vi "CRYO_MASTER_FULL.vi"() -> ()   [LabVIEW 2017]
uses:
  LSI218Data.lvclass
  LSI336Data.lvclass
  USBData.lvclass
  6240AData.lvclass
  <vilib>/DAQmx/create/channels.llb/DAQmx Create Channel (DO-Digital Output).vi
  <vilib>/DAQmx/miscellaneous.llb/DAQmx Fill In Error Info.vi
  <vilib>/DAQmx/create/channels.llb/DAQmx Create Channel (AO-Voltage-Basic).vi
  <vilib>/express/express arith-compare/Formula/XNode/ExpressFormulaBlockNode.xnode
  <vilib>/Analysis/NI_AALBase.lvlib
panel:
  in  "Frontpanel screenshots":bool
  in  "Screenshots interval":i64=3605
  in  "Record interval":i64=10
  out "Cycle #":u32=332
  in  "Measurement Interval (s)":dbl=1.0
  in  "Stop Button":bool
  in  "?":T1(tab)=enum."(Place holder)"
  in  "Base Path (screenshots)":path=path "C:/LabVIEW/DATA/Precooling"
  out "error out (USB6210/6218 AOUT)":errorcluster
  in  "AOUT 1 Label":string="KIKUSUI_I"
  in  "AOUT 0 Label":string="KIKUSUI_V"
  in  "DOUT Labels":string[](array[string])=["D_V1_NO", "D_V2_NC", "D_CV1"]
  in  "AOUT for Current CTRL":tag="Dev1/ao1"
  in  "AOUT For Voltage CTRL":tag="Dev1/ao0"
  out "AO task out":refnum<k21>="20200912_112449_AO"
  in  "Analog Out ON?":bool=TRUE
  in  "InstName (USB6218)":string="USB6218"
  in  "USB6218 Config":T2(array[cluster])=[{"Label"="F_1", "FileFormat"="%5.5f", "Active?"=TRUE, "Physical CH"="Dev1/ai0", " terminal\n type"=10083, "ConversionType"={"Type"=enum."SimpleProp", "ConversionParameters"=[0.0, 5.0, 0.0, 500.0]}, "VoltageLimits"=[0.0, 5.0]}, {"Label"="F_2", "FileFormat"="%5.5f", "Active?"=TRUE, "Physical CH"="Dev1/ai1", " terminal\n type"=10083, "ConversionType"={"Type"=enum."SimpleProp", "ConversionParameters"=[0.0, 5.0, 0.0, 200.0]}, "VoltageLimits"=[0.0, 5.0]}, {"Label"="F_3", "FileFormat"="%5.5f", "Active?"=TRUE, "Physical CH"="Dev1/ai2", " terminal\n type"=10083, "ConversionType"={"Type"=enum."SimpleProp", "ConversionParameters"=[0.0, 5.0, 0.0, 200.0]}, "VoltageLimits"=[0.0, 5.0]}, {"Label"="F_4", "FileFormat"="%5.5f", "Active?"=TRUE, "Physical CH"="Dev1/ai3", " terminal\n type"=10083, "ConversionType"={"Type"=enum."SimpleProp", "ConversionParameters"=[0.0, 5.0, 0.0, 500.0]}, "VoltageLimits"=[0.0, 5.0]}, {"Label"="F_5", "FileFormat"="%5.5f", "Active?"=TRUE, "Physical CH"="Dev1/ai4", " terminal\n type"=10083, "ConversionType"={"Type"=enum."SimpleProp", "ConversionParameters"=[0.0, 5.0, 0.0, 500.0]}, "VoltageLimits"=[0.0, 5.0]}, {"Label"="I_CV", "FileFormat"="%3.5f", "Active?"=TRUE, "Physical CH"="Dev1/ai5", " terminal\n type"=10083, "ConversionType"={"Type"=enum."SimpleProp", "ConversionParameters"=[0.0, 10.0, 0.0, 2000.0]}, "VoltageLimits"=[0.0, 10.0]}, {"Label"="CV1_answer", "FileFormat"="%3.5f", "Active?"=TRUE, "Physical CH"="Dev1/ai6", " terminal\n type"=10083, "ConversionType"={"Type"=enum."SimpleProp", "ConversionParameters"=[1.0, 5.0, 0.0, 100.0]}, "VoltageLimits"=[0.0, 5.0]}] {"terminal\n type" items=["Default"=-1, "RSE"=10083, "NRSE"=10078, "Differential"=10106, "Pseudodifferential"=12529]}
  out "error out (USB6218)":errorcluster
  out "error out (USB6210/6218 DOUT)":errorcluster
  out "DOUT task out":refnum<k21>="20200912_112449_DO"
  in  "DOUT Physical CH":tag[](array[tag])=["Dev1/port1/line0", "Dev1/port1/line1", "Dev1/port1/line2"]
  in  "Digital Out ON?":bool=TRUE
  in  "USB6210 Config":T2(array[cluster])=[{"Label"="P_ins", "FileFormat"="%5.5e", "Active?"=TRUE, "Physical CH"="Dev2/ai0", " terminal\n type"=10083, "ConversionType"={"Type"=enum."CC-10_LOG", "ConversionParameters"=[0.5, 9.0, 0.0, 1.0]}, "VoltageLimits"=[0.0, 10.0]}, {"Label"="P_4Kres", "FileFormat"="%5.5e", "Active?"=TRUE, "Physical CH"="Dev2/ai1", " terminal\n type"=10083, "ConversionType"={"Type"=enum."SimpleProp", "ConversionParameters"=[1.0, 5.0, 0.0, 200000.0]}, "VoltageLimits"=[0.0, 5.0]}, {"Label"="P_3HeIN", "FileFormat"="%5.5e", "Active?"=TRUE, "Physical CH"="Dev2/ai2", " terminal\n type"=10083, "ConversionType"={"Type"=enum."SimpleProp", "ConversionParameters"=[1.0, 5.0, 0.0, 200000.0]}, "VoltageLimits"=[0.0, 5.0]}, {"Label"="P_SldRTN", "FileFormat"="%5.5e", "Active?"=TRUE, "Physical CH"="Dev2/ai3", " terminal\n type"=10083, "ConversionType"={"Type"=enum."SimpleProp", "ConversionParameters"=[1.0, 5.0, 0.0, 200000.0]}, "VoltageLimits"=[0.0, 5.0]}, {"Label"="P_3Hepot", "FileFormat"="%5.5e", "Active?"=TRUE, "Physical CH"="Dev2/ai4", " terminal\n type"=10083, "ConversionType"={"Type"=enum."SimpleProp", "ConversionParameters"=[0.0, 10.0, 0.0, 133320.0]}, "VoltageLimits"=[0.0, 10.0]}, {"Label"="P_1Kpot", "FileFormat"="%5.5e", "Active?"=TRUE, "Physical CH"="Dev2/ai5", " terminal\n type"=10083, "ConversionType"={"Type"=enum."SimpleProp", "ConversionParameters"=[0.0, 10.0, 0.0, 133320.0]}, "VoltageLimits"=[0.0, 10.0]}, {"Label"="P_Dewar", "FileFormat"="%5.5e", "Active?"=TRUE, "Physical CH"="Dev2/ai6", " terminal\n type"=10083, "ConversionType"={"Type"=enum."SimpleProp", "ConversionParameters"=[1.0, 5.0, 0.0, 200000.0]}, "VoltageLimits"=[0.0, 5.0]}, {"Label"="DP_HEX4", "FileFormat"="%5.5e", "Active?"=TRUE, "Physical CH"="Dev2/ai7", " terminal\n type"=10083, "ConversionType"={"Type"=enum."SimpleProp", "ConversionParameters"=[1.0, 5.0, 0.0, 1000.0]}, "VoltageLimits"=[0.0, 5.0]}, {"Label"="DP_HEX5", "FileFormat"="%5.5e", "Active?"=TRUE, "Physical CH"="Dev2/ai8", " terminal\n type"=10083, "ConversionType"={"Type"=enum."SimpleProp", "ConversionParameters"=[1.0, 5.0, 0.0, 20000.0]}, "VoltageLimits"=[0.0, 5.0]}, {"Label"="L1", "FileFormat"="%5.5f", "Active?"=TRUE, "Physical CH"="Dev2/ai9", " terminal\n type"=10083, "ConversionType"={"Type"=enum."SimpleProp", "ConversionParameters"=[0.0, 10.0, 0.0, 100.0]}, "VoltageLimits"=[0.0, 10.0]}, {"Label"="L2-1", "FileFormat"="%5.5f", "Active?"=TRUE, "Physical CH"="Dev2/ai10", " terminal\n type"=10083, "ConversionType"={"Type"=enum."SimpleProp", "ConversionParameters"=[0.0, 10.0, 0.0, 100.0]}, "VoltageLimits"=[0.0, 10.0]}, {"Label"="L2-2", "FileFormat"="%5.5f", "Active?"=TRUE, "Physical CH"="Dev2/ai11", " terminal\n type"=10083, "ConversionType"={"Type"=enum."SimpleProp", "ConversionParameters"=[0.0, 10.0, 0.0, 100.0]}, "VoltageLimits"=[0.0, 10.0]}, {"Label"="L3", "FileFormat"="%5.5f", "Active?"=TRUE, "Physical CH"="Dev2/ai12", " terminal\n type"=10083, "ConversionType"={"Type"=enum."SimpleProp", "ConversionParameters"=[0.0, 10.0, 0.0, 100.0]}, "VoltageLimits"=[0.0, 10.0]}] {"terminal\n type" items=["Default"=-1, "RSE"=10083, "NRSE"=10078, "Differential"=10106, "Pseudodifferential"=12529]}
  in  "RUN identifier":string="PreCooling"
  in  "Base Path":path=path "C:/LabVIEW/DATA/Precooling"
  in  "InstName (USB6210)":string="USB6210"
  out "error out (USB6210)":errorcluster
  out "File Refn USB AO":refnum<file>
  out "File Refn USB DO":refnum<file>
  out "error out (LSI336)":errorcluster
  in  "InstName (LSI336)":string="LSI336"
  in  "FileFormat (336)":string="%4.4f"
  in  "LSI336Settings(X,Y)":T3(array[cluster])=[{"LSIName"="LSi336X", "Labels"=["T1K3-1", "T1K3-2", "T3He5", "T3He8"], "SensorLocations"=[enum."T1K3-1", enum."T1K3-2", enum."T3He5", enum."T3He8"], "Active?"=TRUE, "VISA res. name"="GPIB0::6::INSTR"}, {"LSIName"="LSi336Y", "Labels"=["T3He6-1", "T3He6-2", "T3He7-1", "T3He7-2"], "SensorLocations"=[enum."T3He6-1", enum."T3He6-2", enum."T3He7-1", enum."T3He7-2"], "Active?"=TRUE, "VISA res. name"="GPIB0::2::INSTR"}]
  in  "FileFormat (218)":string="%4.4f"
  in  "InstName (LSI218)":string="LSI218"
  in  "LSI218Settings(A-F)":T3(array[cluster])=[{"LSIName"="LSI218A", "Labels"=["T3He10", "T3He1-1", "TTH3", "TTH4", "TTH1", "TTH2", "T4He1", "T1K1"], "SensorLocations"=[enum."T3He10", enum."T3He1-1", enum."TTH3", enum."TTH4", enum."TTH1", enum."TTH2", enum."T4He1", enum."T1K1"], "Active?"=TRUE, "VISA res. name"="GPIB0::7::INSTR"}, {"LSIName"="LSI218B", "Labels"=["N.C.", "N.C.", "N.C.", "N.C.", "T3He2-1", "T3He2-2", "T3He3", "T3He1-4"], "SensorLocations"=[enum."N.C.", enum."N.C.", enum."N.C.", enum."N.C.", enum."T3He2-1", enum."T3He2-2", enum."T3He3", enum."T3He1-4"], "Active?"=TRUE, "VISA res. name"="GPIB0::4::INSTR"}, {"LSIName"="LSI218C", "Labels"=["T4He3-1", "T4He3-2", "T4He3-3", "T4He3-4", "T4He2-1", "T4He2-2", "T4He4", "T4He5"], "SensorLocations"=[enum."T4He3-1", enum."T4He3-2", enum."T4He3-3", enum."T4He3-4", enum."T4He2-1", enum."T4He2-2", enum."T4He4", enum."T4He5"], "Active?"=TRUE, "VISA res. name"="GPIB0::3::INSTR"}, {"LSIName"="LSI218D", "Labels"=["T4He6", "T4He9", "T3He1-2", "T3He1-3", "T4He7", "T4He8", "T4He10", "T1K6"], "SensorLocations"=[enum."T4He6", enum."T4He9", enum."T3He1-2", enum."T3He1-3", enum."T4He7", enum."T4He8", enum."T4He10", enum."T1K6"], "Active?"=TRUE, "VISA res. name"="GPIB0::5::INSTR"}, {"LSIName"="LSI218E", "Labels"=["TIP1", "N.C.", "TIP2", "N.C.", "TIP3", "TIP4", "TIP5", "N.C."], "SensorLocations"=[enum."TIP1", enum."N.C.", enum."TIP2", enum."N.C.", enum."TIP3", enum."TIP4", enum."TIP5", enum."N.C."], "Active?"=TRUE, "VISA res. name"="GPIB0::11::INSTR"}, {"LSIName"="LSI218F", "Labels"=["T1K2", "T1K4", "T1K5", "T3He4", "T3He9", "TIP6", "N.C.", "N.C."], "SensorLocations"=[enum."T1K2", enum."T1K4", enum."T1K5", enum."T3He4", enum."T3He9", enum."TIP6", enum."N.C.", enum."N.C."], "Active?"=TRUE, "VISA res. name"="GPIB0::8::INSTR"}]
  out "error out (LSI218)":errorcluster
  out "Graph 3":T4(graph) caption="XY Graph"
  out "Graph 1":T4(graph)=[{"TimeArray"=[timestamp(3682722291.26542 s since 1904-01-01), timestamp(3682722291.60303 s since 1904-01-01), timestamp(3682722291.9037905 s since 1904-01-01), timestamp(3682722292.2130303 s since 1904-01-01), timestamp(3682722293.6093 s since 1904-01-01), timestamp(3682722293.911434 s since 1904-01-01), timestamp(3682722294.215163 s since 1904-01-01), timestamp(3682722294.522572 s since 1904-01-01), timestamp(3682722294.8441634 s since 1904-01-01), timestamp(3682722295.1448545 s since 1904-01-01), timestamp(3682722295.44568 s since 1904-01-01), timestamp(3682722295.7512665 s since 1904-01-01), timestamp(3682722296.071016 s since 1904-01-01), timestamp(3682722297.4895544 s since 1904-01-01), timestamp(3682722298.3582816 s since 1904-01-01), timestamp(3682722298.6583776 s since 1904-01-01), timestamp(3682722298.976703 s since 1904-01-01), timestamp(3682722299.303491 s since 1904-01-01), timestamp(3682722299.6028943 s since 1904-01-01), timestamp(3682722299.9109864 s since 1904-01-01), timestamp(3682722301.2943215 s since 1904-01-01), timestamp(3682722302.439338 s since 1904-01-01), timestamp(3682722302.84283 s since 1904-01-01), timestamp(3682722303.976296 s since 1904-01-01), timestamp(3682722304.298886 s since 1904-01-01), timestamp(3682722304.6146727 s since 1904-01-01), timestamp(3682722304.9304714 s since 1904-01-01), timestamp(3682722306.0827866 s since 1904-01-01), timestamp(3682722306.400269 s since 1904-01-01), timestamp(3682722306.701908 s since 1904-01-01), timestamp(3682722307.01266 s since 1904-01-01), timestamp(3682722307.3139567 s since 1904-01-01), timestamp(3682722307.617281 s since 1904-01-01), timestamp(3682722307.9324656 s since 1904-01-01), timestamp(3682722308.2477794 s since 1904-01-01), timestamp(3682722309.066163 s since 1904-01-01), timestamp(3682722309.3965664 s since 1904-01-01), timestamp(3682722309.7003713 s since 1904-01-01), timestamp(3682722310.0011826 s since 1904-01-01), timestamp(3682722310.3316903 s since 1904-01-01), timestamp(3682722310.6338625 s since 1904-01-01), timestamp(3682722311.8390217 s since 1904-01-01), timestamp(3682722312.147876 s since 1904-01-01), timestamp(3682722312.4494967 s since 1904-01-01), timestamp(3682722312.760971 s since 1904-01-01), timestamp(3682722313.065274 s since 1904-01-01), timestamp(3682722313.3656464 s since 1904-01-01), timestamp(3682722313.6989264 s since 1904-01-01), timestamp(3682722314.00116 s since 1904-01-01), timestamp(3682722314.3316183 s since 1904-01-01), timestamp(3682722314.632463 s since 1904-01-01), timestamp(3682722314.9485526 s since 1904-01-01), timestamp(3682722315.2606983 s since 1904-01-01), timestamp(3682722315.5799346 s since 1904-01-01), timestamp(3682722315.9180913 s since 1904-01-01), timestamp(3682722316.2203927 s since 1904-01-01), timestamp(3682722316.5203104 s since 1904-01-01), timestamp(3682722316.8202634 s since 1904-01-01), timestamp(3682722318.055342 s since 1904-01-01), timestamp(3682722318.3566217 s since 1904-01-01), timestamp(3682722318.67011 s since 1904-01-01), timestamp(3682722318.979581 s since 1904-01-01), timestamp(3682722319.3166094 s since 1904-01-01), timestamp(3682722319.6308255 s since 1904-01-01), timestamp(3682722319.948837 s since 1904-01-01), timestamp(3682722320.2572136 s since 1904-01-01), timestamp(3682722320.599373 s since 1904-01-01), timestamp(3682722320.919993 s since 1904-01-01), timestamp(3682722321.220749 s since 1904-01-01), timestamp(3682722321.5287714 s since 1904-01-01), timestamp(3682722321.8486905 s since 1904-01-01), timestamp(3682722322.1527696 s since 1904-01-01), timestamp(3682722322.4684625 s since 1904-01-01), timestamp(3682722322.768717 s since 1904-01-01), timestamp(3682722323.0695057 s since 1904-01-01), timestamp(3682722323.3691983 s since 1904-01-01), timestamp(3682722323.699779 s since 1904-01-01), timestamp(3682722324.00254 s since 1904-01-01), timestamp(3682722324.302169 s since 1904-01-01), timestamp(3682722324.6159334 s since 1904-01-01), timestamp(3682722324.9335217 s since 1904-01-01), timestamp(3682722325.2332306 s since 1904-01-01), timestamp(3682722325.5330367 s since 1904-01-01), timestamp(3682722325.833967 s since 1904-01-01), timestamp(3682722326.1509953 s since 1904-01-01), timestamp(3682722326.4644866 s since 1904-01-01), timestamp(3682722326.767284 s since 1904-01-01), timestamp(3682722327.067716 s since 1904-01-01), timestamp(3682722327.3710494 s since 1904-01-01), timestamp(3682722327.6760697 s since 1904-01-01), timestamp(3682722328.0013742 s since 1904-01-01), timestamp(3682722328.3049417 s since 1904-01-01), timestamp(3682722328.605616 s since 1904-01-01), timestamp(3682722328.915824 s since 1904-01-01), timestamp(3682722329.2197704 s since 1904-01-01), timestamp(3682722329.533479 s since 1904-01-01), timestamp(3682722329.8484006 s since 1904-01-01), timestamp(3682722330.1537294 s since 1904-01-01), timestamp(3682722330.4685154 s since 1904-01-01), timestamp(3682722330.7689 s since 1904-01-01), timestamp(3682722331.0704536 s since 1904-01-01), timestamp(3682722331.371037 s since 1904-01-01), timestamp(3682722331.701168 s since 1904-01-01), timestamp(3682722332.003296 s since 1904-01-01), timestamp(3682722332.3189206 s since 1904-01-01), timestamp(3682722332.6204143 s since 1904-01-01), timestamp(3682722332.9201455 s since 1904-01-01), timestamp(3682722333.222704 s since 1904-01-01), timestamp(3682722333.5307713 s since 1904-01-01), timestamp(3682722333.850218 s since 1904-01-01), timestamp(3682722334.1687818 s since 1904-01-01), timestamp(3682722334.50168 s since 1904-01-01), timestamp(3682722334.8162985 s since 1904-01-01), timestamp(3682722335.1198063 s since 1904-01-01), timestamp(3682722335.433464 s since 1904-01-01), timestamp(3682722335.754174 s since 1904-01-01), timestamp(3682722336.065685 s since 1904-01-01), timestamp(3682722336.3676305 s since 1904-01-01), timestamp(3682722336.678262 s since 1904-01-01), timestamp(3682722337.00354 s since 1904-01-01), timestamp(3682722337.305712 s since 1904-01-01), timestamp(3682722337.6067743 s since 1904-01-01), timestamp(3682722337.906976 s since 1904-01-01), timestamp(3682722338.207723 s since 1904-01-01), timestamp(3682722338.5086007 s since 1904-01-01), timestamp(3682722338.8327622 s since 1904-01-01), timestamp(3682722339.15376 s since 1904-01-01), timestamp(3682722339.4660926 s since 1904-01-01), timestamp(3682722339.7669024 s since 1904-01-01), timestamp(3682722340.0687447 s since 1904-01-01), timestamp(3682722340.3689446 s since 1904-01-01), timestamp(3682722340.669699 s since 1904-01-01), timestamp(3682722340.971668 s since 1904-01-01), timestamp(3682722341.2735777 s since 1904-01-01), timestamp(3682722341.5808673 s since 1904-01-01), timestamp(3682722341.9035897 s since 1904-01-01), timestamp(3682722342.2187233 s since 1904-01-01), timestamp(3682722342.519108 s since 1904-01-01), timestamp(3682722342.8346863 s since 1904-01-01), timestamp(3682722343.148861 s since 1904-01-01), timestamp(3682722343.453436 s since 1904-01-01), timestamp(3682722343.7687 s since 1904-01-01), timestamp(3682722344.0703554 s since 1904-01-01), timestamp(3682722344.3702574 s since 1904-01-01), timestamp(3682722344.6709967 s since 1904-01-01), timestamp(3682722345.753763 s since 1904-01-01), timestamp(3682722346.088916 s since 1904-01-01), timestamp(3682722346.411592 s since 1904-01-01), timestamp(3682722346.713475 s since 1904-01-01), timestamp(3682722347.054868 s since 1904-01-01), timestamp(3682722347.366645 s since 1904-01-01), timestamp(3682722347.6674814 s since 1904-01-01), timestamp(3682722348.1936336 s since 1904-01-01), timestamp(3682722348.7083697 s since 1904-01-01), timestamp(3682722349.007952 s since 1904-01-01), timestamp(3682722349.320494 s since 1904-01-01), timestamp(3682722349.6215 s since 1904-01-01), timestamp(3682722349.921623 s since 1904-01-01), timestamp(3682722350.2236137 s since 1904-01-01), timestamp(3682722350.525284 s since 1904-01-01), timestamp(3682722350.8256655 s since 1904-01-01), timestamp(3682722351.126511 s since 1904-01-01), timestamp(3682722351.434491 s since 1904-01-01), timestamp(3682722351.75064 s since 1904-01-01), timestamp(3682722352.0507593 s since 1904-01-01), timestamp(3682722352.3531384 s since 1904-01-01), timestamp(3682722352.6707296 s since 1904-01-01), timestamp(3682722352.9734945 s since 1904-01-01), timestamp(3682722353.2847114 s since 1904-01-01), timestamp(3682722353.600667 s since 1904-01-01), timestamp(3682722353.906944 s since 1904-01-01), timestamp(3682722354.206764 s since 1904-01-01), timestamp(3682722354.518809 s since 1904-01-01), timestamp(3682722354.8189607 s since 1904-01-01), timestamp(3682722355.138008 s since 1904-01-01), timestamp(3682722355.4524865 s since 1904-01-01), timestamp(3682722355.7545385 s since 1904-01-01), timestamp(3682722356.0694222 s since 1904-01-01), timestamp(3682722356.371631 s since 1904-01-01), timestamp(3682722356.671609 s since 1904-01-01), timestamp(3682722356.972576 s since 1904-01-01), timestamp(3682722357.2745256 s since 1904-01-01), timestamp(3682722357.5746017 s since 1904-01-01), timestamp(3682722357.9027176 s since 1904-01-01), timestamp(3682722358.220368 s since 1904-01-01), timestamp(3682722358.536658 s since 1904-01-01), timestamp(3682722358.8382 s since 1904-01-01), timestamp(3682722359.139381 s since 1904-01-01), timestamp(3682722359.4571586 s since 1904-01-01), timestamp(3682722359.7668686 s since 1904-01-01), timestamp(3682722360.068324 s since 1904-01-01), timestamp(3682722360.3683295 s since 1904-01-01), timestamp(3682722361.6878138 s since 1904-01-01), timestamp(3682722363.114297 s since 1904-01-01), timestamp(3682722363.413959 s since 1904-01-01), timestamp(3682722363.7199144 s since 1904-01-01), timestamp(3682722364.037248 s since 1904-01-01), timestamp(3682722364.3384633 s since 1904-01-01), timestamp(3682722364.6368146 s since 1904-01-01), timestamp(3682722364.936756 s since 1904-01-01), timestamp(3682722365.3525553 s since 1904-01-01), timestamp(3682722365.6523194 s since 1904-01-01), timestamp(3682722365.953843 s since 1904-01-01), timestamp(3682722366.259619 s since 1904-01-01), timestamp(3682722366.5631113 s since 1904-01-01), timestamp(3682722366.868568 s since 1904-01-01), timestamp(3682722367.202246 s since 1904-01-01), timestamp(3682722367.518932 s since 1904-01-01), timestamp(3682722367.835234 s since 1904-01-01), timestamp(3682722368.151437 s since 1904-01-01), timestamp(3682722368.455229 s since 1904-01-01), timestamp(3682722368.7568297 s since 1904-01-01), timestamp(3682722369.070481 s since 1904-01-01), timestamp(3682722369.3724856 s since 1904-01-01), timestamp(3682722369.674691 s since 1904-01-01), timestamp(3682722369.9750576 s since 1904-01-01), timestamp(3682722370.2769585 s since 1904-01-01), timestamp(3682722370.5767703 s since 1904-01-01), timestamp(3682722371.761378 s since 1904-01-01), timestamp(3682722372.0615153 s since 1904-01-01), timestamp(3682722372.36768 s since 1904-01-01), timestamp(3682722372.6716857 s since 1904-01-01), timestamp(3682722372.9741178 s since 1904-01-01), timestamp(3682722373.2752647 s since 1904-01-01), timestamp(3682722373.5791826 s since 1904-01-01), timestamp(3682722373.8855314 s since 1904-01-01), timestamp(3682722374.2075486 s since 1904-01-01), timestamp(3682722374.5190463 s since 1904-01-01), timestamp(3682722374.822685 s since 1904-01-01), timestamp(3682722375.135455 s since 1904-01-01), timestamp(3682722375.4391584 s since 1904-01-01), timestamp(3682722375.753536 s since 1904-01-01), timestamp(3682722376.0574703 s since 1904-01-01), timestamp(3682722376.3707743 s since 1904-01-01), timestamp(3682722376.671406 s since 1904-01-01), timestamp(3682722376.973929 s since 1904-01-01), timestamp(3682722377.275672 s since 1904-01-01), timestamp(3682722377.903696 s since 1904-01-01), timestamp(3682722378.3413343 s since 1904-01-01), timestamp(3682722378.6628866 s since 1904-01-01), timestamp(3682722378.971062 s since 1904-01-01), timestamp(3682722379.272179 s since 1904-01-01), timestamp(3682722379.574565 s since 1904-01-01), timestamp(3682722379.8750696 s since 1904-01-01), timestamp(3682722380.1758666 s since 1904-01-01), timestamp(3682722380.4776945 s since 1904-01-01), timestamp(3682722380.785676 s since 1904-01-01), timestamp(3682722381.101816 s since 1904-01-01), timestamp(3682722382.102351 s since 1904-01-01), timestamp(3682722383.1034727 s since 1904-01-01), timestamp(3682722384.1039815 s since 1904-01-01), timestamp(3682722385.1047606 s since 1904-01-01), timestamp(3682722386.103784 s since 1904-01-01), timestamp(3682722387.1065063 s since 1904-01-01), timestamp(3682722388.105764 s since 1904-01-01), timestamp(3682722389.1080866 s since 1904-01-01), timestamp(3682722392.018273 s since 1904-01-01), timestamp(3682722393.0827537 s since 1904-01-01), timestamp(3682722394.4643016 s since 1904-01-01), timestamp(3682722395.465176 s since 1904-01-01), timestamp(3682722396.4664454 s since 1904-01-01), timestamp(3682722398.0099154 s since 1904-01-01), timestamp(3682722399.010983 s since 1904-01-01), timestamp(3682722400.0118704 s since 1904-01-01), timestamp(3682722401.013437 s since 1904-01-01), timestamp(3682722402.015486 s since 1904-01-01), timestamp(3682722403.0175056 s since 1904-01-01), timestamp(3682722404.01802 s since 1904-01-01), timestamp(3682722405.0194936 s since 1904-01-01), timestamp(3682722406.0196953 s since 1904-01-01), timestamp(3682722407.0214458 s since 1904-01-01), timestamp(3682722408.0222106 s since 1904-01-01), timestamp(3682722409.023329 s since 1904-01-01), timestamp(3682722410.0232754 s since 1904-01-01), timestamp(3682722411.024305 s since 1904-01-01), timestamp(3682722412.0254784 s since 1904-01-01), timestamp(3682722413.024827 s since 1904-01-01), timestamp(3682722414.026385 s since 1904-01-01), timestamp(3682722415.0269694 s since 1904-01-01), timestamp(3682722416.029292 s since 1904-01-01), timestamp(3682722417.03152 s since 1904-01-01), timestamp(3682722418.031929 s since 1904-01-01), timestamp(3682722419.03179 s since 1904-01-01), timestamp(3682722420.032112 s since 1904-01-01), timestamp(3682722421.0339622 s since 1904-01-01), timestamp(3682722422.032736 s since 1904-01-01), timestamp(3682722423.0335274 s since 1904-01-01), timestamp(3682722424.032856 s since 1904-01-01), timestamp(3682722425.0344257 s since 1904-01-01), timestamp(3682722426.0349946 s since 1904-01-01), timestamp(3682722427.1135817 s since 1904-01-01), timestamp(3682722428.113387 s since 1904-01-01), timestamp(3682722429.122927 s since 1904-01-01), timestamp(3682722430.122795 s since 1904-01-01), timestamp(3682722431.1243224 s since 1904-01-01), timestamp(3682722432.1657104 s since 1904-01-01), timestamp(3682722433.5395536 s since 1904-01-01), timestamp(3682722434.5393767 s since 1904-01-01), timestamp(3682722435.5397377 s since 1904-01-01), timestamp(3682722436.541572 s since 1904-01-01), timestamp(3682722437.8902345 s since 1904-01-01), timestamp(3682722438.889765 s since 1904-01-01), timestamp(3682722439.890742 s since 1904-01-01), timestamp(3682722440.8925166 s since 1904-01-01), timestamp(3682722441.8928022 s since 1904-01-01), timestamp(3682722442.8935113 s since 1904-01-01), timestamp(3682722443.9465127 s since 1904-01-01), timestamp(3682722444.946664 s since 1904-01-01), timestamp(3682722445.946266 s since 1904-01-01), timestamp(3682722446.9467134 s since 1904-01-01), timestamp(3682722447.9487176 s since 1904-01-01), timestamp(3682722448.9498606 s since 1904-01-01), timestamp(3682722449.9507394 s since 1904-01-01), timestamp(3682722451.010164 s since 1904-01-01), timestamp(3682722452.011107 s since 1904-01-01), timestamp(3682722453.0121975 s since 1904-01-01), timestamp(3682722454.014766 s since 1904-01-01), timestamp(3682722455.129564 s since 1904-01-01), timestamp(3682722456.129246 s since 1904-01-01), timestamp(3682722457.1289473 s since 1904-01-01), timestamp(3682722458.129476 s since 1904-01-01), timestamp(3682722459.129673 s since 1904-01-01), timestamp(3682722460.1309032 s since 1904-01-01), timestamp(3682722461.1332126 s since 1904-01-01), timestamp(3682722462.133421 s since 1904-01-01), timestamp(3682722463.1336327 s since 1904-01-01), timestamp(3682722464.1343303 s since 1904-01-01), timestamp(3682722465.134672 s since 1904-01-01), timestamp(3682722466.136228 s since 1904-01-01), timestamp(3682722467.1370697 s since 1904-01-01), timestamp(3682722468.136828 s since 1904-01-01), timestamp(3682722469.4057984 s since 1904-01-01)], "DataArray"=array[332 elements]}] caption="XY Graph"
  in  "FIle suffix 4":string="Graph4"
  in  "Take Screenshot! 4":bool
  in  "FIle suffix 3":string="Graph3"
  in  "Take Screenshot! 3":bool
  in  "FIle suffix 2":string="Graph2"
  in  "Take Screenshot! 2":bool
  in  "FIle suffix 1":string="Graph1"
  in  "Take Screenshot! 1":bool
  in  "log/linear 2":bool
  in  "Tab Control 2":T5(tab)
  in  "Plot selecter (USB6210)\n    1      2     3     4":bool[][](array[boolean])=[[FALSE, FALSE, TRUE, FALSE], [FALSE, FALSE, TRUE, FALSE], [FALSE, FALSE, TRUE, FALSE], [FALSE, FALSE, TRUE, FALSE], [FALSE, FALSE, TRUE, FALSE], [FALSE, FALSE, TRUE, FALSE], [TRUE, FALSE, FALSE, FALSE], [FALSE, FALSE, TRUE, FALSE], [FALSE, FALSE, TRUE, FALSE], [FALSE, FALSE, FALSE, TRUE], [FALSE, FALSE, FALSE, TRUE], [FALSE, FALSE, FALSE, TRUE], [FALSE, FALSE, FALSE, TRUE], [FALSE, FALSE, FALSE, FALSE], [FALSE, FALSE, FALSE, FALSE], [FALSE, FALSE, FALSE, FALSE]]
  out "All Labels (USB6210)":string[](array[string])=["P_ins", "P_4Kres", "P_3HeIN", "P_SldRTN", "P_3Hepot", "P_1Kpot", "P_Dewar", "DP_HEX4", "DP_HEX5", "L1", "L2-1", "L2-2", "L3"]
  out "Last Data \n(USB6210)":dbl[](array[numeric])=[0.00028560714995192756, 101440.7952285239, 101333.90751417259, 101019.82209454894, 100881.91242915385, 101237.87956202377, 101521.37230060964, -12.315450307474885, 24.853264932898078, 100.08478128736311, 0.1573062383944258, 0.10338097393213444, 0.16585536566079262] format="%#_6e"
  out "Time of Last Measurement (USB6210)":timestamp=timestamp(3682722469.4057984 s since 1904-01-01)
  out "USB6210 Status":T6(ring)=enum."Ready"
  out "Last Vol\n(USB6210)":dbl[](array[numeric])=[5.72788453773169, 3.028815904570478, 3.026678150283452, 3.020396441890979, 7.566900122198758, 7.593600327184501, 3.030427446012193, 0.9507381987701005, 1.0049706529865796, 10.00847812873631, 0.01573062383944258, 0.010338097393213444, 0.01658553656607926] format="%_5f"
  out "Time of Last Measurement (USB6218)":timestamp=timestamp(3682722469.4107466 s since 1904-01-01)
  out "USB6218 Status":T6(ring)=enum."Ready"
  out "Last Vol \n(USB6218)":dbl[](array[numeric])=[0.1161921013139235, 0.004469645896882965, 0.00525873920597651, -0.08617745088139704, 0.3127420592396069, -0.00427246828913797, -0.0001005194945602722] format="%_5f"
  out "Last Data \n(USB6218)":dbl[](array[numeric])=[11.61921013139235, 0.1787858358753186, 0.21034956823906042, -8.617745088139705, 31.27420592396069, -0.854493657827594, -25.002512987364007] format="%#_6e"
  out "All Labels (USB6218)":string[](array[string])=["F_1", "F_2", "F_3", "F_4", "F_5", "I_CV", "CV1_answer"]
  in  "Plot selecter (USB6218)\n    1      2     3     4":bool[][](array[boolean])=[[FALSE, FALSE, TRUE, FALSE], [FALSE, FALSE, TRUE, FALSE], [FALSE, FALSE, TRUE, FALSE], [FALSE, FALSE, TRUE, FALSE], [FALSE, FALSE, TRUE, FALSE], [FALSE, FALSE, TRUE, FALSE], [FALSE, FALSE, FALSE, FALSE], [FALSE, FALSE, TRUE, FALSE], [FALSE, FALSE, TRUE, FALSE], [FALSE, FALSE, FALSE, TRUE], [FALSE, FALSE, FALSE, TRUE], [FALSE, FALSE, FALSE, TRUE], [FALSE, FALSE, FALSE, TRUE], [FALSE, FALSE, FALSE, FALSE], [FALSE, FALSE, FALSE, FALSE], [FALSE, FALSE, FALSE, FALSE]]
  out "Time of Last Measurement (LSI218)":timestamp=timestamp(3682722469.4057984 s since 1904-01-01)
  out "LSI218 Status":T7(ring)=enum."Measuring"
  out "Last Data \nLSI218 (1)":dbl[](array[numeric])=[285.45, 290.71, 245.43, 252.59, 172.54, 177.97, 71.656, 129.11, 30.0, 0.0, 0.0, 0.0, 207.67, 199.47, 131.72, 290.16, 292.6, 292.74, 292.31, 292.37, 207.68, 204.03, 195.11, 188.36]
  out "Labels LSI218 (1)":string[](array[string])=["T3He10", "T3He1-1", "TTH3", "TTH4", "TTH1", "TTH2", "T4He1", "T1K1", "N.C.", "N.C.", "N.C.", "N.C.", "T3He2-1", "T3He2-2", "T3He3", "T3He1-4", "T4He3-1", "T4He3-2", "T4He3-3", "T4He3-4", "T4He2-1", "T4He2-2", "T4He4", "T4He5"]
  in  "Plot selecter LSI218(1)\n    1      2     3     4":bool[][](array[boolean])=[[FALSE, FALSE, FALSE, FALSE], [FALSE, FALSE, FALSE, FALSE], [FALSE, FALSE, FALSE, FALSE], [FALSE, FALSE, FALSE, FALSE], [FALSE, FALSE, FALSE, FALSE], [FALSE, FALSE, FALSE, FALSE], [FALSE, FALSE, FALSE, FALSE], [FALSE, FALSE, FALSE, FALSE], [FALSE, FALSE, FALSE, FALSE], [FALSE, FALSE, FALSE, FALSE], [FALSE, FALSE, FALSE, FALSE], [FALSE, FALSE, FALSE, FALSE], [FALSE, FALSE, FALSE, FALSE], [FALSE, FALSE, FALSE, FALSE], [FALSE, FALSE, FALSE, FALSE], [FALSE, FALSE, FALSE, FALSE], [FALSE, FALSE, FALSE, FALSE], [FALSE, FALSE, FALSE, FALSE], [FALSE, FALSE, FALSE, FALSE], [FALSE, FALSE, FALSE, FALSE], [FALSE, FALSE, FALSE, FALSE], [FALSE, FALSE, FALSE, FALSE], [FALSE, FALSE, FALSE, FALSE], [FALSE, FALSE, FALSE, FALSE]]
  out "Active?\n (1)":bool[](array[boolean])=[TRUE, TRUE, TRUE, TRUE, TRUE, TRUE, TRUE, TRUE, TRUE, TRUE, TRUE, TRUE, TRUE, TRUE, TRUE, TRUE, TRUE, TRUE, TRUE, TRUE, TRUE, TRUE, TRUE, TRUE]
  out "Labels LSI218 (2)":string[](array[string])=["T4He6", "T4He9", "T3He1-2", "T3He1-3", "T4He7", "T4He8", "T4He10", "T1K6", "TIP1", "N.C.", "TIP2", "N.C.", "TIP3", "TIP4", "TIP5", "N.C.", "T1K2", "T1K4", "T1K5", "T3He4", "T3He9", "TIP6", "N.C.", "N.C."]
  out "Active?\n(2)":bool[](array[boolean])=[TRUE, TRUE, TRUE, TRUE, TRUE, TRUE, TRUE, TRUE, TRUE, TRUE, TRUE, TRUE, TRUE, TRUE, TRUE, TRUE, TRUE, TRUE, TRUE, TRUE, TRUE, TRUE, TRUE, TRUE]
  out "Last Data \nLSI218 (2)":dbl[](array[numeric])=[194.01, 235.91, 290.83, 290.58, 249.16, 274.59, 270.4, 284.47, 279.27, 0.0, 231.46, 688.49, 199.72, 114.83, 153.45, 688.58, 126.48, 94.139, 102.89, 143.16, 127.49, 149.95, 0.433, 0.0]
  in  "Plot selecter LSI218(2)\n    1      2     3     4":bool[][](array[boolean])=[[FALSE, TRUE, FALSE, FALSE], [FALSE, TRUE, FALSE, FALSE], [FALSE, TRUE, FALSE, FALSE], [FALSE, TRUE, FALSE, FALSE], [FALSE, TRUE, FALSE, FALSE], [FALSE, TRUE, FALSE, FALSE], [FALSE, TRUE, FALSE, FALSE], [FALSE, TRUE, FALSE, FALSE], [FALSE, TRUE, FALSE, FALSE], [FALSE, TRUE, FALSE, FALSE], [FALSE, TRUE, FALSE, FALSE], [FALSE, FALSE, FALSE, FALSE], [FALSE, FALSE, FALSE, FALSE], [FALSE, FALSE, FALSE, FALSE], [FALSE, FALSE, FALSE, FALSE], [FALSE, FALSE, FALSE, FALSE], [FALSE, FALSE, FALSE, FALSE], [FALSE, FALSE, FALSE, FALSE], [FALSE, FALSE, FALSE, FALSE], [FALSE, FALSE, FALSE, FALSE], [FALSE, FALSE, FALSE, FALSE], [FALSE, FALSE, FALSE, FALSE], [FALSE, FALSE, FALSE, FALSE], [FALSE, FALSE, FALSE, FALSE]]
  in  "Plot selecter LSI336 \n     1      2     3     4":bool[][](array[boolean])=[[FALSE, TRUE, FALSE, FALSE], [FALSE, TRUE, FALSE, FALSE], [FALSE, TRUE, FALSE, FALSE], [FALSE, TRUE, FALSE, FALSE], [FALSE, TRUE, FALSE, FALSE], [FALSE, TRUE, FALSE, FALSE], [FALSE, TRUE, FALSE, FALSE], [FALSE, TRUE, FALSE, FALSE]]
  out "Time of Last Measurement (LSI336)":timestamp=timestamp(3682722469.4057984 s since 1904-01-01)
  out "Last Data \nLSI336":dbl[](array[numeric])=[95.4242, 95.2873, 133.19, 132.559, 138.289, 138.31, 138.239, 137.444]
  out "Active?\n(LSI336)":bool[](array[boolean])=[TRUE, TRUE, TRUE, TRUE, TRUE, TRUE, TRUE, TRUE]
  out "Labels LSI336":string[](array[string])=["T1K3-1", "T1K3-2", "T3He5", "T3He8", "T3He6-1", "T3He6-2", "T3He7-1", "T3He7-2"]
  out "LSI336 Status":T7(ring)=enum."Measuring"
  in  "log/linear 1":bool
  out "Graph 2":T4(graph) caption="XY Graph"
  out "Graph 4":T4(graph) caption="XY Graph"
  in  "log/linear 4":bool
  in  "log/linear 3":bool
  out "Fill (false)":bool=TRUE
  in  "Fill state":bool
  out "state 1 (false)":bool=TRUE
  out "state 1":bool
  out "state 2":bool
  out "state 2 (false)":bool=TRUE
  out "Status V2 CTRL":enum16{"Pressurize", "Release"}(ring)
  out "Status V1 CTRL":enum16{"Pressurize", "Release"}(ring)
  out "Lav (%)":dbl=-49199.19854911039 format="%0.2f"
  out "Lstd":dbl=554.7391446242465 format="%0.2f"
  out "Last N M.A. Levels":dbl[](array[numeric]) format="%_5e"
  out "Lstd history":dbl(graph)=554.7391446242465
  out "Lav history":dbl(graph)=-49199.19854911039
  out "Target Index (L)":i32=6
  in  "Auto Fll\nHe level label":string="P_Dewar"
  out "Target Index (P)":i32=6
  in  "Auto Fll\nDewar P. label":string="P_Dewar"
  out "He Level":T8(graph) caption="XY Graph"
  in  "P_safelimit_high (Pa)":dbl=300000.0 format="%_4e"
  in  "P_safelimit_low (Pa)":dbl=100.0 format="%_4e"
  in  "Auto Fill ON?":bool
  out "Pstd history":dbl(graph)=554.7391446242465
  out "Pav history":dbl(graph)=-49199.19854911039
  in  "Mov. Avg Interval":i64=4
  in  "V2 (N.C.)":bool
  in  "V1 (N.O.)":bool=TRUE
  in  "N for sampling":i64=7
  in  "L_low (%)":dbl=5000.0 format="%_3f"
  in  "L_high (%)":dbl=5000.0 format="%_3g"
  in  "P_2_low (Pa)":dbl=103000.0 format="%_4e"
  in  "P_1_low (Pa)":dbl=125000.0 format="%_4g"
  in  "P_2_high (Pa)":dbl=120000.0 format="%_4e"
  in  "P_1_high (Pa)":dbl=130000.0 format="%_4e"
  out "Dewar Pressure":T8(graph) caption="XY Graph"
  out "Last N M.A. Pressures":dbl[](array[numeric]) format="%_5e"
  out "Pav (Pa)":dbl=-49199.19854911039 format="%0.4e"
  out "Pstd":dbl=554.7391446242465 format="%0.4e"
  out "File Refn DewarCTRL":refnum<file>
  out "Error Out (Dewar CTRL":errorcluster
  in  "update current":bool
  out "USB AOUT":dbl[](array[numeric])=[0.18461538461538463, 0.07466342093496944]
  out "Monitor Current (mA)":dbl=4.104672235741318 min=0.0 max=1.9 format="%_4e"
  out "Graph 7":T9(graph)=[{"TimeArray (USB6218)"=[timestamp(3682722306.0778 s since 1904-01-01), timestamp(3682722307.1276407 s since 1904-01-01), timestamp(3682722309.0611777 s since 1904-01-01), timestamp(3682722309.8881736 s since 1904-01-01), timestamp(3682722311.8328657 s since 1904-01-01)], "DataArrayConv (USB6218)"=[]}, {"TimeArray (USB6218)"=[], "DataArrayConv (USB6218)"=[]}] caption="XY Graph"
  in  "upper limit (V)\n (Kikusui)":dbl=20.0 format="%_3f"
  in  "lower limit (V) \n(Kikusui)":dbl format="%_3f"
  in  "lower limit (mA) \n(Kikusui)":dbl=4.0 format="%_3f"
  in  "upper limit (mA)\n (Kikusui)":dbl=20.0 format="%_3f"
  in  "lower limit (mA)":dbl=4.0 format="%_3f"
  in  "SetCurrent 2 (mA)":dbl=8.0 format="%_3f"
  in  "upper limit (mA)":dbl=20.0 format="%_3f"
  out "error out (KIKUSI CTRL)":errorcluster
  out "ActualVoltage (V)":dbl[](array[numeric]) format="%_6g"
  out "ActualCurrent (A)":dbl[](array[numeric])=[0.004, 0.008] format="%_3e"
  in  "SetCurrent 1 (mA)":dbl=3.9999999999999996 format="%_3g"
  in  "Output\n (ADCMT)":bool[](array[boolean])=[FALSE, FALSE]
  out "error out (ADCMT6420A)":errorcluster
  in  "Voltage limits (V)":dbl[](array[numeric])=[12.0, 12.0] format="%_3f"
  in  "CtrlLabels":string[](array[string])=["CV2", "CV3"]
  in  "VISA":refnum<visa-resource-name>[](array[refnum])=["GPIB0::1::INSTR", "GPIB0::12::INSTR"]
  out "Initialized?":bool=TRUE
  in  "InstName":string="ADCMT"
  out "Graph 6":T8(graph)=[{"TimeArray"=[timestamp(3682722298.1082263 s since 1904-01-01), timestamp(3682722301.293357 s since 1904-01-01), timestamp(3682722302.439338 s since 1904-01-01)], "Filtered X"=[0.004, 0.004, 0.004]}, {"TimeArray"=[timestamp(3682722298.1082263 s since 1904-01-01), timestamp(3682722301.293357 s since 1904-01-01), timestamp(3682722302.439338 s since 1904-01-01)], "Filtered X"=[0.008, 0.008, 0.008]}, {"TimeArray"=[timestamp(3682722298.1082263 s since 1904-01-01), timestamp(3682722301.293357 s since 1904-01-01), timestamp(3682722302.439338 s since 1904-01-01)], "Filtered X"=[0.003999999999999999, 0.003999999999999999, 0.003999999999999999]}, {"TimeArray"=[timestamp(3682722298.1082263 s since 1904-01-01), timestamp(3682722301.293357 s since 1904-01-01), timestamp(3682722302.439338 s since 1904-01-01)], "Filtered X"=[0.008, 0.008, 0.008]}] caption="XY Graph"
  in  "Initialize":bool
  in  "CONTROL KIKUSUI?":bool=TRUE
  in  "OUTPUT\n(Kikusui)":bool
  in  "Set Voltage (V)\n (Kikusui)":dbl=12.0 min=0.0 max=49.0 format="%_3g"
  in  "Set Current (mA)\n (Kikusui)":dbl=5.0 min=0.0 max=1.9 format="%_3g"
  out "DP HEX5":dbl=101960.43422179746 format="%_4e"
  out "DP_HEX5":dbl=101960.43422179746 format="%_4e"
  in  "Diff pressure HEX5":string="DP_HEX5"
  out "3He pot level":dbl=31.04734165451921 format="%_4f"
  in  "3He pot":string="L1"
  out "He level (3He)":dbl(slide)=31.04734165451921 scale=0.0..100.0
  out "He level (1K) b":dbl(slide)=31.04734165451921 scale=0.0..100.0
  out "He level (1K)":dbl(slide)=31.04734165451921 scale=0.0..100.0
  out "He level (4K)":dbl(slide)=31.04734165451921 scale=0.0..100.0
  out "1K pot(b1)":dbl=31.04734165451921 format="%_4f"
  in  "1K pot (b)":string="L2-2"
  in  "1K pot level":string="L2-1"
  out "L(1K) (a1)":dbl=31.04734165451921 format="%_4f"
  in  "SensorLocation 2":T10(ring)=enum."TTH4"
  out "Temperature 2":dbl=252.6
  out "DP HEX4":dbl=101960.43422179746 format="%_4e"
  in  "Diff pressure HEX4":string="DP_HEX4"
  out "V2":bool
  out "V1":bool
  out "F5 (3He pump ex.)":dbl=31.04734165451921 format="%_4e"
  out "F4 (3He in flow to HEX7)":dbl=-8.463214304279017 format="%_4e"
  out "F3 (4He rtn flw via HEX7)":dbl=0.19062223546802864 format="%_4e"
  out "F1 (1K pump exhaust) flow":dbl=11.563316028234391 format="%_4e"
  out "P (Dewar)":dbl=101960.43422179746 format="%_4e"
  out "P (1K pot)":dbl=101161.60088168262 format="%_4e"
  out "P (3He pot)":dbl=100974.8496520803 format="%_4e"
  out "P (shield return)":dbl=101003.37781721646 format="%_4e"
  out "P (3He IN)":dbl=100916.22322905027 format="%_4e"
  out "P (4K reservoir)":dbl=101450.66177958067 format="%_4e"
  out "P (insulation)":dbl=0.00032199835577441523 format="%_4e"
  in  "3He pump exhaust flow":string="F_5"
  out "F_5":dbl=31.04734165451921 format="%_4f"
  in  "3He incoming flow into HEX7":string="F_4"
  out "F_4":dbl=-8.463214304279017 format="%_4f"
  out "F_3":dbl=0.19062223546802864 format="%_4f"
  in  "4He return flow from HEX7":string="F_3"
  out "F_2":dbl=0.386580406013938 format="%_4f"
  in  "Shield flow":string="F_2"
  out "P_SldRTN":dbl=101003.37781721646 format="%_4e"
  in  "3He pot pressure":string="P_3Hepot"
  out "P_3Hepot":dbl=100974.8496520803 format="%_4e"
  in  "Shield return press.":string="P_SldRTN"
  out "F_1":dbl=11.563316028234391 format="%_4f"
  in  "1K pump exhaust flow":string="F_1"
  out "P_Dewar":dbl=101960.43422179746 format="%_4e"
  in  "Dewar pressure":string="P_Dewar"
  out "P_1Kpot":dbl=101161.60088168262 format="%_4e"
  in  "1Kpot pressure":string="P_1Kpot"
  out "P_3HeIN":dbl=100916.22322905027 format="%_4e"
  in  "3He inlet pressure":string="P_3HeIN"
  in  "4K reservoir pressure":string="P_4Kres"
  out "P_4Kres":dbl=101450.66177958067 format="%_4e"
  out "P_ins":dbl=0.00032199835577441523 format="%_4e"
  in  "Insulation vacuum":string="P_ins"
  out "T3He7-1/6-2 (3He pot) 2":dbl=137.447 format="%_4f"
  out "T3He7-1/7-2 (HEX1)":dbl=138.238 format="%_4f"
  out "T3He6-1/6-2 (3He pot) 2":dbl=138.305 format="%_4f"
  out "T3He6-1/6-2 (HEX1)":dbl=138.289 format="%_4f"
  out "T1K3-1/3-2 (1K pot) 2":dbl=95.288 format="%_4f"
  out "T1K3-1/3-2 (1K pot)":dbl=105.4208 format="%_4f"
  out "T4He1 (4K reservoir )":dbl=71.656 format="%_4f"
  out "Temperature 1":dbl=252.6
  in  "SensorLocation 1":T10(ring)=enum."TTH4"
  out "TIP7":dbl format="%_4g"
  out "T3He6-2":dbl=138.305 format="%_4g"
  out "T3He7-2":dbl=137.447 format="%_4g"
  out "T3He6-1":dbl=138.289 format="%_4g"
  out "T3He4":dbl=143.19 format="%_4g"
  out "T3He7-1":dbl=138.238 format="%_4g"
  out "T3He8":dbl=132.559 format="%_4g"
  out "T3He5":dbl=133.191 format="%_4g"
  out "T1K3-2":dbl=95.288 format="%_4g"
  out "T1K3-1":dbl=95.4208 format="%_4g"
  out "TIP6":dbl=149.97 format="%_4g"
  out "T3He9":dbl=128.03 format="%_4g"
  out "T1K5":dbl=102.91 format="%_4g"
  out "T1K4":dbl=93.845 format="%_4g"
  out "T1K2":dbl=126.48 format="%_4g"
  out "TIP5":dbl=153.46 format="%_4g"
  out "TIP4":dbl=114.84 format="%_4g"
  out "TIP3":dbl=199.72 format="%_4g"
  out "TIP2":dbl=231.46 format="%_4g"
  out "TIP1":dbl=279.27 format="%_4g"
  out "T1K6":dbl=284.49 format="%_4g"
  out "T4He10":dbl=270.39 format="%_4g"
  out "T4He8":dbl=274.6 format="%_4g"
  out "T4He7":dbl=249.16 format="%_4g"
  out "T3He1-3":dbl=290.57 format="%_4g"
  out "T3He1-2":dbl=290.84 format="%_4g"
  out "T4He9":dbl=235.88 format="%_4g"
  out "T4He6":dbl=194.05 format="%_4g"
  out "T4He5":dbl=188.35 format="%_4g"
  out "T4He4":dbl=195.1 format="%_4g"
  out "T4He2-2":dbl=204.02 format="%_4g"
  out "T4He2-1":dbl=207.68 format="%_4g"
  out "T4He3-4":dbl=292.38 format="%_4g"
  out "T4He3-3":dbl=292.31 format="%_4g"
  out "T4He3-2":dbl=292.75 format="%_4g"
  out "T4He3-1":dbl=292.61 format="%_4g"
  out "T3He1-4":dbl format="%_4g"
  out "T3He3":dbl=131.72 format="%_4g"
  out "T3He2-2":dbl=199.47 format="%_4g"
  out "T3He2-1":dbl=207.67 format="%_4g"
  out "T1K1":dbl=129.11 format="%_4g"
  out "T4He1":dbl=71.656 format="%_4g"
  out "TTH1":dbl=172.52 format="%_4g"
  out "TTH2":dbl=177.97 format="%_4g"
  out "TTH4":dbl=252.6 format="%_4g"
  out "TTH3":dbl=245.42 format="%_4g"
  out "T3He1-1":dbl=290.7 format="%_4g"
  out "T3He10":dbl=285.44 format="%_4g"
  out "F2 (shield flow)":dbl=0.386580406013938 format="%_4e"
  out "DP_HEX4":dbl=101960.43422179746 format="%_4e"
  in  "4K reservoir level":string="L3"
  out "L3":dbl=31.04734165451921 format="%_4f"
  out "Series 1":string[](array[string])=["P_Dewar"]
  out "Series 2":string[](array[string])=["T4He6", "T4He9", "T3He1-2", "T3He1-3", "T4He7", "T4He8", "T4He10", "T1K6", "TIP1", "N.C.", "TIP2", "T1K3-1", "T1K3-2", "T3He5", "T3He8", "T3He6-1", "T3He6-2", "T3He7-1", "T3He7-2"]
  out "Series 3":string[](array[string])=["P_ins", "P_4Kres", "P_3HeIN", "P_SldRTN", "P_3Hepot", "P_1Kpot", "DP_HEX4", "DP_HEX5", "F_1", "F_2", "F_3", "F_4", "F_5", "I_CV"]
  out "Series 4":string[](array[string])=["L1", "L2-1", "L2-2", "L3"]
  out "Plot errors":errorcluster
  out "LastMeasurementConfig (218)":T11(array[cluster])=[{"LSIName"="LSI218A", "Active?"=TRUE, "LastData"=[285.45, 290.71, 245.43, 252.59, 172.54, 177.97, 71.656, 129.11], "Labels"=["T3He10", "T3He1-1", "TTH3", "TTH4", "TTH1", "TTH2", "T4He1", "T1K1"]}, {"LSIName"="LSI218B", "Active?"=TRUE, "LastData"=[30.0, 0.0, 0.0, 0.0, 207.67, 199.47, 131.72, 290.16], "Labels"=["N.C.", "N.C.", "N.C.", "N.C.", "T3He2-1", "T3He2-2", "T3He3", "T3He1-4"]}, {"LSIName"="LSI218C", "Active?"=TRUE, "LastData"=[292.6, 292.74, 292.31, 292.37, 207.68, 204.03, 195.11, 188.36], "Labels"=["T4He3-1", "T4He3-2", "T4He3-3", "T4He3-4", "T4He2-1", "T4He2-2", "T4He4", "T4He5"]}, {"LSIName"="LSI218D", "Active?"=TRUE, "LastData"=[194.01, 235.91, 290.83, 290.58, 249.16, 274.59, 270.4, 284.47], "Labels"=["T4He6", "T4He9", "T3He1-2", "T3He1-3", "T4He7", "T4He8", "T4He10", "T1K6"]}, {"LSIName"="LSI218E", "Active?"=TRUE, "LastData"=[279.27, 0.0, 231.46, 688.49, 199.72, 114.83, 153.45, 688.58], "Labels"=["TIP1", "N.C.", "TIP2", "N.C.", "TIP3", "TIP4", "TIP5", "N.C."]}, {"LSIName"="LSI218F", "Active?"=TRUE, "LastData"=[126.48, 94.139, 102.89, 143.16, 127.49, 149.95, 0.433, 0.0], "Labels"=["T1K2", "T1K4", "T1K5", "T3He4", "T3He9", "TIP6", "N.C.", "N.C."]}]
  out "DataArrayConv (USB6210)":dbl[][](array[numeric])
  out "LastMeasurementConfig (336)":T11(array[cluster])=[{"LSIName"="LSi336X", "Active?"=TRUE, "LastData"=[95.4242, 95.2873, 133.19, 132.559], "Labels"=["T1K3-1", "T1K3-2", "T3He5", "T3He8"]}, {"LSIName"="LSi336Y", "Active?"=TRUE, "LastData"=[138.289, 138.31, 138.239, 137.444], "Labels"=["T3He6-1", "T3He6-2", "T3He7-1", "T3He7-2"]}]
  out "DataArrayConv (USB6218)":dbl[][](array[numeric])=[[11.490982481403101, 0.18273130197144594, 0.10513712758129379, -8.492805305061522, 30.587037338056568, -0.4467107834284478, -25.01730848687032], [11.58961913293365, 0.27873765455439214, 0.18930708004284258, -8.696654424264324, 30.882947256300454, -0.407247924666102, -24.99100537660044], [11.316724392303513, 0.1906222354247991, 0.21429503482473616, -9.071473772921438, 30.215505993440544, -0.13100791365129427, -24.98525157123842], [11.609346466643878, 0.08540979493210105, 0.19851316875147262, -8.558563085403442, 30.679098201121125, -0.06523648251544611, -25.035391875201192], [11.408785267398217, 0.19982832355139224, 0.29188920945905766, -9.199701445997562, 30.564022120811956, -0.7755679404119076, -25.001691015150374], [11.280557618819653, 0.4063077381192367, 0.3707985400753195, -9.318065451198459, 31.244614934109162, -0.6045622190648992, -25.004978903948793], [11.23781506863284, 0.1695797473442457, 0.25901032169088317, -8.755836426452737, 30.682386088525128, -1.1965051004229061, -25.013198625892088], [11.247678732990337, 0.09198557252944767, 0.1485372591722502, -8.719669647222561, 30.96514445628075, -0.6308707912467537, -25.003334959551943], [11.333163834776823, 0.26690125458449987, 0.07094308404610972, -8.657199755715721, 30.702113416623977, -1.1044250962649338, -24.985251571250938], [11.382482160824328, 0.18667676879071732, 0.2866285875458375, -9.387111119605493, 31.12296307874075, -0.8413393717973289, -25.003334959534047], [10.97149610069009, 0.06962792888078789, 0.2853134319841271, -9.193125666645193, 30.899386696069662, -1.2359679593997026, -25.02141834785811], [10.961632435400107, 0.12880992663947866, 0.2629557884889442, -9.212853002836892, 30.87637148017886, -0.9202650887594704, -24.99758115417236], [11.55345236284882, 0.10908259383470037, 0.08146432832322997, -8.959685546591448, 30.534431128691796, -0.7361050817496301, -25.010732709307952], [11.537012920386381, -0.0645179334322391, 0.22218596796138873, -9.462732567656094, 30.517991690252522, -0.5387907871187936, -25.007444820515133], [11.602770689682304, 0.04595512944075686, 0.08277948377222166, -8.581578308823968, 30.51470380140865, -1.130733669086672, -25.001691015148946], [11.586331247657418, 0.23928298927602942, 0.1222341492013323, -8.864336765720951, 30.975008120060217, -0.5256365008951391, -24.969634099523855], [11.934847423054636, 0.12354930458952762, 0.11697352656795973, -8.752548537237095, 30.583749449675857, -0.39409363853383617, -25.00497890394045], [11.809907663165475, 0.25901032194455026, 0.09987650548610605, -8.469790083152125, 31.040765879768717, -0.6834879361905949, -25.020596375679833], [11.264118176490383, 0.1787858356220916, 0.3352893413056002, -8.667063423594708, 30.633067768810697, -0.7624136540439441, -24.997581154167637], [11.609346466832863, 0.3589621401554776, 0.10908259418139332, -8.607881420665949, 30.882947253788313, -0.7229507948351943, -25.01155468149601], [11.5666039166006, 0.24322845555311945, 0.16694943655568423, -8.93338243454018, 30.797462168942356, -0.5124822147330038, -25.03046004202788], [11.513997701322246, 0.26032547720985183, 0.16431912561062356, -8.660487646525745, 31.172281398033995, -0.7624136543357224, -25.00169101515301], [11.418648934646505, -0.00796624659380718, 0.216925345832929, -9.156958888385258, 30.984871783453492, -0.6177165053589412, -25.01155468153301], [11.333163834137396, 0.3602772955422935, 0.27084672151487876, -8.854473097591264, 31.057205319599067, -0.3677850662851212, -25.01813045907319], [11.13589052562087, 0.1367008587328583, 0.1630039700939403, -9.383823231284946, 30.478537034131183, -0.7097965085394703, -25.021418347879194], [12.03677196699588, 0.032803574387140044, 0.06305215128172026, -8.926806656386994, 30.146460345753333, 4.196752238706526, -25.009088764923405], [11.69483156541343, 0.19456770208500096, 0.16431912551690975, -8.450062748726507, 31.03419010347982, 2.6840093310248223, -24.98689551562517], [11.296997061240452, 0.2353375229199257, 0.16431912554549244, -8.423759637899142, 30.9322655756951, 4.525609391337346, -25.015664542499167], [11.48111881652701, 0.28662858757665344, 0.20640410162105444, -8.344850299937132, 30.741568072714685, 4.512455105664342, -25.005800876121693], [11.504134035227695, 0.0893552613053823, 0.14064632586784898, -8.841321541329352, 30.616628329076327, 4.538763677132864, -25.01648651469523], [11.90854431702662, 0.2156101903358444, 0.06042184026468472, -8.785427427882212, 30.932265576275363, 3.762660794945796, -24.998403126369627], [11.513997700808494, 0.2747921873826553, 0.24980423360728216, -8.801866873211754, 31.346539460825763, 3.7626607957664246, -25.005800876130035], [11.49098248131275, 0.11960383788932238, 0.0656824622824208, -8.985988658712222, 30.60676466604444, 4.170443663281372, -25.011554681522803], [11.504134034914774, 0.1656342809324548, 0.2471739224851784, -9.350944340711155, 30.764583289103513, 4.328295099160375, -25.004978903931885], [11.487694593362393, 0.05779152909716451, 0.09067041705806561, -8.302107742862296, 30.72841652060969, 5.143860837763778, -25.002512987353576], [11.35946694179938, 0.2945195208556215, 0.14459179285486234, -8.640760311640621, 31.09665997523212, 3.4601122146074337, -24.993471293188524], [11.34960327725615, 0.21955565672792082, 0.1340705486112111, -8.499381085032953, 30.71855285683536, 4.972855118852794, -24.999225098560753], [11.323300169337553, 0.2958346757859944, 0.14853725927559763, -8.246213630939824, 30.95856867929743, 4.630843680254304, -24.99511523759339], [11.343027499831209, 0.1971980129461075, 0.17878583586159214, -9.058322217018965, 30.537719017370396, 4.999163689607002, -25.003334959550294], [11.214799849333652, 0.1682645918427173, 0.152482725576003, -8.69994231322289, 30.94541712790173, 5.170169410335134, -25.006622848326977], [11.694831566049324, 0.10645228310730631, 0.12354930468467995, -8.719669647039604, 30.66594664943561, 4.104672235741318, -24.985251571232826], [11.3561790540713, 0.16563428110695966, 0.2419133003458253, -8.903791432344011, 30.942129240024325, 4.236215096831768, -25.0099107371075], [11.58304335780301, 0.16826459199620225, 0.15511303705807572, -8.565138864832363, 31.303796915982918, 4.749232255496515, -25.01977440348003], [11.296997061349288, 0.15642819188859003, 0.16957974729617487, -8.801866873047695, 30.761295400579048, 2.7103179040088308, -25.00251298735928], [11.773740890305548, 0.3273984081929371, 0.12617961577417397, -8.318547188457153, 30.458809704916966, 4.24936937918712, -24.98360762685409], [11.530437142999236, 0.2892588982203344, 0.10776743835148439, -8.57829042068449, 30.692249753576657, 4.5387636774521924, -24.991827348815608], [11.441664154315093, 0.26821641020579745, 0.09593103884935505, -8.765700093686734, 31.10652363904777, 3.986283659825639, -25.014842570286522], [11.487694593426465, 0.14327663740091723, 0.08804010598887785, -8.371153412325885, 31.21502394179917, 4.933392259687649, -25.006622848329613], [11.724422560908906, 0.0038701533121064946, 0.04200966292254976, -8.752548538105561, 30.859932040831428, 4.1441350940945725, -25.03539187519175], [11.573179691901384, 0.0946158834193292, 0.19456770211979546, -8.650623978046331, 30.672522425053728, 4.157289378771079, -25.003334959536023], [11.622498020431989, 0.19062223547388768, 0.04332481866714627, -8.311971409622771, 30.935553464413125, 4.341449385738266, -25.003334959539973], [10.932041439003562, 0.12486446009947078, 0.4155138268466323, -8.87091254222994, 31.15255407018573, 3.591655075687629, -25.002512987345337], [11.648801127948376, 0.08672495015110332, 0.24454361102304417, -8.785427428737883, 30.494976474285686, 4.880775115228005, -25.014020598109894], [11.431800489175444, 0.26164063268574317, 0.18667676922523302, -8.551987308619152, 31.063781094431626, 4.9333922588917405, -25.01402059808496], [11.326588057630529, 0.047270285111469856, 0.17878583604706966, -8.423759635839918, 30.61005255347151, 4.249369381738312, -24.99922509857393], [11.938135311970399, 0.1616888143913328, 0.18010099137564967, -9.04845854932204, 30.639643545287353, 5.841038000070986, -25.007444820531166], [11.38905793856813, 0.1314402374978048, 0.19982832427219893, -8.627608755579605, 31.178857173247394, 3.9731293736403375, -24.998403126374352], [11.20493618394129, 0.26427094361574394, 0.2511193890151714, -9.143807331909667, 30.646219320909584, 3.973129374191226, -24.98525157124556], [11.520573477936999, 0.18536161338669932, 0.20508894615885265, -8.64404820072753, 30.758007512151963, 4.61768939294551, -24.996759181972124], [11.648801127237865, 0.1472221037437681, 0.2248162785409878, -9.097776885987265, 30.18920288925773, 4.4861465329015955, -24.9975811541661], [11.477830927105408, 0.3602772955697025, 0.22350112325037008, -8.384304968631232, 30.922401912365444, 3.4074950695641135, -24.97620987708589], [11.208224072183421, 0.261640632531558, 0.2576951664750871, -8.515820529183463, 30.955280791380712, 4.236215096656388, -25.000047070763298], [11.533725032031802, 0.28136796496159283, 0.1761555246875135, -9.018867549130013, 30.36674884264524, 4.420375100249781, -24.99840312636381], [11.257542399654593, 0.05516121792874357, 0.21824050120227734, -9.1964135561706, 30.771159063265586, 3.696889363571666, -25.021418347873155], [11.533725030831059, 0.16300396946990808, 0.22613143396148733, -9.173398333517598, 30.636355656384307, 3.4995750736956746, -25.006622848328625], [11.267406064948487, 0.31161654221495283, 0.2826831206829793, -8.436911193441471, 31.155841958435044, 4.130980808297173, -25.003334959567535], [11.412073157694342, 0.1577433477874154, 0.31293169703587137, -8.96626132472456, 30.4423702663223, 4.893929400351923, -25.000869042964517], [11.714558897258637, 0.18404645785937973, 0.03280357439560483, -9.288474449552917, 30.734992296048024, 4.0783636614594565, -25.01977440347015], [11.507421922732313, 0.21429503477160372, 0.2747921881032965, -9.541641904813343, 30.708689193235184, 4.157289380258517, -25.0000470707667], [11.31343650320379, 0.19193739117487718, 0.16168881447827366, -8.900503543472823, 30.804037944567597, 4.3940665297226085, -25.008266792714164], [11.421936822726948, 0.33528934081932094, 0.24454361140224945, -8.358001855686265, 30.932265576176448, 4.223060810047171, -24.999225098564487], [11.320012280603757, 0.39184102786781666, 0.2116647234762839, -8.913655099736326, 30.859932039866845, 4.617689393436315, -24.98525157123469], [11.359466942558269, 0.25374969951771364, 0.1380160153659168, -9.21614088997085, 30.68567397690054, 4.854466544401205, -24.996759181975087], [11.21151196070096, 0.21561018934420995, 0.18141614713988824, -8.621032977073492, 30.905962470907255, 4.380912243319898, -25.015664542484338], [11.537012920627934, 0.16037365847752522, 0.034118729761182964, -8.706518091199149, 30.843492600182632, 3.0523293422666047, -25.01073270929906], [11.704695232582127, 0.10908259419615718, 0.11171290507204756, -8.785427428475927, 30.72184074532085, 5.525335134902942, -25.001691015155203], [11.19178462998844, 0.14327663738580193, 0.09198557242903155, -8.995852325116555, 30.22865754683446, 3.920512224895726, -24.9794977658696], [11.467967261099128, 0.2287617446073898, 0.23139205644867122, -9.160246776752258, 30.879659367720368, 4.788695110710433, -25.0205963756929], [11.691543677021098, 0.43918662611029236, 0.2695315658782726, -8.173880071621355, 30.991447559469176, 4.854466544169839, -24.99264932099081], [11.267406064810318, 0.17484036946047787, 0.2537496997529462, -9.110928441528635, 30.945417127549295, 4.6439979663463316, -25.02059637565754], [11.481118816209705, 0.210349568000888, 0.18404645810879078, -9.219428780228679, 30.685673976856208, 4.578226535423113, -24.987717487822113], [11.329875946028352, 0.20245863520867452, 0.19062223561479003, -8.670351312861763, 30.938841352066316, 4.617689393709717, -25.030460042013164], [11.612634352381287, 0.18536161376067634, 0.27742249918069106, -8.542123640867594, 31.159129846474254, 4.565072248715825, -24.996759181970585], [11.606058578615938, 0.2511193886070723, 0.04200966305491066, -8.657199756040058, 30.853356264142658, 4.8018493991914655, -25.001691015159818], [11.737574115897516, 0.18141614707145182, 0.12617961560138247, -8.959685546847975, 30.69882552886415, 4.591380822260423, -24.980319738068847], [11.204936182972705, 0.18536161370412985, 0.34844089606606093, -8.910367211273423, 30.81718949706903, 4.617689393016876, -25.00744482054127], [11.366042719140374, 0.16431912547021216, 0.16957974757011207, -8.538835752335572, 30.498264361254968, 4.986009404436309, -25.01730848688844], [11.64551323982406, 0.27742249918470896, 0.13012508200383055, -8.42047174696457, 30.830341047905996, 3.7758150829860964, -25.01484257029728], [11.336451723145458, 0.4089380495894067, 0.14722210390966028, -8.683502869478591, 31.504358083933575, 3.6574265063055824, -25.01484257028026], [11.444952042141013, 0.14853725901717046, 0.06436730675290708, -9.028731215944132, 30.554158458011333, 3.9994379461594907, -25.00169101515246], [11.46139148492832, 0.19851316869843755, 0.24848907784158097, -8.532259973825003, 30.76787117669485, 4.6439979664410105, -25.02552820885875], [11.790180330339062, 0.21429503498046137, 0.14722210366835664, -8.584866199706713, 30.48840069843553, 4.1835979519428985, -24.988539460034865], [11.560028138327013, 0.1577433477233664, 0.24322845597049714, -9.268747115032323, 30.347021514508864, 4.367757957005107, -25.011554681504023], [10.974783989244564, 0.06436730654608763, 0.2695315659489414, -8.94982187909774, 30.22208177031035, 4.512455105264605, -24.998403126360408], [11.73757411768901, 0.3050407646433977, 0.03937935190537306, -8.768987982367756, 30.593613113286988, 3.9468208018141113, -24.996759181983215], [11.270693953340778, 0.05647637334519895, 0.010445930678276594, -8.76898798249356, 30.26811220269948, 4.380912243130697, -24.987717487823872], [11.053693313389731, 0.22481627847191282, 0.20114347981800534, -9.153670999310688, 30.80732583272507, 4.078363663290623, -25.016486514677112], [11.53372503198196, 0.21955565685679657, 0.1735252140766103, -8.864336765272949, 31.195296614132584, 4.025746518319017, -25.001691015151362], [11.201648294885306, 0.2879437429877677, 0.3050407647955287, -8.890639876225093, 31.333387908859596, 4.012592230578262, -24.999225098558007], [11.619210131681665, 0.34318027448452737, 0.22087081239644213, -9.035306993708554, 30.879659368151234, 4.736077969236117, -25.005800876133765], [11.586331247860352, 0.1090825938527224, 0.0735733954352426, -8.3875928573483, 30.534431129287505, 4.315140812231588, -25.012376653693607], [11.188496741206428, 0.23533752260488622, 0.3010952983541011, -8.752548538462053, 30.527855351165485, 4.144135093826316, -24.984429599042798], [11.52714925388285, 0.2353375226812675, 0.17878583609299487, -8.673639201081055, 30.96514445553463, 5.104397980353438, -24.991827348797386], [11.625785908751691, 0.14196148175098983, 0.12354930481913112, -8.959685546361996, 30.72184074500256, 4.643997965420521, -24.999225098575575], [11.234527179893057, 0.18141614703087855, 0.29320436517244913, -9.03530699398904, 31.33338790896548, 4.5782265358684855, -25.01073270930697], [11.573179693878725, 0.3287135633418243, 0.07751886192346741, -8.34156241153696, 30.853356263671657, 4.709769396138661, -24.99347129320532], [11.264118176507147, 0.34975605136471516, 0.29451952040311036, -8.548699418381519, 31.093372087018185, 4.696615108116297, -24.98936143222182], [11.418648935228177, 0.1498524149548467, 0.1011916609965064, -8.798578984806364, 30.353597289914607, 4.591380821730982, -24.989361432227085], [11.50413403487677, 0.3694833844462332, 0.21561019037551232, -9.268747115294081, 30.859932040582017, 3.5390379317261202, -24.98689551564197], [11.941423201444337, 0.37605916166655085, 0.024912641323538043, -8.384304967633211, 31.310372693185073, 5.1964779806748105, -24.994293265396998], [11.793468220551777, 0.08672495037927663, 0.14985241490832213, -8.857760986878587, 31.182145061828216, 2.789243620833091, -25.00086904294937], [11.32658805762146, 0.339234807828827, 0.198513168798701, -8.72953331527837, 31.021038551346543, 4.538763676302083, -25.00004707077219], [11.55345236219298, 0.15248272591201378, 0.19982832417004498, -8.765700093960195, 31.18872083740595, 4.301986525066979, -24.999225098561194], [11.099723752019482, 0.251119388589293, 0.19456770209876206, -9.028731215325159, 31.168993510384325, 4.038900804986406, -24.995937209781], [11.195072517832564, 0.21297987896775988, 0.2721618768902532, -9.433141566023213, 30.74485596099238, 4.367757957182527, -25.00744482051601], [11.494270370362027, 0.1722100582414982, 0.06962792885251401, -8.37115341297862, 30.406203498603222, 4.262523669177238, -24.992649320990374], [11.316724392009734, 0.16826459220368856, 0.31556200868490736, -9.242444002633254, 30.64293143263136, 5.025472263503187, -24.99429326538525], [11.711271009574919, 0.16300396981940024, 0.1248644603595267, -8.982700769401871, 30.652795096243064, 4.670306538025655, -25.04361159717556], [11.227951403078752, 0.19062223544310897, 0.23533752228807298, -9.12079210791374, 30.83362893691921, 5.656877995171407, -24.99758115417137], [11.40878526944105, 0.2353375226042836, 0.1774706804339341, -8.828169984989637, 30.393051946294225, 5.170169409910922, -24.979497765872342], [11.027390205156111, 0.21824050093024783, 0.4010471164191006, -8.699942314505, 30.698825528923262, 4.2888322402336705, -25.00744482052743], [11.441664152823417, 0.24848907791035652, 0.1866767688538099, -9.255595558674509, 30.774446952718442, 4.157289380325122, -25.015664542483023], [11.661952680947634, 0.09593103886931964, 0.2563800108120371, -9.272035003878063, 30.613340441057584, 4.130980808170916, -25.01237665369031], [11.336451723229338, 0.15248272559331305, 0.13144023776404523, -8.821594208617848, 30.557446344399008, 4.657152252987179, -25.001691015165306], [11.62907379688268, 0.26953156583444027, 0.32476809700664916, -8.851185210584596, 31.116387302294235, 4.236215096362043, -25.002512987382126], [11.87895331953046, 0.22744659002391626, 0.11565837140181628, -8.745972759195269, 31.698343473214997, 4.130980807965709, -25.008266792714384], [11.435088376928238, 0.106452282990956, 0.26032547742344697, -9.410126343375689, 30.72841652128833, 4.341449384772161, -25.001691015148946], [11.477830927829439, 0.16826459173286418, 0.2064041017418511, -8.939958212110415, 30.425930825415627, 5.025472261725607, -24.991827348816816], [11.809907662635128, 0.14590694818551703, 0.19193739117807473, -8.676927091111668, 30.61662832964272, 4.670306538963496, -25.003334959543377], [11.356179049661339, 0.15248272603470436, 0.2300769007288892, -8.82159420673442, 30.89609880849463, 3.302260781062552, -24.991005376598466], [11.701407343709565, 0.251119389014293, 0.29451952033844364, -8.775563761002719, 30.830341047899072, 5.104397979084068, -24.990183404412612], [11.451527820038521, 0.23533752260694135, 0.20377379076994845, -9.189837778759827, 30.925689799968016, 4.683460824874937, -25.004156931732858], [11.241102957022148, 0.16168881438995564, 0.2708467211518367, -9.064897994901308, 31.201872390004525, 4.433529388607073, -25.000869042961227], [11.698119454813524, 0.29714983154011965, 0.18667676893211282, -8.683502868214557, 31.047341655538336, 5.025472263240087, -24.981141710261067], [11.162193633292464, 0.2747921877807923, 0.26032547766719816, -8.864336764226472, 31.13940251912539, 4.052055090080714, -25.00991073710684], [11.490982480002403, 0.11171290492169167, 0.29714983183511756, -8.946533991218192, 30.82705315946469, 4.51245510504014, -24.996759181975197], [11.569891805215597, 0.2169253453875148, 0.21955565686187556, -8.867624653942892, 30.57717367344933, 5.025472257451534, -24.970456071721237], [11.471255150231356, -0.032954201256366056, 0.12354930465106401, -9.16353466563911, 30.85664415241178, 4.328295098396316, -24.993471293192147], [11.609346464833607, 0.25901032189018086, 0.20508894639509267, -8.722957537447684, 31.096659974790313, 4.459837959880813, -24.99347129319522], [11.283845507506088, 0.22218596741447816, 0.2563800110169885, -8.880776209986244, 30.93226557455938, 4.367757957511996, -24.981141710265785], [11.412073157867491, 0.11960383770528504, 0.11039774968052246, -8.91365509965694, 30.817189496424604, 3.407495069203982, -24.985251571240948], [11.648801127130156, 0.06436730676996433, 0.05779152929697928, -8.788715316509283, 30.550870569718292, 4.052055089759689, -24.970456071718054], [11.717846782420512, 0.18667676920031784, 0.21955565660824305, -9.344368562611708, 30.78759850516774, 5.209632268353697, -24.98196368245845], [11.754013556802008, 0.2945195207187883, 0.1182886822819364, -9.202989336279188, 30.54429479281543, 5.064935121782783, -24.994293265395456], [11.911832203624947, 0.03806419641263403, 0.09856134953862539, -9.097776884753769, 30.478537034186786, 4.472992247123424, -24.979497765865865], [11.619210129515494, 0.3247680973885546, 0.18536161327777972, -8.722957537800994, 31.168993509928654, 3.23648935076917, -24.976209877089182], [11.487694593389461, 0.09593103887110654, 0.06173699561125606, -8.226486296317288, 30.5475826819883, 5.4990265612601785, -25.000047070768343], [11.592907024456297, 0.16037365878388965, 0.15642819235834687, -8.69665442535664, 30.570597897261255, 4.078363663276581, -25.00826679272284], [11.911832205869729, 0.207719257208889, 0.11039774975550326, -8.838033652584844, 30.971720231811943, 4.10467223335575, -25.00086904297012], [11.490982481375504, 0.24322845581166475, 0.2734770324507107, -8.857760987249916, 30.531143240993035, 4.288832239921005, -24.99511523760744], [11.448239931168354, 0.12749477122753877, 0.152482725932384, -8.844609431013899, 30.748143848643412, 5.051780835887108, -24.98525157124457], [12.056499297068243, 0.13933117074205575, 0.05516121808433716, -8.736109092448645, 30.836916824531464, 4.56507224961168, -24.991827348796505], [11.329875946227974, 0.16431912502809815, 0.2077192570705204, -9.183262001770663, 30.52456746615831, 3.854740799089355, -25.01648651468787], [11.707983120998456, 0.08672495039824119, 0.12223414894544504, -8.565138864569343, 30.89938669636406, 4.788695112571493, -25.00908876491945], [11.546876585794195, 0.08804010581144506, 0.17221005825038566, -8.545411530051346, 30.938841351570552, 4.762386541353565, -25.009910737134845], [11.717846785955107, 0.18273130237443408, 0.15116757020515198, -8.558563085295013, 30.478537033690966, 5.249095127141636, -24.981141710255358], [11.777028777074735, -0.004020779757986315, 0.04069450737719349, -8.861048875393408, 30.268112202534443, 4.762386538574431, -24.969634099525393], [11.737574115131284, 0.13144023779687236, 0.09856134989936727, -8.54541152939295, 30.75143173644618, 4.301986527346431, -24.993471293186985], [11.198360406201266, 0.1143432158850663, 0.1748403687610542, -9.058322217058828, 30.432506602482327, 4.065209375618113, -24.97703184929414], [11.908544317390072, 0.07751886164654587, 0.10382197212254562, -9.018867549696965, 31.01775066278244, 4.065209377729995, -25.027994125453745], [11.517285589546864, 0.07620370619168815, 0.053846062682992246, -8.755836427356286, 30.71197708064457, 4.36775795855366, -24.986895515621658], [11.560028138437199, 0.23139205598442597, 0.23533752222339366, -8.85447309751473, 30.34373362603635, 4.012592231634331, -24.994293265400287], [11.612634353744959, 0.06436730664513302, 0.1511675705387428, -8.795291095873784, 30.09385413866607, 5.26224941256398, -24.986073543431413], [11.14575419083212, 0.08935526102293251, 0.23665267860454015, -9.15367099841794, 30.84678048822279, 4.9860094050622905, -25.0148425702807], [11.458103596000184, 0.09856135004284061, 0.16826459203395389, -9.36738378548769, 30.43579449019589, 4.354603672074128, -25.008266792723827], [11.85593810084857, 0.1537978814704576, 0.16563428091212362, -8.551987307396864, 30.304278970029795, 4.03890080276892, -25.009088764937687], [11.418648934636014, 0.18799192427945738, 0.27873765469616596, -8.571714642268743, 30.406203497590322, 4.367757957489003, -25.024706236648075], [11.543588696420077, 0.128809926410559, 0.17747068020813594, -8.749260649044425, 30.465385482466594, 3.841586512518262, -25.02059637565787], [11.172057298770568, 0.10382197215046701, 0.16694943650409555, -9.245731891568202, 30.646219321631442, 4.1046722355501695, -25.02717215323209], [11.155617855967604, 0.24191330044466786, 0.2682164106218414, -8.91694298854727, 31.070356871484723, 5.01231797700449, -25.016486514677332], [11.711271008976384, 0.2235011231321955, 0.10776743851127296, -8.52568419649002, 30.86321992823627, 5.5121808488265405, -24.991005376603955], [11.418648934946091, 0.23665267741524926, 0.12486446027824794, -8.32512296685944, 30.87308359227051, 4.394066529645393, -25.005800876132778], [11.145754190916463, 0.22087081220746674, 0.22876174538069893, -8.834745763061283, 30.843492599553635, 5.130706552265816, -25.011554681502048], [11.90854431509472, 0.0472702849427698, 0.03674904091260378, -8.795291094969189, 30.455521817389908, 4.091517949159994, -25.000047070780536], [11.816483439847964, 0.15116757015719096, 0.1669494363685458, -8.792003205870916, 30.827053158803597, 4.722923681839544, -24.98853946001873], [11.41864893525873, 0.178785836086701, 0.15248272592096707, -8.768987983101944, 30.771159064805442, 3.986283659637947, -24.99675918197245], [11.33645172309687, 0.340549962706821, 0.19719801326954994, -8.358001856998989, 30.62977988150551, 4.736077969057269, -24.966346210757603], [11.214799849059665, 0.2471739219850403, 0.18141614725327843, -8.916942989509192, 30.53114324096059, 4.972855119092857, -24.98936143223335], [11.379194273386853, 0.2511193891141257, 0.11434321614756815, -8.522396307125371, 30.889523030958106, 3.460112213282519, -24.98114171025887], [11.800043997824169, 0.19193739071623328, -0.03558451214834635, -8.117985958355897, 30.61334044186562, 4.183597952384781, -24.984429599040052], [11.711271008800436, 0.1551130366196825, 0.08277948383942435, -8.867624653624615, 30.024808490326027, 4.249369381670053, -25.021418347856677], [11.632361686030686, 0.15511303675805554, 0.2524345444910084, -8.768987984084497, 30.807325832476362, 4.052055090601465, -25.000869042978024], [11.073420643840732, 0.2129798792550458, 0.2971498317249395, -9.012291770868641, 31.165705621323347, 4.341449385776823, -25.021418347854812], [11.767165111725914, 0.24848907789912678, 0.11960383801222474, -8.321835077205828, 30.665946648106452, 5.196477981024213, -24.97538790488818], [11.402209492591172, 0.08935526147588507, 0.07225823994103198, -8.989276547617036, 30.228657546723248, 4.788695113681438, -25.02470623665884], [11.711271007526761, 0.23533752259933344, 0.16168881423757925, -8.949821878794287, 30.610052552396176, 4.236215095546468, -25.01648651468425], [11.770453000183752, 0.30635592007560886, 0.09593103880759979, -9.143807331527704, 30.89281092037307, 4.56507224800046, -24.991827348795518], [11.349603276208908, 0.15905850325066206, 0.26164063304684226, -9.245731892003494, 30.68567397591816, 4.236215095656783, -24.99758115417038], [11.86251387637984, 0.2287617452134746, 0.03806419631079999, -8.193607405778442, 30.94870501493966, 3.0260207714561433, -24.986073543432948], [11.37919427317358, 0.011761086239782781, 0.13275539322766905, -8.621032976635398, 30.300991082352287, 4.065209377238962, -24.997581154171588], [11.398921603553063, 0.22087081247437007, 0.24717392252141368, -8.821594206989229, 31.053917430742782, 4.6834608249906715, -25.000047070781523], [11.458103596796443, 0.19719801328848768, 0.06173699540463018, -8.50266897292319, 30.935553461703115, 3.7758150823844114, -24.99347129321268], [11.408785269595885, 0.18799192425323796, 0.11960383810208153, -8.37115341298415, 30.846780487435847, 4.4072208158741075, -24.998403126370068], [11.329875945925302, 0.237967833995904, 0.12486446015551261, -8.821594206780393, 30.80732583270926, 4.209906524612732, -24.992649320995312], [11.638937462629777, 0.06436730674095992, 0.09856135007442263, -8.755836427597014, 30.55744634582031, 5.038626548997431, -25.014842570283008], [11.796756108455565, 0.3116165422480415, 0.18010099157896348, -8.0883949574532, 31.698343473659857, 4.472992243766015, -24.962236349771906], [11.599482799000604, 0.08409463871132272, 0.17089490221539916, -8.887351988409245, 30.517991690149383, 3.578500789781608, -25.009088764906167], [11.444952042671163, 0.13538570421880242, 0.27084672147264904, -8.765700093546132, 30.902674583936506, 4.17044366511727, -25.000869042963092], [11.231239291803112, 0.252434544208653, 0.28662858769291816, -8.916942988612808, 30.846780488623825, 4.117826521952588, -25.018130459074513], [11.31343650353454, 0.2379678338606241, 0.17352521404449905, -8.893927765978397, 30.93555346351751, 3.4469579278225275, -24.989361432206227], [11.375906384602025, 0.23533752266402275, 0.13538570430900887, -8.535547863013985, 31.040765878233607, 4.104672233721107, -25.011554681513353], [11.52057347746918, 0.08014917269620603, 0.17221005857996868, -8.670351313280648, 30.705401305176615, 4.117826520991506, -24.990183404410196], [11.471255150938076, 0.24717392207389094, 0.21297987928229783, -8.926806655464711, 31.076932647310183, 4.1046722346485085, -25.000047070753634], [11.287133394958165, 0.1511675701862788, 0.2235011234412237, -9.40026267600009, 30.573885785684183, 4.815003684924131, -24.997581154168184], [11.615922242103476, 0.05647637353841539, 0.09461588334135612, -8.874200431906008, 30.55744634517879, 5.485872275070523, -24.999225098558448], [11.546876583980007, 0.07357339528318335, 0.2142950348017792, -8.936670322693745, 30.659370873638537, 4.486146532526341, -25.005800876138817], [11.421936822720905, 0.15642819249365097, 0.13538570398567135, -8.450062748337627, 30.682386089153336, 4.341449386271379, -25.012376653715567], [11.310148615125406, 0.25374969993393626, 0.28794374280928686, -8.512532640390932, 30.905962471852455, 5.117552264753816, -24.99675918197201], [11.76716511228, 0.16957974732571302, 0.16694943644551002, -8.657199756428389, 30.728416519264083, 4.880775115996331, -24.989361432208092], [11.490982479934061, 0.1787858358000965, 0.24454361142236647, -9.179974111215428, 31.234751268893245, 3.8152779361264417, -25.010732709303014], [11.560028139690726, 0.33134387469377685, 0.30109529801135715, -8.84460943093975, 31.432024547567256, 3.8547407986106244, -24.972921988300428], [11.385770050179197, 0.3313438744097542, 0.20640410165593615, -8.844609431009905, 30.820477384314415, 4.236215095677958, -25.0082667927235], [11.300284949653898, 0.13012508225705138, 0.049900596058222224, -8.351426077629307, 30.807325831934858, 4.683460824860909, -25.015664542480387], [11.030678093758395, 0.22744658947548468, 0.33923480747675505, -8.713093869446146, 30.912538248276277, 4.499300819009327, -25.010732709305323], [11.35946694234395, 0.24059814477232838, 0.15248272561325604, -8.551987307951633, 30.744855960447794, 3.354877924995863, -24.981141710255578], [11.622498020339615, 0.017021708165793126, 0.12091899364912789, -9.278610782786505, 30.386476169705272, 4.788695113963726, -25.024706236636984], [11.579755469946917, 0.2300769006059104, 0.1577433480624893, -8.792003205960183, 31.057205317684065, 4.880775115576987, -25.00251298733996], [11.402209492813368, 0.25769516636412887, 0.2669012549856544, -8.821594206718833, 30.54758268190753, 5.15701512330681, -25.01319862589582], [11.800043995237615, 0.11171290504712239, 0.12880992662689095, -8.542123640807631, 30.81061372002808, 5.025472262875462, -25.001691015151913], [11.244390845206713, 0.2090344128298403, 0.3037256088482682, -8.979412880484697, 30.748143848227045, 4.275677954410094, -25.004978903932653], [11.609346467203, 0.18010099172324895, 0.12486446009039087, -8.959685546194859, 30.85335626411434, 4.630843680759256, -24.994293265381405], [11.65866479311011, 0.03280357440263282, 0.22218596749826192, -8.96954921294116, 30.7875985039025, 4.749232254991513, -25.02224032006867], [11.10629952873353, 0.27347703239336, 0.3497560517768321, -8.93338243351008, 31.116387303352443, 3.499575073213294, -25.001691015145543], [11.42193682356332, 0.17484036953538423, 0.1919373906960391, -9.005715993211648, 30.715264968949512, 4.617689392213984, -25.015664542491255], [11.73099834033918, 0.09987650548842059, 0.15905850345697536, -9.035306995188822, 30.636355657195658, 4.262523669492913, -25.009910737114748], [11.84936232252117, 0.21034956800196675, 0.1564281918151939, -8.660487645115253, 30.685673977266053, 4.301986526892172, -24.98607354343833], [11.35617905417838, 0.21561018975228502, 0.03411873003241794, -8.581578308515683, 30.7415680721906, 4.091517947581984, -24.98442959903742], [11.29699706118761, 0.16431912538458043, 0.13538570429321228, -8.42704752802106, 30.741568072919854, 4.025746518762952, -25.00580087614135], [11.546876585693562, 0.34186511861359226, 0.09067041678088777, -8.328410855382772, 30.731704409167428, 4.933392260527465, -24.985251571238752], [11.721134673150898, 0.1682645918377017, 0.2695315659478059, -9.60739968568665, 30.28455164211824, 4.828157971834887, -25.00004707076747], [11.823059216339686, 0.24717392207398825, 0.16563428075831482, -8.489517417563079, 30.882947256110942, 5.1701694105227345, -24.982785654657476], [11.707983119561579, 0.23402236760995765, 0.2432284559833196, -8.627608755172703, 31.00788699987701, 3.657426507340432, -25.009088764910448], [11.290421284441269, 0.09987650500427209, 0.1774706805870071, -8.956397657218574, 30.902674584512663, 4.9202379742915765, -25.00908876491506], [11.16548152165127, 0.0775188615666067, 0.264270943793908, -8.805154762780088, 30.268112201915798, 3.525883646256945, -25.02059637566819], [11.520573477732968, 0.06962792839353787, 0.15116756996958225, -8.637472422625999, 30.29770319431906, 4.196752236693534, -24.985251571242156], [11.813195550937753, 0.33134387486541894, 0.31819231962199335, -9.51205090303682, 31.241327044125534, 4.078363663779943, -25.020596375675442], [11.750725670361513, 0.285313432127965, 0.12880992648807688, -9.426565788045723, 30.642931432932073, 4.565072249275019, -25.001691015153447], [11.464679373297734, 0.03543388556403271, 0.1498524145446124, -8.943246100553404, 30.320718410286506, 3.9468208016720094, -25.014020598085736], [11.707983120273315, 0.16037365896334077, 0.27347703235900456, -8.726245426350872, 30.78431061702222, 3.4469579288330396, -24.991005376598903], [11.537012920026049, 0.1090825941003058, 0.11960383803249924, -8.8215942069853, 30.10371780204651, 4.512455104700029, -24.998403126359747], [11.494270370061477, 0.16300397004828793, 0.07883401718004485, -8.473077972950191, 30.68896186461565, 4.749232254241056, -24.980319738085644], [11.836210770590938, 0.19851316884835912, 0.14196148182293272, -8.696654424751895, 30.804037944643003, 3.999437946798075, -24.997581154167637], [11.42522471206963, 0.12486446005211127, 0.09198557238789651, -8.509244751477352, 30.521279576542103, 4.986009404603116, -24.999225098568], [11.155617856195665, 0.22087081222460714, 0.2274465898824236, -8.502668973176334, 30.846780488696346, 4.565072249595976, -25.016486514679524], [11.553452362974843, 0.34449542979891223, 0.17747068037612834, -8.775563760528753, 31.17556928652799, 4.183597951969075, -25.010732709324646], [11.596194912911525, 0.29978014272881864, 0.27084672125372566, -8.841321542095848, 31.083508423231766, 5.117552264427933, -24.99100537660209], [11.44823992938577, 0.21561019004429166, 0.27216187692798316, -9.012291770231101, 30.85993203960591, 3.9994379464631016, -25.024706236641812], [11.60934646699751, 0.06962792847287347, 0.10382197187906966, -8.93338243435915, 30.692249753324724, 4.788695113825236, -25.03703581959738], [11.694831564492244, 0.14459179288153318, 0.2182405012040617, -8.57500253096183, 31.083508423502586, 4.18359795194629, -25.008266792715812], [11.26740606463148, 0.23402236721526148, 0.18930707990590562, -8.936670322419635, 30.57059789668382, 4.091517949649252, -25.017308486872736], [11.375906384660968, 0.21824050041576087, 0.1603736588060185, -8.456638526592483, 30.72512863343243, 5.3017122683070905, -25.016486514699405], [11.425224711294282, 0.10119166107760674, 0.3089862313457558, -8.900503544568856, 30.794174280990312, 4.499300819432042, -25.029638069865097], [11.540300808152844, 0.25243454434657947, 0.23139205654957679, -9.107640552174761, 31.027614327323256, 3.8152779401133463, -25.010732709307078], [11.533725030177907, 0.12617961562271474, 0.3563318291128851, -9.114216332204967, 31.126250967020212, 4.236215096026853, -25.008266792732837], [11.398921604334603, 0.2011434795873372, 0.1406463260844249, -8.749260648463645, 31.030902215048116, 4.972855118365295, -24.996759181969928], [11.33316383285132, 0.05384606245398338, 0.25769516643082413, -9.357520118567184, 30.38647616945232, 3.749506508555055, -24.99429326538492], [11.431800488125955, 0.1432766371682005, 0.31424685346265024, -8.706518091976125, 30.501552250440177, 4.999163690472176, -24.998403126366664], [11.606058577390261, 0.17878583616794302, 0.2866285874774864, -9.055034327855028, 30.564022121714014, 4.42037510017969, -24.982785654649465], [11.481118816140516, 0.0906704167904901, 0.17878583601155623, -8.979412880373246, 30.58046156153817, 4.749232255692866, -25.010732709300598], [11.579755467848459, 0.1840464579768451, 0.09724619414902508, -9.350944340959918, 30.721840744489782, 4.630843677480602, -25.018952431287378], [11.343027500285325, 0.14327663729732953, 0.16957974752288096, -8.772275872245087, 30.425930826403686, 4.920237974153306, -24.99429326538997], [11.487694591919894, 0.25769516583571334, 0.15905850315673087, -8.838033652415374, 31.08022053532719, 4.670306537176633, -25.032103986409687], [11.484406704971791, 0.29846498644606395, 0.07094308440010588, -8.742684870573544, 31.175569286069084, 4.420375102874492, -25.011554681504677], [11.849362324487407, 0.17747068046836822, 0.04595512964609416, -8.916942989030852, 30.669234537611572, 4.8413122568859395, -25.00662284832928], [11.533725031288554, 0.03674904094338677, 0.157743347893607, -8.890639876230873, 30.531143242223614, 3.8415865129148226, -25.005800876127836], [11.7014073415438, 0.2011434789558082, 0.12486445994424944, -8.77885165003445, 30.603476776826817, 4.722923682395243, -25.000047070751325], [11.747437782603061, 0.0919855723288554, 0.10908259387871733, -9.068185884635607, 30.820477384239307, 4.315140812458583, -25.000047070751986], [11.09314797505468, 0.28662858782642175, 0.31687716444951874, -8.535547862474509, 31.44188821221754, 4.446683673540274, -24.987717487817285], [11.79675610830488, 0.09198557262952861, 0.10119166115415706, -8.897215655685214, 30.541006906062236, 3.907357944199356, -25.00580087613124], [11.06026908838517, 0.11697352704290914, 0.2156101902216262, -9.055034327356278, 30.659370873764978, 4.42037510211005, -25.009088764910558], [11.632361686358243, 0.2853134321102708, 0.05121575168527731, -8.13442540328276, 30.425930824883036, 4.459837961038442, -25.018952431269696], [11.201648295095607, 0.30241045294920244, 0.21561019030531575, -8.77227587183789, 31.034190103355524, 4.315140810969339, -24.981963682456694], [11.839498659879338, 0.1248644599634599, 0.07751886164247068, -8.650623978433462, 30.75143173704218, 3.881049371578521, -24.985251571237104], [11.346315387888879, 0.2537496998115569, 0.2826831209772113, -8.953109768089071, 30.810613719654867, 4.394066528954214, -25.005800876127836], [12.00060519332751, 0.11434321601896952, 0.057791529098336236, -8.657199757011206, 30.93555346276819, 3.775815081563642, -24.97867579368221], [11.103011640732719, 0.17221005790568128, 0.2524345445764208, -9.048458549418468, 30.771159064304303, 4.7360779673089635, -25.020596375663036], [11.507421924052174, 0.17089490252226863, 0.28399827611850115, -8.479653749368588, 30.71197708139678, 4.722923683279063, -25.016486514682825], [11.652089015917188, 0.24191330030214792, 0.22744658967091297, -8.032500844751542, 30.659370873139856, 5.038626545790252, -24.980319738057645], [11.316724392419628, 0.1708949028470434, 0.13538570431377756, -8.450062748230575, 30.78102272768965, 4.2625236691491475, -25.004978903926723], [11.467967262584907, 0.18536161353076042, 0.17089490295722964, -8.611169310022754, 30.991447558792622, 4.499300818600636, -24.991827348801227], [11.625785909506051, 0.23270721178330545, 0.07488855085553692, -8.601305642639312, 30.4062034984116, 4.880775116164571, -24.99758115417609], [11.859225990868616, 0.32739840848242907, 0.13538570424436375, -8.519108417175728, 30.185915002331747, 4.709769396164888, -24.992649320996414], [11.458103596805156, 0.2116647235425605, 0.19456770185395145, -9.097776885360128, 30.57717367339291, 3.8284322241170163, -24.980319738058526], [11.5501644745511, 0.2721618770069232, 0.1551130369602916, -8.016061399297975, 30.55744634524178, 5.420100845583041, -24.984429599035224], [11.602770688456584, 0.24059814499262078, 0.11302806053308351, -8.637472422906765, 30.978296007533366, 4.14413509379294, -24.994293265400728], [11.96772630899543, 0.17221005865860844, 0.06305215112562584, -9.058322217131762, 30.646219321605205, 4.446683674457144, -24.99758115418773], [11.195072517977374, 0.2853134321332215, 0.2313920564839443, -8.722957536626726, 30.912538247672128, 4.801849397945039, -25.005800876135524], [11.320012280642906, 0.12354930419820043, 0.1432766372893684, -9.002428103362824, 30.718552856434094, 4.315140812710606, -25.040323708390645], [11.188496741307489, 0.18930707978089995, 0.2511193891343204, -9.055034327787014, 30.448946041316518, 4.788695113858554, -25.021418347851625], [11.497558257824531, 0.11828868255950598, 0.18667676899179342, -8.815018429688992, 30.639643545794854, 4.130980807955121, -24.9877174878197], [11.267406063720227, 0.14196148148666987, 0.24980423279606873, -9.11092844181608, 31.014462774923064, 3.933666516390441, -24.995115237590422], [11.36275482990431, 0.06568246202485312, 0.14590694819149574, -8.999140214719512, 30.406203498614037, 4.893929402449444, -25.004978903938476], [11.204936183594585, 0.1051371273681091, 0.2669012551762159, -9.147095221059395, 30.751431737351343, 3.657426505935503, -25.01319862591372], [11.517285589539114, 0.24059814496278786, 0.1985131686106945, -8.63747242164603, 30.810613721126785, 4.420375101841641, -24.997581154173783], [11.773740890421443, 0.12091899347679969, 0.13407054878955615, -7.996334066678937, 30.833628935531397, 4.525609391633674, -25.001691015159267], [11.241102956410954, 0.12880992637327449, 0.24848907755622418, -8.782139539880172, 30.60676466551202, 3.275952208185241, -24.99347129319676], [11.67839212467184, 0.2064041015381764, -0.004020779821048592, -8.864336765266529, 30.060975257944804, 4.828157971608747, -25.013198625891096], [11.484406703289492, 0.23928298925898983, 0.23796783383347248, -8.354713967419574, 31.356403124071697, 3.9468208014389856, -24.977853821490974], [11.096435863793715, 0.2116647230978792, 0.3208226306580933, -8.84132154179165, 30.978296007346557, 4.565072249978148, -24.99675918198365], [11.435088376545199, 0.33134387495212697, 0.18536161361692494, -8.532259974014554, 30.856644152003355, 4.775540827433397, -24.994293265406], [11.3364517221564, 0.2248162785367327, 0.28399827647187986, -9.041882772920786, 30.2648243128815, 4.788695112945309, -25.00580087616858], [11.80990766139125, 0.15774334763286918, 0.12091899340597972, -8.706518092475944, 30.33058207302133, 5.130706550562056, -24.99675918197168], [11.369330608034458, 0.03148841826536186, 0.18404645808012693, -9.08462532883361, 30.478537034081064, 5.762112283380259, -25.001691015153888], [11.61592224340429, 0.19719801297252815, 0.27742249865802143, -9.232580336146892, 31.20187239003866, 3.986283659646541, -24.98442959903643], [11.421936823376724, 0.1879919244801982, 0.22876174527001092, -8.601305643183206, 30.672522423161077, 3.420649356729571, -24.979497765870367], [11.77702877808213, 0.1274947712968525, 0.10382197216451916, -8.91036721152831, 30.1990665539991, 3.9205122303334816, -24.981963682464485], [11.69811945345154, 0.17352521262931386, 0.11171290453215404, -8.57500253091416, 30.208930218315476, 5.972580861862573, -24.977031849278113], [11.333163833739341, 0.21034956810525185, 0.21166472384004054, -9.291762338059458, 30.524567465730723, 4.17044366635404, -25.002512987341273], [11.356179053514978, 0.12749477114985602, 0.10908259416207805, -8.690078646650202, 30.810613720429025, 3.8415865125798074, -25.027994125430464], [11.658664792358895, 0.17484036899011635, 0.1787858358889644, -8.397456524856228, 30.90267458415224, 4.959700832613363, -25.0090887649211], [11.359466942241724, 0.16037365880802834, 0.17089490310189165, -8.4073201913481, 30.639643545133268, 4.893929399210605, -24.978675793672327], [11.241102957044044, 0.2445436113453872, 0.21692534557855764, -8.834745763764376, 31.017750663973416, 4.920237974708915, -24.998403126367432], [11.241102957226449, 0.22350112318559157, 0.16037365904547501, -8.196895294759761, 30.902674583871704, 3.959975086852558, -25.007444820538193], [11.487694593418732, 0.2550648556357621, 0.10250681587289223, -8.427047525875617, 30.823765272497322, 3.999437946410437, -24.995937209799006], [11.152329967870063, 0.11171290523935917, 0.17878583611105814, -9.05174643909739, 30.96843234413134, 4.538763676738756, -25.00826679271856], [11.89539276347589, 0.32345294172373057, 0.10908259425233952, -8.078531290172874, 30.67252242542781, 4.6176893939659465, -24.97538790488763], [11.671816346582704, 0.28005280999965787, 0.19193739117000402, -8.676927090112919, 31.211736054181717, 4.762386540780137, -24.991005376603077], [11.40220949274411, 0.22876174533962534, 0.13144023776298913, -8.305395632258197, 31.10323575021625, 4.446683673869909, -24.99758115418048], [11.721134673315925, 0.19062223563006309, 0.18141614711584314, -8.84132154154352, 30.682386088191784, 4.4729922469200645, -25.00333495954371], [11.004374985914637, 0.09067041689516553, 0.2537496998499311, -9.443005234009394, 30.945417128464413, 4.117826517814258, -25.00497890392925], [11.257542399295946, 0.08277948398391322, 0.2366526779827482, -9.193125667401695, 30.978296007353173, 4.341449384297049, -25.018130459066384], [11.711271007354608, 0.12223414848268854, 0.14722210382738304, -8.709805980987666, 30.938841351758807, 4.3940665288602405, -25.010732709307298], [11.45810359526331, 0.30372560910363683, 0.21166472382912022, -8.864336764416237, 30.988159671725146, 4.249369381640462, -25.032103986422864], [11.35946694179879, 0.07357339521628603, 0.19719801282129312, -9.63041490910859, 30.573885785553962, 4.36775795819416, -25.011554681499522], [11.905256428560644, 0.1419614813224393, 0.10908259325161285, -9.219428778896406, 30.577173672493814, 4.7623865407417, -24.99675918197388], [11.510709812737748, 0.15511303633386175, 0.10119166049372252, -8.775563761017017, 30.688961865688132, 4.551917964177176, -25.00004707075572], [11.19836040673518, 0.11828868255891761, 0.2077192572508642, -8.9761249919838, 30.343733624764447, 4.565072248770149, -25.003334959552166], [11.556740250782022, 0.21561018999217474, 0.2550648553603271, -8.772275872379756, 30.994735446123922, 4.3940665293948244, -25.032103986427153], [12.211030056316918, 0.1459069477976267, 0.07751886180827244, -8.910367211114526, 30.419355050552312, 4.43352938579152, -25.00086904298835], [11.707983119420854, 0.23270721193125354, 0.14853725916171645, -8.28238040883798, 30.79746216721042, 3.6837350793543293, -25.001691015148175], [11.563316028234391, 0.386580406013938, 0.19062223546802864, -8.463214304279017, 31.04734165451921, 3.4601122144512226, -25.01155468150215], [11.61921013139235, 0.1787858358753186, 0.21034956823906042, -8.617745088139705, 31.27420592396069, -0.854493657827594, -25.002512987364007]]
  out "TimeArray (USB6218)":timestamp[](array[timestamp])=[timestamp(3682722291.269417 s since 1904-01-01), timestamp(3682722291.6090097 s since 1904-01-01), timestamp(3682722291.909876 s since 1904-01-01), timestamp(3682722292.2170215 s since 1904-01-01), timestamp(3682722293.6133137 s since 1904-01-01), timestamp(3682722293.9179463 s since 1904-01-01), timestamp(3682722294.219336 s since 1904-01-01), timestamp(3682722294.528156 s since 1904-01-01), timestamp(3682722294.8491826 s since 1904-01-01), timestamp(3682722295.1502175 s since 1904-01-01), timestamp(3682722295.450474 s since 1904-01-01), timestamp(3682722295.7592254 s since 1904-01-01), timestamp(3682722296.078004 s since 1904-01-01), timestamp(3682722297.49354 s since 1904-01-01), timestamp(3682722298.3642545 s since 1904-01-01), timestamp(3682722298.6638055 s since 1904-01-01), timestamp(3682722298.9826818 s since 1904-01-01), timestamp(3682722299.3095007 s since 1904-01-01), timestamp(3682722299.607537 s since 1904-01-01), timestamp(3682722299.9149704 s since 1904-01-01), timestamp(3682722301.2983103 s since 1904-01-01), timestamp(3682722302.4433274 s since 1904-01-01), timestamp(3682722302.8488145 s since 1904-01-01), timestamp(3682722303.9812856 s since 1904-01-01), timestamp(3682722304.305741 s since 1904-01-01), timestamp(3682722304.6206574 s since 1904-01-01), timestamp(3682722304.9363046 s since 1904-01-01), timestamp(3682722306.086776 s since 1904-01-01), timestamp(3682722306.4063826 s since 1904-01-01), timestamp(3682722306.711479 s since 1904-01-01), timestamp(3682722307.0166626 s since 1904-01-01), timestamp(3682722307.3209543 s since 1904-01-01), timestamp(3682722307.6242127 s since 1904-01-01), timestamp(3682722307.9394455 s since 1904-01-01), timestamp(3682722308.2527823 s since 1904-01-01), timestamp(3682722309.0702834 s since 1904-01-01), timestamp(3682722309.403611 s since 1904-01-01), timestamp(3682722309.7063704 s since 1904-01-01), timestamp(3682722310.0072503 s since 1904-01-01), timestamp(3682722310.340029 s since 1904-01-01), timestamp(3682722310.640317 s since 1904-01-01), timestamp(3682722311.8439727 s since 1904-01-01), timestamp(3682722312.153859 s since 1904-01-01), timestamp(3682722312.456537 s since 1904-01-01), timestamp(3682722312.767045 s since 1904-01-01), timestamp(3682722313.072183 s since 1904-01-01), timestamp(3682722313.37411 s since 1904-01-01), timestamp(3682722313.7055745 s since 1904-01-01), timestamp(3682722314.006999 s since 1904-01-01), timestamp(3682722314.340123 s since 1904-01-01), timestamp(3682722314.6395106 s since 1904-01-01), timestamp(3682722314.9560866 s since 1904-01-01), timestamp(3682722315.2667 s since 1904-01-01), timestamp(3682722315.586967 s since 1904-01-01), timestamp(3682722315.9260817 s since 1904-01-01), timestamp(3682722316.2263846 s since 1904-01-01), timestamp(3682722316.5273294 s since 1904-01-01), timestamp(3682722316.824146 s since 1904-01-01), timestamp(3682722318.060288 s since 1904-01-01), timestamp(3682722318.36248 s since 1904-01-01), timestamp(3682722318.676595 s since 1904-01-01), timestamp(3682722318.9848504 s since 1904-01-01), timestamp(3682722319.3245873 s since 1904-01-01), timestamp(3682722319.6388264 s since 1904-01-01), timestamp(3682722319.9543386 s since 1904-01-01), timestamp(3682722320.2624993 s since 1904-01-01), timestamp(3682722320.606464 s since 1904-01-01), timestamp(3682722320.9279394 s since 1904-01-01), timestamp(3682722321.2265406 s since 1904-01-01), timestamp(3682722321.5345297 s since 1904-01-01), timestamp(3682722321.853625 s since 1904-01-01), timestamp(3682722322.159787 s since 1904-01-01), timestamp(3682722322.4765434 s since 1904-01-01), timestamp(3682722322.774765 s since 1904-01-01), timestamp(3682722323.076607 s since 1904-01-01), timestamp(3682722323.3740945 s since 1904-01-01), timestamp(3682722323.7074966 s since 1904-01-01), timestamp(3682722324.009541 s since 1904-01-01), timestamp(3682722324.3072734 s since 1904-01-01), timestamp(3682722324.6249175 s since 1904-01-01), timestamp(3682722324.94047 s since 1904-01-01), timestamp(3682722325.239233 s since 1904-01-01), timestamp(3682722325.537832 s since 1904-01-01), timestamp(3682722325.8409486 s since 1904-01-01), timestamp(3682722326.15796 s since 1904-01-01), timestamp(3682722326.469768 s since 1904-01-01), timestamp(3682722326.7745266 s since 1904-01-01), timestamp(3682722327.07472 s since 1904-01-01), timestamp(3682722327.3775873 s since 1904-01-01), timestamp(3682722327.680513 s since 1904-01-01), timestamp(3682722328.0083985 s since 1904-01-01), timestamp(3682722328.3129334 s since 1904-01-01), timestamp(3682722328.611471 s since 1904-01-01), timestamp(3682722328.922543 s since 1904-01-01), timestamp(3682722329.227749 s since 1904-01-01), timestamp(3682722329.5414734 s since 1904-01-01), timestamp(3682722329.8565145 s since 1904-01-01), timestamp(3682722330.1604033 s since 1904-01-01), timestamp(3682722330.476668 s since 1904-01-01), timestamp(3682722330.774875 s since 1904-01-01), timestamp(3682722331.0763545 s since 1904-01-01), timestamp(3682722331.376464 s since 1904-01-01), timestamp(3682722331.708552 s since 1904-01-01), timestamp(3682722332.0103297 s since 1904-01-01), timestamp(3682722332.3245473 s since 1904-01-01), timestamp(3682722332.627525 s since 1904-01-01), timestamp(3682722332.925225 s since 1904-01-01), timestamp(3682722333.2296343 s since 1904-01-01), timestamp(3682722333.5364175 s since 1904-01-01), timestamp(3682722333.8591824 s since 1904-01-01), timestamp(3682722334.174748 s since 1904-01-01), timestamp(3682722334.509348 s since 1904-01-01), timestamp(3682722334.8232136 s since 1904-01-01), timestamp(3682722335.1275034 s since 1904-01-01), timestamp(3682722335.4384727 s since 1904-01-01), timestamp(3682722335.761193 s since 1904-01-01), timestamp(3682722336.0714703 s since 1904-01-01), timestamp(3682722336.3734264 s since 1904-01-01), timestamp(3682722336.6838417 s since 1904-01-01), timestamp(3682722337.0125136 s since 1904-01-01), timestamp(3682722337.312355 s since 1904-01-01), timestamp(3682722337.6117897 s since 1904-01-01), timestamp(3682722337.911963 s since 1904-01-01), timestamp(3682722338.212713 s since 1904-01-01), timestamp(3682722338.515533 s since 1904-01-01), timestamp(3682722338.837754 s since 1904-01-01), timestamp(3682722339.1613526 s since 1904-01-01), timestamp(3682722339.473036 s since 1904-01-01), timestamp(3682722339.7738833 s since 1904-01-01), timestamp(3682722340.0778775 s since 1904-01-01), timestamp(3682722340.3737345 s since 1904-01-01), timestamp(3682722340.6766768 s since 1904-01-01), timestamp(3682722340.978561 s since 1904-01-01), timestamp(3682722341.27956 s since 1904-01-01), timestamp(3682722341.5866785 s since 1904-01-01), timestamp(3682722341.910305 s since 1904-01-01), timestamp(3682722342.226322 s since 1904-01-01), timestamp(3682722342.523912 s since 1904-01-01), timestamp(3682722342.842628 s since 1904-01-01), timestamp(3682722343.1561103 s since 1904-01-01), timestamp(3682722343.4603863 s since 1904-01-01), timestamp(3682722343.775651 s since 1904-01-01), timestamp(3682722344.0775495 s since 1904-01-01), timestamp(3682722344.375196 s since 1904-01-01), timestamp(3682722344.675948 s since 1904-01-01), timestamp(3682722345.75802 s since 1904-01-01), timestamp(3682722346.0932946 s since 1904-01-01), timestamp(3682722346.415583 s since 1904-01-01), timestamp(3682722346.7194586 s since 1904-01-01), timestamp(3682722347.059891 s since 1904-01-01), timestamp(3682722347.372628 s since 1904-01-01), timestamp(3682722347.6744647 s since 1904-01-01), timestamp(3682722348.1986303 s since 1904-01-01), timestamp(3682722348.712384 s since 1904-01-01), timestamp(3682722349.0128455 s since 1904-01-01), timestamp(3682722349.3274846 s since 1904-01-01), timestamp(3682722349.629469 s since 1904-01-01), timestamp(3682722349.9287167 s since 1904-01-01), timestamp(3682722350.2305937 s since 1904-01-01), timestamp(3682722350.5342593 s since 1904-01-01), timestamp(3682722350.832652 s since 1904-01-01), timestamp(3682722351.1315007 s since 1904-01-01), timestamp(3682722351.4424863 s since 1904-01-01), timestamp(3682722351.755626 s since 1904-01-01), timestamp(3682722352.058862 s since 1904-01-01), timestamp(3682722352.361109 s since 1904-01-01), timestamp(3682722352.6776423 s since 1904-01-01), timestamp(3682722352.9804754 s since 1904-01-01), timestamp(3682722353.289053 s since 1904-01-01), timestamp(3682722353.6086473 s since 1904-01-01), timestamp(3682722353.9139414 s since 1904-01-01), timestamp(3682722354.212695 s since 1904-01-01), timestamp(3682722354.526895 s since 1904-01-01), timestamp(3682722354.8239746 s since 1904-01-01), timestamp(3682722355.1460752 s since 1904-01-01), timestamp(3682722355.4592047 s since 1904-01-01), timestamp(3682722355.762469 s since 1904-01-01), timestamp(3682722356.0803466 s since 1904-01-01), timestamp(3682722356.3786144 s since 1904-01-01), timestamp(3682722356.676559 s since 1904-01-01), timestamp(3682722356.9803343 s since 1904-01-01), timestamp(3682722357.282457 s since 1904-01-01), timestamp(3682722357.578398 s since 1904-01-01), timestamp(3682722357.9105134 s since 1904-01-01), timestamp(3682722358.2273817 s since 1904-01-01), timestamp(3682722358.5446 s since 1904-01-01), timestamp(3682722358.843864 s since 1904-01-01), timestamp(3682722359.1465826 s since 1904-01-01), timestamp(3682722359.4641614 s since 1904-01-01), timestamp(3682722359.77346 s since 1904-01-01), timestamp(3682722360.075001 s since 1904-01-01), timestamp(3682722360.37332 s since 1904-01-01), timestamp(3682722361.6928 s since 1904-01-01), timestamp(3682722363.1191063 s since 1904-01-01), timestamp(3682722363.4209495 s since 1904-01-01), timestamp(3682722363.7262216 s since 1904-01-01), timestamp(3682722364.0422 s since 1904-01-01), timestamp(3682722364.3445926 s since 1904-01-01), timestamp(3682722364.640804 s since 1904-01-01), timestamp(3682722364.944861 s since 1904-01-01), timestamp(3682722365.3566194 s since 1904-01-01), timestamp(3682722365.6562753 s since 1904-01-01), timestamp(3682722365.95898 s since 1904-01-01), timestamp(3682722366.266608 s since 1904-01-01), timestamp(3682722366.57009 s since 1904-01-01), timestamp(3682722366.8765793 s since 1904-01-01), timestamp(3682722367.2081814 s since 1904-01-01), timestamp(3682722367.5267887 s since 1904-01-01), timestamp(3682722367.8403583 s since 1904-01-01), timestamp(3682722368.1564255 s since 1904-01-01), timestamp(3682722368.4612904 s since 1904-01-01), timestamp(3682722368.762861 s since 1904-01-01), timestamp(3682722369.077429 s since 1904-01-01), timestamp(3682722369.379464 s since 1904-01-01), timestamp(3682722369.6796794 s since 1904-01-01), timestamp(3682722369.9800215 s since 1904-01-01), timestamp(3682722370.281791 s since 1904-01-01), timestamp(3682722370.5837607 s since 1904-01-01), timestamp(3682722371.765492 s since 1904-01-01), timestamp(3682722372.0675383 s since 1904-01-01), timestamp(3682722372.373628 s since 1904-01-01), timestamp(3682722372.677635 s since 1904-01-01), timestamp(3682722372.9801407 s since 1904-01-01), timestamp(3682722373.282252 s since 1904-01-01), timestamp(3682722373.5831704 s since 1904-01-01), timestamp(3682722373.890516 s since 1904-01-01), timestamp(3682722374.2132273 s since 1904-01-01), timestamp(3682722374.525751 s since 1904-01-01), timestamp(3682722374.830208 s since 1904-01-01), timestamp(3682722375.143437 s since 1904-01-01), timestamp(3682722375.4440994 s since 1904-01-01), timestamp(3682722375.761483 s since 1904-01-01), timestamp(3682722376.0634546 s since 1904-01-01), timestamp(3682722376.3777046 s since 1904-01-01), timestamp(3682722376.6763616 s since 1904-01-01), timestamp(3682722376.9812737 s since 1904-01-01), timestamp(3682722377.2816544 s since 1904-01-01), timestamp(3682722377.907652 s since 1904-01-01), timestamp(3682722378.3451457 s since 1904-01-01), timestamp(3682722378.666877 s since 1904-01-01), timestamp(3682722378.9770503 s since 1904-01-01), timestamp(3682722379.278165 s since 1904-01-01), timestamp(3682722379.5815215 s since 1904-01-01), timestamp(3682722379.8790617 s since 1904-01-01), timestamp(3682722380.1838393 s since 1904-01-01), timestamp(3682722380.484638 s since 1904-01-01), timestamp(3682722380.791707 s since 1904-01-01), timestamp(3682722381.1058064 s since 1904-01-01), timestamp(3682722382.1073337 s since 1904-01-01), timestamp(3682722383.108455 s since 1904-01-01), timestamp(3682722384.109976 s since 1904-01-01), timestamp(3682722385.111748 s since 1904-01-01), timestamp(3682722386.110368 s since 1904-01-01), timestamp(3682722387.113498 s since 1904-01-01), timestamp(3682722388.110863 s since 1904-01-01), timestamp(3682722389.1160274 s since 1904-01-01), timestamp(3682722392.0222664 s since 1904-01-01), timestamp(3682722393.0877514 s since 1904-01-01), timestamp(3682722394.468309 s since 1904-01-01), timestamp(3682722395.472353 s since 1904-01-01), timestamp(3682722396.4754257 s since 1904-01-01), timestamp(3682722398.0146966 s since 1904-01-01), timestamp(3682722399.016179 s since 1904-01-01), timestamp(3682722400.01852 s since 1904-01-01), timestamp(3682722401.019458 s since 1904-01-01), timestamp(3682722402.0224977 s since 1904-01-01), timestamp(3682722403.0235906 s since 1904-01-01), timestamp(3682722404.0247984 s since 1904-01-01), timestamp(3682722405.0265346 s since 1904-01-01), timestamp(3682722406.027513 s since 1904-01-01), timestamp(3682722407.0285106 s since 1904-01-01), timestamp(3682722408.0305967 s since 1904-01-01), timestamp(3682722409.0293097 s since 1904-01-01), timestamp(3682722410.0282626 s since 1904-01-01), timestamp(3682722411.031312 s since 1904-01-01), timestamp(3682722412.032471 s since 1904-01-01), timestamp(3682722413.0294766 s since 1904-01-01), timestamp(3682722414.033274 s since 1904-01-01), timestamp(3682722415.032189 s since 1904-01-01), timestamp(3682722416.0382686 s since 1904-01-01), timestamp(3682722417.0385666 s since 1904-01-01), timestamp(3682722418.038904 s since 1904-01-01), timestamp(3682722419.0365458 s since 1904-01-01), timestamp(3682722420.0365386 s since 1904-01-01), timestamp(3682722421.039256 s since 1904-01-01), timestamp(3682722422.0376897 s since 1904-01-01), timestamp(3682722423.037548 s since 1904-01-01), timestamp(3682722424.0368495 s since 1904-01-01), timestamp(3682722425.041404 s since 1904-01-01), timestamp(3682722426.042352 s since 1904-01-01), timestamp(3682722427.1176 s since 1904-01-01), timestamp(3682722428.1180434 s since 1904-01-01), timestamp(3682722429.1272926 s since 1904-01-01), timestamp(3682722430.1267505 s since 1904-01-01), timestamp(3682722431.130331 s since 1904-01-01), timestamp(3682722432.170221 s since 1904-01-01), timestamp(3682722433.5435047 s since 1904-01-01), timestamp(3682722434.544317 s since 1904-01-01), timestamp(3682722435.547687 s since 1904-01-01), timestamp(3682722436.5455537 s since 1904-01-01), timestamp(3682722437.8944626 s since 1904-01-01), timestamp(3682722438.894748 s since 1904-01-01), timestamp(3682722439.8967633 s since 1904-01-01), timestamp(3682722440.897467 s since 1904-01-01), timestamp(3682722441.9001656 s since 1904-01-01), timestamp(3682722442.8984895 s since 1904-01-01), timestamp(3682722443.9515 s since 1904-01-01), timestamp(3682722444.9524393 s since 1904-01-01), timestamp(3682722445.951253 s since 1904-01-01), timestamp(3682722446.9551663 s since 1904-01-01), timestamp(3682722447.9556985 s since 1904-01-01), timestamp(3682722448.9578447 s since 1904-01-01), timestamp(3682722449.9597225 s since 1904-01-01), timestamp(3682722451.01432 s since 1904-01-01), timestamp(3682722452.0182304 s since 1904-01-01), timestamp(3682722453.018864 s since 1904-01-01), timestamp(3682722454.021084 s since 1904-01-01), timestamp(3682722455.134126 s since 1904-01-01), timestamp(3682722456.1330423 s since 1904-01-01), timestamp(3682722457.134115 s since 1904-01-01), timestamp(3682722458.1349463 s since 1904-01-01), timestamp(3682722459.136244 s since 1904-01-01), timestamp(3682722460.136195 s since 1904-01-01), timestamp(3682722461.139483 s since 1904-01-01), timestamp(3682722462.1393704 s since 1904-01-01), timestamp(3682722463.139332 s since 1904-01-01), timestamp(3682722464.1406846 s since 1904-01-01), timestamp(3682722465.14165 s since 1904-01-01), timestamp(3682722466.142207 s since 1904-01-01), timestamp(3682722467.1460376 s since 1904-01-01), timestamp(3682722468.1418934 s since 1904-01-01), timestamp(3682722469.4107466 s since 1904-01-01)]
  out "Data Array sizes (6210)":i32[](array[numeric])=[332, 13]
  out "DataArraySize (6218)":i32[](array[numeric])=[332, 7]
  out "TimeArray size (6218)":i32=332
  out "TimeArray (LSI336)":timestamp[](array[timestamp])=[timestamp(3682722291.2644224 s since 1904-01-01), timestamp(3682722291.604032 s since 1904-01-01), timestamp(3682722291.9037905 s since 1904-01-01), timestamp(3682722292.2130303 s since 1904-01-01), timestamp(3682722293.6093 s since 1904-01-01), timestamp(3682722293.911434 s since 1904-01-01), timestamp(3682722294.215163 s since 1904-01-01), timestamp(3682722294.522572 s since 1904-01-01), timestamp(3682722294.8441634 s since 1904-01-01), timestamp(3682722295.1448545 s since 1904-01-01), timestamp(3682722295.44568 s since 1904-01-01), timestamp(3682722295.7512665 s since 1904-01-01), timestamp(3682722296.071016 s since 1904-01-01), timestamp(3682722297.4895544 s since 1904-01-01), timestamp(3682722298.3582816 s since 1904-01-01), timestamp(3682722298.6583776 s since 1904-01-01), timestamp(3682722298.976703 s since 1904-01-01), timestamp(3682722299.303491 s since 1904-01-01), timestamp(3682722299.6028943 s since 1904-01-01), timestamp(3682722299.9109864 s since 1904-01-01), timestamp(3682722301.2943215 s since 1904-01-01), timestamp(3682722302.439338 s since 1904-01-01), timestamp(3682722302.84283 s since 1904-01-01), timestamp(3682722303.976296 s since 1904-01-01), timestamp(3682722304.298886 s since 1904-01-01), timestamp(3682722304.6146727 s since 1904-01-01), timestamp(3682722304.9304714 s since 1904-01-01), timestamp(3682722306.0827866 s since 1904-01-01), timestamp(3682722306.400269 s since 1904-01-01), timestamp(3682722306.701908 s since 1904-01-01), timestamp(3682722307.01266 s since 1904-01-01), timestamp(3682722307.3139567 s since 1904-01-01), timestamp(3682722307.617281 s since 1904-01-01), timestamp(3682722307.9324656 s since 1904-01-01), timestamp(3682722308.2477794 s since 1904-01-01), timestamp(3682722309.066163 s since 1904-01-01), timestamp(3682722309.3965664 s since 1904-01-01), timestamp(3682722309.7003713 s since 1904-01-01), timestamp(3682722310.0011826 s since 1904-01-01), timestamp(3682722310.3316903 s since 1904-01-01), timestamp(3682722310.6338625 s since 1904-01-01), timestamp(3682722311.8390217 s since 1904-01-01), timestamp(3682722312.147876 s since 1904-01-01), timestamp(3682722312.4494967 s since 1904-01-01), timestamp(3682722312.760971 s since 1904-01-01), timestamp(3682722313.065274 s since 1904-01-01), timestamp(3682722313.3656464 s since 1904-01-01), timestamp(3682722313.6989264 s since 1904-01-01), timestamp(3682722314.00116 s since 1904-01-01), timestamp(3682722314.3316183 s since 1904-01-01), timestamp(3682722314.632463 s since 1904-01-01), timestamp(3682722314.9485526 s since 1904-01-01), timestamp(3682722315.2606983 s since 1904-01-01), timestamp(3682722315.5799346 s since 1904-01-01), timestamp(3682722315.9180913 s since 1904-01-01), timestamp(3682722316.2203927 s since 1904-01-01), timestamp(3682722316.5203104 s since 1904-01-01), timestamp(3682722316.8202634 s since 1904-01-01), timestamp(3682722318.055342 s since 1904-01-01), timestamp(3682722318.3566217 s since 1904-01-01), timestamp(3682722318.67011 s since 1904-01-01), timestamp(3682722318.979581 s since 1904-01-01), timestamp(3682722319.3166094 s since 1904-01-01), timestamp(3682722319.6308255 s since 1904-01-01), timestamp(3682722319.948837 s since 1904-01-01), timestamp(3682722320.2572136 s since 1904-01-01), timestamp(3682722320.599373 s since 1904-01-01), timestamp(3682722320.919993 s since 1904-01-01), timestamp(3682722321.220749 s since 1904-01-01), timestamp(3682722321.5287714 s since 1904-01-01), timestamp(3682722321.8486905 s since 1904-01-01), timestamp(3682722322.1527696 s since 1904-01-01), timestamp(3682722322.4684625 s since 1904-01-01), timestamp(3682722322.7676926 s since 1904-01-01), timestamp(3682722323.0695057 s since 1904-01-01), timestamp(3682722323.3691983 s since 1904-01-01), timestamp(3682722323.699779 s since 1904-01-01), timestamp(3682722324.00254 s since 1904-01-01), timestamp(3682722324.302169 s since 1904-01-01), timestamp(3682722324.6159334 s since 1904-01-01), timestamp(3682722324.9335217 s since 1904-01-01), timestamp(3682722325.2332306 s since 1904-01-01), timestamp(3682722325.5330367 s since 1904-01-01), timestamp(3682722325.832957 s since 1904-01-01), timestamp(3682722326.1509953 s since 1904-01-01), timestamp(3682722326.4644866 s since 1904-01-01), timestamp(3682722326.767284 s since 1904-01-01), timestamp(3682722327.067716 s since 1904-01-01), timestamp(3682722327.3710494 s since 1904-01-01), timestamp(3682722327.6760697 s since 1904-01-01), timestamp(3682722328.0013742 s since 1904-01-01), timestamp(3682722328.3049417 s since 1904-01-01), timestamp(3682722328.605616 s since 1904-01-01), timestamp(3682722328.915824 s since 1904-01-01), timestamp(3682722329.2197704 s since 1904-01-01), timestamp(3682722329.533479 s since 1904-01-01), timestamp(3682722329.8484006 s since 1904-01-01), timestamp(3682722330.1537294 s since 1904-01-01), timestamp(3682722330.4685154 s since 1904-01-01), timestamp(3682722330.767936 s since 1904-01-01), timestamp(3682722331.0694575 s since 1904-01-01), timestamp(3682722331.371037 s since 1904-01-01), timestamp(3682722331.701168 s since 1904-01-01), timestamp(3682722332.003296 s since 1904-01-01), timestamp(3682722332.3189206 s since 1904-01-01), timestamp(3682722332.6204143 s since 1904-01-01), timestamp(3682722332.9201455 s since 1904-01-01), timestamp(3682722333.222704 s since 1904-01-01), timestamp(3682722333.5307713 s since 1904-01-01), timestamp(3682722333.850218 s since 1904-01-01), timestamp(3682722334.1687818 s since 1904-01-01), timestamp(3682722334.50168 s since 1904-01-01), timestamp(3682722334.8162985 s since 1904-01-01), timestamp(3682722335.1198063 s since 1904-01-01), timestamp(3682722335.433464 s since 1904-01-01), timestamp(3682722335.754174 s since 1904-01-01), timestamp(3682722336.065685 s since 1904-01-01), timestamp(3682722336.3676305 s since 1904-01-01), timestamp(3682722336.678262 s since 1904-01-01), timestamp(3682722337.00354 s since 1904-01-01), timestamp(3682722337.305712 s since 1904-01-01), timestamp(3682722337.6067743 s since 1904-01-01), timestamp(3682722337.906976 s since 1904-01-01), timestamp(3682722338.207723 s since 1904-01-01), timestamp(3682722338.5086007 s since 1904-01-01), timestamp(3682722338.8327622 s since 1904-01-01), timestamp(3682722339.15376 s since 1904-01-01), timestamp(3682722339.4660926 s since 1904-01-01), timestamp(3682722339.7669024 s since 1904-01-01), timestamp(3682722340.0687447 s since 1904-01-01), timestamp(3682722340.3689446 s since 1904-01-01), timestamp(3682722340.669699 s since 1904-01-01), timestamp(3682722340.971668 s since 1904-01-01), timestamp(3682722341.272559 s since 1904-01-01), timestamp(3682722341.5808673 s since 1904-01-01), timestamp(3682722341.9035897 s since 1904-01-01), timestamp(3682722342.2187233 s since 1904-01-01), timestamp(3682722342.519108 s since 1904-01-01), timestamp(3682722342.8346863 s since 1904-01-01), timestamp(3682722343.148861 s since 1904-01-01), timestamp(3682722343.453436 s since 1904-01-01), timestamp(3682722343.7687 s since 1904-01-01), timestamp(3682722344.0703554 s since 1904-01-01), timestamp(3682722344.3712144 s since 1904-01-01), timestamp(3682722344.6709967 s since 1904-01-01), timestamp(3682722345.753763 s since 1904-01-01), timestamp(3682722346.088916 s since 1904-01-01), timestamp(3682722346.411592 s since 1904-01-01), timestamp(3682722346.712583 s since 1904-01-01), timestamp(3682722347.054868 s since 1904-01-01), timestamp(3682722347.366645 s since 1904-01-01), timestamp(3682722347.6665287 s since 1904-01-01), timestamp(3682722348.1936336 s since 1904-01-01), timestamp(3682722348.7083697 s since 1904-01-01), timestamp(3682722349.007952 s since 1904-01-01), timestamp(3682722349.320494 s since 1904-01-01), timestamp(3682722349.6215 s since 1904-01-01), timestamp(3682722349.921623 s since 1904-01-01), timestamp(3682722350.2236137 s since 1904-01-01), timestamp(3682722350.525284 s since 1904-01-01), timestamp(3682722350.8256655 s since 1904-01-01), timestamp(3682722351.126511 s since 1904-01-01), timestamp(3682722351.434491 s since 1904-01-01), timestamp(3682722351.75064 s since 1904-01-01), timestamp(3682722352.0507593 s since 1904-01-01), timestamp(3682722352.3531384 s since 1904-01-01), timestamp(3682722352.6707296 s since 1904-01-01), timestamp(3682722352.9734945 s since 1904-01-01), timestamp(3682722353.2847114 s since 1904-01-01), timestamp(3682722353.600667 s since 1904-01-01), timestamp(3682722353.906944 s since 1904-01-01), timestamp(3682722354.206764 s since 1904-01-01), timestamp(3682722354.518809 s since 1904-01-01), timestamp(3682722354.8189607 s since 1904-01-01), timestamp(3682722355.138008 s since 1904-01-01), timestamp(3682722355.4524865 s since 1904-01-01), timestamp(3682722355.7545385 s since 1904-01-01), timestamp(3682722356.0694222 s since 1904-01-01), timestamp(3682722356.371631 s since 1904-01-01), timestamp(3682722356.671609 s since 1904-01-01), timestamp(3682722356.972576 s since 1904-01-01), timestamp(3682722357.2745256 s since 1904-01-01), timestamp(3682722357.5746017 s since 1904-01-01), timestamp(3682722357.9027176 s since 1904-01-01), timestamp(3682722358.220368 s since 1904-01-01), timestamp(3682722358.536658 s since 1904-01-01), timestamp(3682722358.8382 s since 1904-01-01), timestamp(3682722359.139381 s since 1904-01-01), timestamp(3682722359.4571586 s since 1904-01-01), timestamp(3682722359.7668686 s since 1904-01-01), timestamp(3682722360.068324 s since 1904-01-01), timestamp(3682722360.3683295 s since 1904-01-01), timestamp(3682722361.6878138 s since 1904-01-01), timestamp(3682722363.114297 s since 1904-01-01), timestamp(3682722363.413959 s since 1904-01-01), timestamp(3682722363.7199144 s since 1904-01-01), timestamp(3682722364.037248 s since 1904-01-01), timestamp(3682722364.337508 s since 1904-01-01), timestamp(3682722364.6368146 s since 1904-01-01), timestamp(3682722364.936756 s since 1904-01-01), timestamp(3682722365.3525553 s since 1904-01-01), timestamp(3682722365.6523194 s since 1904-01-01), timestamp(3682722365.953843 s since 1904-01-01), timestamp(3682722366.259619 s since 1904-01-01), timestamp(3682722366.5631113 s since 1904-01-01), timestamp(3682722366.868568 s since 1904-01-01), timestamp(3682722367.202246 s since 1904-01-01), timestamp(3682722367.518932 s since 1904-01-01), timestamp(3682722367.835234 s since 1904-01-01), timestamp(3682722368.151437 s since 1904-01-01), timestamp(3682722368.455229 s since 1904-01-01), timestamp(3682722368.755842 s since 1904-01-01), timestamp(3682722369.070481 s since 1904-01-01), timestamp(3682722369.371531 s since 1904-01-01), timestamp(3682722369.674691 s since 1904-01-01), timestamp(3682722369.9750576 s since 1904-01-01), timestamp(3682722370.2769585 s since 1904-01-01), timestamp(3682722370.5767703 s since 1904-01-01), timestamp(3682722371.761378 s since 1904-01-01), timestamp(3682722372.0615153 s since 1904-01-01), timestamp(3682722372.36768 s since 1904-01-01), timestamp(3682722372.6716857 s since 1904-01-01), timestamp(3682722372.9741178 s since 1904-01-01), timestamp(3682722373.2752647 s since 1904-01-01), timestamp(3682722373.5791826 s since 1904-01-01), timestamp(3682722373.8855314 s since 1904-01-01), timestamp(3682722374.2075486 s since 1904-01-01), timestamp(3682722374.5190463 s since 1904-01-01), timestamp(3682722374.822685 s since 1904-01-01), timestamp(3682722375.135455 s since 1904-01-01), timestamp(3682722375.4391584 s since 1904-01-01), timestamp(3682722375.753536 s since 1904-01-01), timestamp(3682722376.0574703 s since 1904-01-01), timestamp(3682722376.3707743 s since 1904-01-01), timestamp(3682722376.671406 s since 1904-01-01), timestamp(3682722376.973929 s since 1904-01-01), timestamp(3682722377.275672 s since 1904-01-01), timestamp(3682722377.903696 s since 1904-01-01), timestamp(3682722378.3413343 s since 1904-01-01), timestamp(3682722378.6628866 s since 1904-01-01), timestamp(3682722378.971062 s since 1904-01-01), timestamp(3682722379.27123 s since 1904-01-01), timestamp(3682722379.574565 s since 1904-01-01), timestamp(3682722379.8750696 s since 1904-01-01), timestamp(3682722380.1758666 s since 1904-01-01), timestamp(3682722380.4776945 s since 1904-01-01), timestamp(3682722380.785676 s since 1904-01-01), timestamp(3682722381.101816 s since 1904-01-01), timestamp(3682722382.102351 s since 1904-01-01), timestamp(3682722383.1034727 s since 1904-01-01), timestamp(3682722384.102972 s since 1904-01-01), timestamp(3682722385.1037545 s since 1904-01-01), timestamp(3682722386.103784 s since 1904-01-01), timestamp(3682722387.1065063 s since 1904-01-01), timestamp(3682722388.105764 s since 1904-01-01), timestamp(3682722389.1080866 s since 1904-01-01), timestamp(3682722392.018273 s since 1904-01-01), timestamp(3682722393.0827537 s since 1904-01-01), timestamp(3682722394.4643016 s since 1904-01-01), timestamp(3682722395.4641614 s since 1904-01-01), timestamp(3682722396.465436 s since 1904-01-01), timestamp(3682722398.0099154 s since 1904-01-01), timestamp(3682722399.010983 s since 1904-01-01), timestamp(3682722400.0118704 s since 1904-01-01), timestamp(3682722401.013437 s since 1904-01-01), timestamp(3682722402.015486 s since 1904-01-01), timestamp(3682722403.0175056 s since 1904-01-01), timestamp(3682722404.01802 s since 1904-01-01), timestamp(3682722405.0194936 s since 1904-01-01), timestamp(3682722406.0196953 s since 1904-01-01), timestamp(3682722407.0214458 s since 1904-01-01), timestamp(3682722408.0222106 s since 1904-01-01), timestamp(3682722409.023329 s since 1904-01-01), timestamp(3682722410.0232754 s since 1904-01-01), timestamp(3682722411.024305 s since 1904-01-01), timestamp(3682722412.0254784 s since 1904-01-01), timestamp(3682722413.024827 s since 1904-01-01), timestamp(3682722414.026385 s since 1904-01-01), timestamp(3682722415.0269694 s since 1904-01-01), timestamp(3682722416.029292 s since 1904-01-01), timestamp(3682722417.03152 s since 1904-01-01), timestamp(3682722418.031929 s since 1904-01-01), timestamp(3682722419.03179 s since 1904-01-01), timestamp(3682722420.032112 s since 1904-01-01), timestamp(3682722421.0330806 s since 1904-01-01), timestamp(3682722422.032736 s since 1904-01-01), timestamp(3682722423.0335274 s since 1904-01-01), timestamp(3682722424.032856 s since 1904-01-01), timestamp(3682722425.0344257 s since 1904-01-01), timestamp(3682722426.0349946 s since 1904-01-01), timestamp(3682722427.1135817 s since 1904-01-01), timestamp(3682722428.113387 s since 1904-01-01), timestamp(3682722429.122927 s since 1904-01-01), timestamp(3682722430.122795 s since 1904-01-01), timestamp(3682722431.1243224 s since 1904-01-01), timestamp(3682722432.1657104 s since 1904-01-01), timestamp(3682722433.5395536 s since 1904-01-01), timestamp(3682722434.5393767 s since 1904-01-01), timestamp(3682722435.5397377 s since 1904-01-01), timestamp(3682722436.541572 s since 1904-01-01), timestamp(3682722437.8902345 s since 1904-01-01), timestamp(3682722438.889765 s since 1904-01-01), timestamp(3682722439.890742 s since 1904-01-01), timestamp(3682722440.8925166 s since 1904-01-01), timestamp(3682722441.8928022 s since 1904-01-01), timestamp(3682722442.8935113 s since 1904-01-01), timestamp(3682722443.9465127 s since 1904-01-01), timestamp(3682722444.946664 s since 1904-01-01), timestamp(3682722445.946266 s since 1904-01-01), timestamp(3682722446.945718 s since 1904-01-01), timestamp(3682722447.9487176 s since 1904-01-01), timestamp(3682722448.9498606 s since 1904-01-01), timestamp(3682722449.9507394 s since 1904-01-01), timestamp(3682722451.010164 s since 1904-01-01), timestamp(3682722452.011107 s since 1904-01-01), timestamp(3682722453.0121975 s since 1904-01-01), timestamp(3682722454.013758 s since 1904-01-01), timestamp(3682722455.129564 s since 1904-01-01), timestamp(3682722456.129246 s since 1904-01-01), timestamp(3682722457.1289473 s since 1904-01-01), timestamp(3682722458.129476 s since 1904-01-01), timestamp(3682722459.129673 s since 1904-01-01), timestamp(3682722460.1309032 s since 1904-01-01), timestamp(3682722461.1332126 s since 1904-01-01), timestamp(3682722462.133421 s since 1904-01-01), timestamp(3682722463.1336327 s since 1904-01-01), timestamp(3682722464.1343303 s since 1904-01-01), timestamp(3682722465.134672 s since 1904-01-01), timestamp(3682722466.135208 s since 1904-01-01), timestamp(3682722467.1370697 s since 1904-01-01), timestamp(3682722468.136828 s since 1904-01-01), timestamp(3682722469.4057984 s since 1904-01-01)]
  out "TimeArray Size (336)":i32=332
  out "DataArray (336)":dbl[][](array[numeric])=[[95.4144, 95.2813, 133.127, 132.564, 138.25, 138.265, 138.199, 137.404], [95.4109, 95.2811, 133.125, 132.563, 138.248, 138.266, 138.2, 137.404], [95.4076, 95.2812, 133.127, 132.562, 138.246, 138.27, 138.2, 137.405], [95.4145, 95.2793, 133.129, 132.562, 138.25, 138.269, 138.198, 137.41], [95.4132, 95.281, 133.127, 132.563, 138.251, 138.27, 138.2, 137.405], [95.4164, 95.2745, 133.13, 132.564, 138.25, 138.267, 138.2, 137.404], [95.4172, 95.2793, 133.128, 132.563, 138.25, 138.267, 138.2, 137.406], [95.409, 95.2842, 133.128, 132.562, 138.245, 138.267, 138.204, 137.403], [95.4051, 95.2815, 133.131, 132.564, 138.248, 138.265, 138.201, 137.408], [95.4033, 95.2922, 133.129, 132.567, 138.247, 138.267, 138.2, 137.406], [95.4199, 95.2891, 133.129, 132.563, 138.254, 138.269, 138.2, 137.404], [95.41, 95.2827, 133.129, 132.561, 138.249, 138.268, 138.201, 137.41], [95.407, 95.276, 133.126, 132.564, 138.25, 138.269, 138.203, 137.409], [95.4152, 95.3249, 133.135, 132.564, 138.253, 138.266, 138.2, 137.406], [95.4102, 95.2723, 133.129, 132.563, 138.255, 138.271, 138.203, 137.407], [95.4213, 95.2806, 133.129, 132.565, 138.252, 138.269, 138.201, 137.411], [95.4119, 95.2804, 133.13, 132.56, 138.249, 138.269, 138.201, 137.409], [95.4069, 95.2767, 133.133, 132.563, 138.254, 138.27, 138.201, 137.41], [95.4094, 95.2781, 133.131, 132.565, 138.253, 138.269, 138.197, 137.407], [95.4119, 95.2776, 133.13, 132.562, 138.252, 138.269, 138.203, 137.407], [95.4095, 95.286, 133.13, 132.561, 138.251, 138.267, 138.204, 137.408], [95.3896, 95.2819, 133.134, 132.563, 138.25, 138.268, 138.2, 137.405], [95.4084, 95.2768, 133.134, 132.562, 138.247, 138.27, 138.206, 137.409], [95.408, 95.2856, 133.133, 132.563, 138.252, 138.27, 138.209, 137.406], [95.4139, 95.2746, 133.131, 132.563, 138.251, 138.271, 138.208, 137.405], [95.4132, 95.2838, 133.132, 132.564, 138.252, 138.266, 138.202, 137.405], [95.4122, 95.2779, 133.135, 132.561, 138.251, 138.271, 138.206, 137.411], [95.4127, 95.2784, 133.136, 132.562, 138.251, 138.268, 138.202, 137.408], [95.4119, 95.278, 133.135, 132.561, 138.252, 138.271, 138.204, 137.41], [95.4203, 95.2805, 133.136, 132.564, 138.254, 138.27, 138.205, 137.407], [95.4187, 95.2776, 133.137, 132.564, 138.251, 138.266, 138.205, 137.409], [95.42, 95.278, 133.13, 132.564, 138.253, 138.268, 138.203, 137.41], [95.4224, 95.2807, 133.134, 132.566, 138.253, 138.27, 138.204, 137.41], [95.4188, 95.2811, 133.133, 132.561, 138.253, 138.27, 138.205, 137.408], [95.4205, 95.2853, 133.134, 132.562, 138.251, 138.27, 138.203, 137.41], [95.4169, 95.2851, 133.137, 132.562, 138.249, 138.274, 138.206, 137.41], [95.4224, 95.2786, 133.135, 132.561, 138.252, 138.273, 138.205, 137.408], [95.4242, 95.2812, 133.136, 132.562, 138.252, 138.27, 138.202, 137.409], [95.4139, 95.2822, 133.134, 132.559, 138.256, 138.273, 138.204, 137.409], [95.4156, 95.2813, 133.139, 132.562, 138.253, 138.271, 138.207, 137.411], [95.4133, 95.2839, 133.136, 132.563, 138.252, 138.271, 138.204, 137.409], [95.4122, 95.2751, 133.136, 132.562, 138.251, 138.272, 138.202, 137.411], [95.4071, 95.2803, 133.136, 132.561, 138.253, 138.271, 138.206, 137.409], [95.4138, 95.2802, 133.137, 132.564, 138.253, 138.269, 138.206, 137.413], [95.4084, 95.2771, 133.136, 132.564, 138.254, 138.273, 138.208, 137.407], [95.4123, 95.2859, 133.135, 132.565, 138.255, 138.272, 138.205, 137.409], [95.417, 95.2802, 133.136, 132.561, 138.254, 138.273, 138.201, 137.409], [95.4119, 95.2826, 133.137, 132.56, 138.252, 138.274, 138.208, 137.41], [95.4071, 95.2779, 133.138, 132.563, 138.258, 138.274, 138.209, 137.408], [95.4116, 95.2839, 133.137, 132.564, 138.252, 138.271, 138.201, 137.408], [95.412, 95.2797, 133.138, 132.561, 138.253, 138.272, 138.206, 137.408], [95.412, 95.2785, 133.139, 132.563, 138.256, 138.269, 138.209, 137.409], [95.4152, 95.2835, 133.139, 132.564, 138.259, 138.268, 138.206, 137.409], [95.4095, 95.2815, 133.136, 132.563, 138.258, 138.275, 138.206, 137.41], [95.4111, 95.2798, 133.138, 132.563, 138.254, 138.27, 138.208, 137.412], [95.4126, 95.2839, 133.137, 132.563, 138.255, 138.275, 138.206, 137.409], [95.4105, 95.2776, 133.139, 132.562, 138.254, 138.272, 138.206, 137.41], [95.3709, 95.2535, 133.136, 132.56, 138.254, 138.274, 138.205, 137.41], [95.4121, 95.2821, 133.139, 132.561, 138.254, 138.274, 138.206, 137.411], [95.415, 95.2848, 133.138, 132.562, 138.254, 138.274, 138.204, 137.408], [95.4125, 95.2797, 133.139, 132.563, 138.254, 138.276, 138.204, 137.412], [95.4139, 95.2859, 133.139, 132.561, 138.258, 138.272, 138.21, 137.409], [95.4159, 95.2851, 133.138, 132.564, 138.253, 138.273, 138.206, 137.412], [95.4184, 95.2834, 133.141, 132.561, 138.252, 138.275, 138.207, 137.413], [95.4154, 95.2858, 133.141, 132.562, 138.256, 138.271, 138.206, 137.411], [95.4131, 95.2859, 133.138, 132.561, 138.256, 138.275, 138.209, 137.412], [95.4175, 95.2783, 133.139, 132.563, 138.257, 138.271, 138.207, 137.411], [95.4077, 95.2772, 133.142, 132.564, 138.252, 138.273, 138.205, 137.41], [95.409, 95.2846, 133.14, 132.561, 138.258, 138.273, 138.206, 137.412], [95.4164, 95.2766, 133.14, 132.565, 138.257, 138.272, 138.204, 137.41], [95.4132, 95.276, 133.138, 132.563, 138.253, 138.274, 138.206, 137.413], [95.4108, 95.2832, 133.142, 132.564, 138.255, 138.275, 138.21, 137.412], [95.4151, 95.2841, 133.139, 132.562, 138.256, 138.276, 138.21, 137.414], [95.4095, 95.2829, 133.14, 132.563, 138.254, 138.273, 138.203, 137.41], [95.403, 95.2785, 133.141, 132.563, 138.257, 138.275, 138.208, 137.409], [95.4123, 95.2846, 133.139, 132.562, 138.255, 138.273, 138.209, 137.41], [95.4167, 95.278, 133.142, 132.56, 138.257, 138.273, 138.204, 137.412], [95.4135, 95.2772, 133.143, 132.562, 138.254, 138.275, 138.207, 137.411], [95.4304, 95.2932, 133.144, 132.565, 138.255, 138.277, 138.206, 137.411], [95.4174, 95.2783, 133.142, 132.564, 138.26, 138.274, 138.208, 137.41], [95.4144, 95.2881, 133.141, 132.559, 138.258, 138.275, 138.209, 137.412], [95.416, 95.2812, 133.144, 132.566, 138.255, 138.277, 138.206, 137.416], [95.4086, 95.2784, 133.137, 132.56, 138.254, 138.275, 138.209, 137.412], [95.4106, 95.2832, 133.144, 132.563, 138.259, 138.274, 138.209, 137.415], [95.4191, 95.278, 133.141, 132.56, 138.257, 138.275, 138.207, 137.417], [95.4118, 95.2736, 133.141, 132.562, 138.257, 138.275, 138.206, 137.411], [95.4197, 95.2823, 133.144, 132.562, 138.255, 138.278, 138.209, 137.411], [95.4161, 95.277, 133.144, 132.56, 138.255, 138.277, 138.206, 137.415], [95.4089, 95.2743, 133.142, 132.566, 138.262, 138.27, 138.21, 137.419], [95.4073, 95.2783, 133.142, 132.564, 138.26, 138.276, 138.207, 137.415], [95.404, 95.2773, 133.141, 132.561, 138.256, 138.277, 138.21, 137.414], [95.4122, 95.2824, 133.143, 132.567, 138.259, 138.277, 138.209, 137.412], [95.4112, 95.2752, 133.141, 132.562, 138.258, 138.279, 138.209, 137.411], [95.4032, 95.2748, 133.143, 132.562, 138.258, 138.275, 138.208, 137.415], [95.4121, 95.2787, 133.143, 132.564, 138.255, 138.273, 138.21, 137.414], [95.4064, 95.2775, 133.144, 132.564, 138.257, 138.277, 138.212, 137.414], [95.4131, 95.2764, 133.144, 132.563, 138.258, 138.276, 138.211, 137.417], [95.4181, 95.2797, 133.141, 132.565, 138.259, 138.274, 138.209, 137.414], [95.4117, 95.2816, 133.142, 132.562, 138.261, 138.276, 138.208, 137.413], [95.4108, 95.2779, 133.143, 132.562, 138.256, 138.275, 138.211, 137.414], [95.4131, 95.277, 133.144, 132.563, 138.255, 138.277, 138.208, 137.414], [95.4095, 95.2758, 133.142, 132.563, 138.259, 138.276, 138.21, 137.412], [95.4145, 95.2801, 133.144, 132.561, 138.258, 138.28, 138.21, 137.413], [95.4154, 95.2821, 133.142, 132.562, 138.256, 138.276, 138.209, 137.412], [95.4113, 95.2804, 133.143, 132.561, 138.26, 138.277, 138.212, 137.416], [95.4129, 95.282, 133.148, 132.563, 138.254, 138.274, 138.21, 137.411], [95.4051, 95.2738, 133.143, 132.562, 138.257, 138.275, 138.207, 137.414], [95.4134, 95.286, 133.145, 132.564, 138.259, 138.276, 138.213, 137.414], [95.4139, 95.2798, 133.144, 132.558, 138.259, 138.277, 138.211, 137.413], [95.4106, 95.2788, 133.144, 132.56, 138.259, 138.275, 138.208, 137.415], [95.4106, 95.2793, 133.144, 132.56, 138.259, 138.277, 138.21, 137.418], [95.4092, 95.2785, 133.145, 132.562, 138.261, 138.274, 138.209, 137.415], [95.4104, 95.2775, 133.147, 132.564, 138.251, 138.273, 138.207, 137.418], [95.4143, 95.2841, 133.144, 132.562, 138.26, 138.277, 138.21, 137.41], [95.4123, 95.2859, 133.146, 132.563, 138.26, 138.278, 138.209, 137.412], [95.4123, 95.2796, 133.146, 132.565, 138.255, 138.274, 138.207, 137.416], [95.4154, 95.2812, 133.144, 132.562, 138.261, 138.276, 138.209, 137.414], [95.4102, 95.2888, 133.146, 132.564, 138.257, 138.276, 138.211, 137.418], [95.4083, 95.2844, 133.145, 132.562, 138.261, 138.28, 138.211, 137.415], [95.4133, 95.2793, 133.146, 132.562, 138.26, 138.272, 138.208, 137.415], [95.409, 95.2808, 133.146, 132.561, 138.258, 138.278, 138.209, 137.415], [95.4035, 95.2794, 133.146, 132.563, 138.259, 138.275, 138.211, 137.415], [95.4137, 95.2786, 133.145, 132.565, 138.259, 138.278, 138.209, 137.418], [95.4188, 95.2801, 133.146, 132.562, 138.255, 138.278, 138.212, 137.415], [95.4061, 95.2817, 133.146, 132.56, 138.257, 138.279, 138.213, 137.417], [95.4074, 95.2812, 133.149, 132.563, 138.258, 138.28, 138.211, 137.415], [95.4348, 95.2977, 133.148, 132.564, 138.261, 138.277, 138.211, 137.412], [95.4183, 95.2812, 133.146, 132.563, 138.26, 138.277, 138.21, 137.413], [95.4089, 95.2817, 133.146, 132.564, 138.26, 138.277, 138.212, 137.419], [95.4126, 95.2817, 133.149, 132.564, 138.259, 138.281, 138.212, 137.416], [95.4132, 95.2803, 133.146, 132.559, 138.26, 138.277, 138.211, 137.414], [95.4084, 95.2835, 133.148, 132.558, 138.261, 138.278, 138.212, 137.418], [95.413, 95.281, 133.144, 132.563, 138.26, 138.278, 138.21, 137.414], [95.4106, 95.2811, 133.145, 132.562, 138.259, 138.28, 138.211, 137.415], [95.4091, 95.2821, 133.146, 132.563, 138.26, 138.279, 138.215, 137.417], [95.4102, 95.286, 133.149, 132.563, 138.259, 138.28, 138.214, 137.414], [95.4087, 95.2831, 133.147, 132.563, 138.261, 138.277, 138.216, 137.418], [95.476, 95.3333, 133.151, 132.561, 138.261, 138.278, 138.212, 137.419], [95.4078, 95.2834, 133.148, 132.562, 138.261, 138.277, 138.213, 137.415], [95.4058, 95.2799, 133.148, 132.564, 138.259, 138.277, 138.212, 137.419], [95.4029, 95.2781, 133.147, 132.563, 138.259, 138.278, 138.216, 137.415], [95.4142, 95.2813, 133.15, 132.564, 138.262, 138.277, 138.212, 137.417], [95.4134, 95.278, 133.148, 132.561, 138.26, 138.279, 138.212, 137.416], [95.415, 95.2865, 133.149, 132.565, 138.259, 138.279, 138.209, 137.413], [95.4107, 95.2773, 133.147, 132.561, 138.263, 138.277, 138.214, 137.417], [95.4157, 95.281, 133.148, 132.562, 138.262, 138.277, 138.212, 137.418], [95.4027, 95.2788, 133.152, 132.561, 138.262, 138.279, 138.216, 137.418], [95.41, 95.2789, 133.149, 132.56, 138.262, 138.278, 138.214, 137.417], [95.4088, 95.2841, 133.149, 132.561, 138.259, 138.278, 138.213, 137.419], [95.4111, 95.2799, 133.15, 132.559, 138.262, 138.279, 138.211, 137.419], [95.4093, 95.2808, 133.15, 132.563, 138.263, 138.278, 138.211, 137.417], [95.4097, 95.2774, 133.148, 132.561, 138.262, 138.282, 138.214, 137.417], [95.4076, 95.2807, 133.15, 132.563, 138.265, 138.282, 138.219, 137.42], [95.408, 95.2832, 133.151, 132.563, 138.26, 138.277, 138.212, 137.417], [95.4072, 95.2746, 133.149, 132.563, 138.259, 138.282, 138.218, 137.42], [95.4108, 95.2793, 133.15, 132.561, 138.261, 138.283, 138.213, 137.417], [95.4139, 95.2847, 133.149, 132.558, 138.262, 138.279, 138.211, 137.414], [95.4084, 95.2723, 133.151, 132.562, 138.269, 138.283, 138.216, 137.419], [95.4072, 95.2817, 133.151, 132.564, 138.26, 138.281, 138.213, 137.419], [95.4118, 95.2855, 133.149, 132.562, 138.263, 138.279, 138.214, 137.416], [95.4041, 95.2834, 133.152, 132.561, 138.262, 138.277, 138.213, 137.418], [95.4159, 95.2824, 133.151, 132.561, 138.26, 138.282, 138.211, 137.417], [95.4101, 95.2807, 133.147, 132.563, 138.258, 138.28, 138.213, 137.42], [95.4076, 95.2745, 133.152, 132.564, 138.261, 138.28, 138.215, 137.422], [95.4052, 95.2784, 133.151, 132.563, 138.262, 138.281, 138.216, 137.42], [95.4106, 95.2765, 133.152, 132.562, 138.263, 138.277, 138.214, 137.418], [95.4141, 95.2796, 133.151, 132.563, 138.261, 138.279, 138.216, 137.419], [95.409, 95.28, 133.152, 132.562, 138.264, 138.278, 138.216, 137.422], [95.4123, 95.2839, 133.152, 132.562, 138.263, 138.278, 138.212, 137.416], [95.4091, 95.2837, 133.152, 132.559, 138.261, 138.283, 138.216, 137.418], [95.3819, 95.2646, 133.154, 132.562, 138.263, 138.28, 138.216, 137.417], [95.4031, 95.2843, 133.152, 132.559, 138.262, 138.283, 138.217, 137.422], [95.4038, 95.28, 133.153, 132.563, 138.262, 138.278, 138.214, 137.421], [95.4002, 95.2875, 133.151, 132.561, 138.263, 138.283, 138.213, 137.418], [95.4054, 95.2837, 133.153, 132.562, 138.262, 138.28, 138.213, 137.418], [95.4103, 95.2783, 133.155, 132.562, 138.265, 138.281, 138.216, 137.419], [95.4095, 95.2841, 133.153, 132.564, 138.261, 138.28, 138.215, 137.421], [95.4047, 95.2817, 133.155, 132.561, 138.265, 138.282, 138.217, 137.422], [95.4058, 95.2802, 133.152, 132.563, 138.264, 138.282, 138.211, 137.417], [95.4078, 95.281, 133.153, 132.565, 138.263, 138.283, 138.215, 137.418], [95.409, 95.2848, 133.153, 132.564, 138.264, 138.279, 138.215, 137.421], [95.4145, 95.2808, 133.152, 132.559, 138.263, 138.28, 138.216, 137.419], [95.4414, 95.3032, 133.158, 132.565, 138.264, 138.281, 138.213, 137.421], [95.4089, 95.2812, 133.156, 132.559, 138.262, 138.28, 138.216, 137.42], [95.418, 95.2799, 133.154, 132.565, 138.264, 138.282, 138.214, 137.417], [95.414, 95.2843, 133.153, 132.56, 138.268, 138.283, 138.214, 137.422], [95.4041, 95.2803, 133.153, 132.561, 138.261, 138.282, 138.216, 137.415], [95.4157, 95.2851, 133.156, 132.562, 138.26, 138.279, 138.214, 137.42], [95.4179, 95.2812, 133.155, 132.562, 138.265, 138.283, 138.217, 137.42], [95.4149, 95.2875, 133.154, 132.56, 138.258, 138.279, 138.213, 137.418], [95.4062, 95.2806, 133.154, 132.561, 138.264, 138.282, 138.214, 137.426], [95.4201, 95.28, 133.155, 132.561, 138.263, 138.286, 138.217, 137.423], [95.4123, 95.2746, 133.152, 132.561, 138.265, 138.285, 138.216, 137.423], [95.4148, 95.2802, 133.158, 132.562, 138.268, 138.28, 138.213, 137.419], [95.419, 95.28, 133.157, 132.561, 138.265, 138.285, 138.218, 137.422], [95.4105, 95.282, 133.157, 132.563, 138.266, 138.284, 138.219, 137.425], [95.4153, 95.2829, 133.153, 132.563, 138.265, 138.283, 138.219, 137.423], [95.4217, 95.277, 133.155, 132.562, 138.264, 138.282, 138.218, 137.422], [95.4076, 95.2861, 133.153, 132.561, 138.266, 138.285, 138.214, 137.424], [95.4176, 95.2798, 133.155, 132.561, 138.266, 138.284, 138.215, 137.417], [95.4105, 95.2802, 133.155, 132.561, 138.266, 138.285, 138.219, 137.421], [95.412, 95.2866, 133.156, 132.563, 138.265, 138.284, 138.216, 137.421], [95.4148, 95.2791, 133.157, 132.564, 138.264, 138.282, 138.217, 137.423], [95.4131, 95.2849, 133.156, 132.56, 138.264, 138.285, 138.215, 137.421], [95.4173, 95.2812, 133.157, 132.564, 138.266, 138.28, 138.216, 137.424], [95.4116, 95.2746, 133.157, 132.56, 138.264, 138.285, 138.217, 137.422], [95.4152, 95.276, 133.158, 132.565, 138.267, 138.286, 138.215, 137.422], [95.4153, 95.2887, 133.156, 132.559, 138.266, 138.285, 138.219, 137.423], [95.4161, 95.2775, 133.155, 132.564, 138.268, 138.282, 138.217, 137.423], [95.4145, 95.2822, 133.158, 132.563, 138.267, 138.281, 138.217, 137.421], [95.4062, 95.2877, 133.158, 132.561, 138.265, 138.281, 138.217, 137.427], [95.4758, 95.2802, 133.158, 132.56, 138.268, 138.285, 138.222, 137.423], [95.4041, 95.2875, 133.158, 132.561, 138.268, 138.284, 138.222, 137.422], [95.4127, 95.2815, 133.159, 132.561, 138.268, 138.285, 138.217, 137.421], [95.4215, 95.2842, 133.155, 132.559, 138.265, 138.284, 138.217, 137.428], [95.4118, 95.2831, 133.161, 132.561, 138.269, 138.285, 138.22, 137.424], [95.4197, 95.2883, 133.162, 132.564, 138.267, 138.282, 138.218, 137.42], [95.4164, 95.2817, 133.159, 132.559, 138.268, 138.286, 138.217, 137.425], [95.4205, 95.286, 133.159, 132.562, 138.27, 138.285, 138.218, 137.423], [95.4183, 95.3004, 133.16, 132.56, 138.267, 138.288, 138.216, 137.421], [95.4347, 95.2837, 133.158, 132.566, 138.261, 138.285, 138.217, 137.421], [95.4137, 95.285, 133.156, 132.566, 138.265, 138.285, 138.219, 137.422], [95.4217, 95.2827, 133.159, 132.561, 138.27, 138.284, 138.22, 137.423], [95.424, 95.2843, 133.159, 132.561, 138.267, 138.281, 138.219, 137.423], [95.4157, 95.2855, 133.161, 132.564, 138.266, 138.288, 138.217, 137.424], [95.4118, 95.2813, 133.159, 132.562, 138.266, 138.283, 138.215, 137.422], [95.4207, 95.2844, 133.157, 132.559, 138.269, 138.287, 138.221, 137.424], [95.4134, 95.2811, 133.159, 132.561, 138.269, 138.288, 138.217, 137.423], [95.4168, 95.2883, 133.16, 132.565, 138.268, 138.283, 138.22, 137.424], [95.413, 95.2793, 133.158, 132.559, 138.268, 138.287, 138.223, 137.427], [95.4213, 95.2825, 133.16, 132.561, 138.266, 138.287, 138.217, 137.424], [95.4213, 95.2793, 133.157, 132.56, 138.267, 138.284, 138.218, 137.424], [95.42, 95.2822, 133.158, 132.562, 138.266, 138.283, 138.218, 137.424], [95.4166, 95.2856, 133.159, 132.562, 138.269, 138.284, 138.215, 137.425], [95.412, 95.2892, 133.161, 132.563, 138.266, 138.286, 138.219, 137.421], [95.4091, 95.2869, 133.162, 132.563, 138.269, 138.287, 138.226, 137.427], [95.4156, 95.2851, 133.16, 132.561, 138.268, 138.285, 138.221, 137.426], [95.4182, 95.2783, 133.163, 132.562, 138.269, 138.285, 138.218, 137.423], [95.4189, 95.2821, 133.162, 132.563, 138.267, 138.284, 138.221, 137.423], [95.4179, 95.2814, 133.159, 132.559, 138.267, 138.284, 138.219, 137.423], [95.4178, 95.2813, 133.16, 132.564, 138.268, 138.291, 138.222, 137.427], [95.4181, 95.2864, 133.163, 132.564, 138.266, 138.283, 138.222, 137.425], [95.4176, 95.2329, 133.154, 132.561, 138.271, 138.285, 138.22, 137.426], [95.4104, 95.2826, 133.161, 132.561, 138.269, 138.286, 138.221, 137.426], [95.4149, 95.2786, 133.161, 132.561, 138.27, 138.286, 138.221, 137.424], [95.4224, 95.2831, 133.162, 132.56, 138.269, 138.286, 138.219, 137.424], [95.413, 95.2853, 133.162, 132.56, 138.27, 138.287, 138.221, 137.423], [95.4207, 95.2784, 133.162, 132.56, 138.27, 138.283, 138.221, 137.428], [95.4141, 95.2841, 133.16, 132.561, 138.271, 138.284, 138.221, 137.423], [95.4165, 95.2876, 133.16, 132.558, 138.268, 138.287, 138.222, 137.423], [95.4161, 95.2832, 133.159, 132.56, 138.271, 138.288, 138.218, 137.426], [95.4132, 95.2849, 133.164, 132.563, 138.269, 138.286, 138.221, 137.425], [95.4222, 95.2868, 133.162, 132.563, 138.27, 138.287, 138.222, 137.428], [95.4713, 95.3352, 133.163, 132.561, 138.269, 138.291, 138.223, 137.428], [95.4147, 95.2884, 133.165, 132.564, 138.271, 138.286, 138.222, 137.43], [95.418, 95.2822, 133.166, 132.562, 138.27, 138.289, 138.223, 137.428], [95.4252, 95.2907, 133.163, 132.56, 138.271, 138.288, 138.223, 137.426], [95.4181, 95.2803, 133.165, 132.56, 138.269, 138.29, 138.221, 137.426], [95.4133, 95.2751, 133.167, 132.561, 138.277, 138.292, 138.224, 137.429], [95.4152, 95.2832, 133.167, 132.561, 138.276, 138.29, 138.225, 137.428], [95.4154, 95.2889, 133.166, 132.558, 138.272, 138.29, 138.227, 137.429], [95.423, 95.2805, 133.169, 132.561, 138.27, 138.288, 138.227, 137.429], [95.4198, 95.2837, 133.167, 132.561, 138.273, 138.291, 138.223, 137.432], [95.4192, 95.2837, 133.168, 132.559, 138.27, 138.292, 138.225, 137.429], [95.4125, 95.2857, 133.167, 132.557, 138.271, 138.29, 138.226, 137.428], [95.4187, 95.2858, 133.168, 132.561, 138.275, 138.29, 138.226, 137.431], [95.4136, 95.2837, 133.167, 132.556, 138.273, 138.29, 138.226, 137.43], [95.4069, 95.2879, 133.171, 132.558, 138.271, 138.292, 138.225, 137.432], [95.4065, 95.2831, 133.169, 132.562, 138.275, 138.294, 138.228, 137.435], [95.4132, 95.2851, 133.168, 132.56, 138.274, 138.291, 138.23, 137.43], [95.4102, 95.2831, 133.168, 132.558, 138.273, 138.291, 138.224, 137.431], [95.4159, 95.2881, 133.171, 132.559, 138.276, 138.295, 138.228, 137.434], [95.4179, 95.292, 133.171, 132.56, 138.277, 138.295, 138.226, 137.434], [95.4147, 95.2959, 133.17, 132.557, 138.272, 138.292, 138.229, 137.434], [95.407, 95.29, 133.173, 132.56, 138.276, 138.293, 138.228, 137.431], [95.4152, 95.2916, 133.171, 132.558, 138.277, 138.292, 138.227, 137.428], [95.4116, 95.2896, 133.174, 132.559, 138.277, 138.291, 138.23, 137.432], [95.4141, 95.2897, 133.173, 132.561, 138.276, 138.296, 138.227, 137.432], [95.4168, 95.2942, 133.172, 132.561, 138.277, 138.299, 138.232, 137.44], [95.4136, 95.2918, 133.172, 132.559, 138.276, 138.293, 138.226, 137.437], [95.468, 95.3268, 133.175, 132.56, 138.279, 138.297, 138.229, 137.435], [95.4195, 95.2909, 133.174, 132.56, 138.277, 138.293, 138.226, 137.433], [95.4111, 95.2881, 133.174, 132.561, 138.278, 138.297, 138.228, 137.437], [95.411, 95.2924, 133.176, 132.56, 138.28, 138.296, 138.234, 137.433], [95.4142, 95.2927, 133.176, 132.562, 138.277, 138.293, 138.225, 137.439], [95.4139, 95.2907, 133.173, 132.558, 138.277, 138.297, 138.229, 137.436], [95.4076, 95.2855, 133.176, 132.556, 138.277, 138.294, 138.226, 137.435], [95.4136, 95.2868, 133.175, 132.558, 138.279, 138.296, 138.232, 137.435], [95.408, 95.281, 133.176, 132.559, 138.28, 138.295, 138.228, 137.437], [95.41, 95.2812, 133.176, 132.563, 138.28, 138.297, 138.231, 137.436], [95.4082, 95.2866, 133.177, 132.561, 138.279, 138.297, 138.231, 137.437], [95.4046, 95.2778, 133.18, 132.556, 138.278, 138.296, 138.233, 137.437], [95.4106, 95.2826, 133.178, 132.559, 138.28, 138.295, 138.231, 137.436], [95.411, 95.2918, 133.177, 132.555, 138.281, 138.3, 138.228, 137.435], [95.4137, 95.2868, 133.176, 132.56, 138.282, 138.298, 138.23, 137.437], [95.4137, 95.2894, 133.179, 132.558, 138.278, 138.296, 138.228, 137.439], [95.4027, 95.2826, 133.177, 132.558, 138.28, 138.298, 138.232, 137.439], [95.4071, 95.2808, 133.178, 132.559, 138.282, 138.302, 138.232, 137.439], [95.3555, 95.2463, 133.176, 132.562, 138.275, 138.297, 138.234, 137.438], [95.4143, 95.2851, 133.18, 132.56, 138.28, 138.3, 138.232, 137.439], [95.4117, 95.2887, 133.182, 132.559, 138.281, 138.298, 138.234, 137.438], [95.4094, 95.2852, 133.181, 132.56, 138.282, 138.303, 138.236, 137.44], [95.413, 95.2809, 133.184, 132.561, 138.28, 138.3, 138.233, 137.441], [95.4166, 95.2841, 133.181, 132.558, 138.283, 138.302, 138.235, 137.441], [95.4111, 95.2831, 133.182, 132.562, 138.282, 138.302, 138.233, 137.44], [95.418, 95.2849, 133.18, 132.558, 138.281, 138.302, 138.234, 137.439], [95.4135, 95.2808, 133.182, 132.561, 138.284, 138.301, 138.235, 137.438], [95.4138, 95.286, 133.184, 132.56, 138.281, 138.299, 138.232, 137.44], [95.4219, 95.2888, 133.182, 132.56, 138.283, 138.302, 138.238, 137.439], [95.4228, 95.2871, 133.185, 132.559, 138.288, 138.303, 138.239, 137.443], [95.4158, 95.2867, 133.186, 132.563, 138.282, 138.302, 138.232, 137.44], [95.4153, 95.2851, 133.183, 132.558, 138.282, 138.301, 138.234, 137.441], [95.422, 95.2831, 133.185, 132.56, 138.283, 138.302, 138.234, 137.441], [95.4258, 95.2894, 133.183, 132.558, 138.287, 138.301, 138.234, 137.44], [95.4288, 95.2884, 133.185, 132.56, 138.284, 138.3, 138.237, 137.439], [95.4252, 95.2861, 133.186, 132.558, 138.285, 138.302, 138.237, 137.438], [95.3894, 95.2627, 133.183, 132.558, 138.287, 138.299, 138.235, 137.441], [95.4222, 95.2821, 133.187, 132.557, 138.285, 138.305, 138.239, 137.439], [95.4242, 95.2894, 133.187, 132.557, 138.285, 138.304, 138.236, 137.446], [95.4223, 95.2874, 133.188, 132.557, 138.288, 138.307, 138.239, 137.442], [95.4214, 95.2899, 133.187, 132.559, 138.288, 138.308, 138.238, 137.444], [95.4224, 95.2877, 133.186, 132.56, 138.288, 138.305, 138.237, 137.442], [95.4149, 95.2901, 133.185, 132.559, 138.288, 138.307, 138.239, 137.447], [95.4159, 95.2857, 133.186, 132.559, 138.288, 138.305, 138.24, 137.443], [95.4183, 95.2852, 133.186, 132.557, 138.286, 138.304, 138.24, 137.448], [95.42, 95.2845, 133.19, 132.558, 138.289, 138.304, 138.24, 137.447], [95.4171, 95.2912, 133.189, 132.559, 138.286, 138.306, 138.244, 137.444], [95.4214, 95.2937, 133.189, 132.559, 138.286, 138.307, 138.237, 137.442], [95.4156, 95.2903, 133.187, 132.557, 138.288, 138.31, 138.239, 137.443], [95.4276, 95.2906, 133.19, 132.56, 138.289, 138.305, 138.238, 137.447], [95.4208, 95.288, 133.191, 132.559, 138.289, 138.305, 138.238, 137.447], [95.4242, 95.2873, 133.19, 132.559, 138.289, 138.31, 138.239, 137.444]]
  out "DataArray size (336)":i32[](array[numeric])=[332, 8]
  out "LastData (LSI218)":dbl[](array[numeric])=[285.45, 290.71, 245.43, 252.59, 172.54, 177.97, 71.656, 129.11, 30.0, 0.0, 0.0, 0.0, 207.67, 199.47, 131.72, 290.16, 292.6, 292.74, 292.31, 292.37, 207.68, 204.03, 195.11, 188.36, 194.01, 235.91, 290.83, 290.58, 249.16, 274.59, 270.4, 284.47, 279.27, 0.0, 231.46, 688.49, 199.72, 114.83, 153.45, 688.58, 126.48, 94.139, 102.89, 143.16, 127.49, 149.95, 0.433, 0.0]
  out "TempSensorsLocations":T12(array[ring])=[enum."T3He10", enum."T3He1-1", enum."TTH3", enum."TTH4", enum."TTH1", enum."TTH2", enum."T4He1", enum."T1K1", enum."N.C.", enum."N.C.", enum."N.C.", enum."T3He1-4", enum."T3He2-1", enum."T3He2-2", enum."T3He3", enum."T3He1-4", enum."T4He3-1", enum."T4He3-2", enum."T4He3-3", enum."T4He3-4", enum."T4He2-1", enum."T4He2-2", enum."T4He4", enum."T4He5", enum."T4He6", enum."T4He9", enum."T3He1-2", enum."T3He1-3", enum."T4He7", enum."T4He8", enum."T4He10", enum."T1K6", enum."TIP1", enum."N.C.", enum."TIP2", enum."N.C.", enum."TIP3", enum."TIP4", enum."TIP5", enum."N.C.", enum."T1K2", enum."T1K4", enum."T1K5", enum."T3He4", enum."T3He9", enum."TIP6", enum."N.C.", enum."N.C.", enum."T1K3-1", enum."T1K3-2", enum."T3He5", enum."T3He8", enum."T3He6-1", enum."T3He6-2", enum."T3He7-1", enum."T3He7-2"]
  out "AllTemperatures":dbl[](array[numeric])=[285.44, 290.7, 245.42, 252.6, 172.52, 177.97, 71.656, 129.11, 30.0, 0.0, 0.0, 0.0, 207.67, 199.47, 131.72, 290.15, 292.61, 292.75, 292.31, 292.38, 207.68, 204.02, 195.1, 188.35, 194.05, 235.88, 290.84, 290.57, 249.16, 274.6, 270.39, 284.49, 279.27, 0.0, 231.46, 688.49, 199.72, 114.84, 153.46, 688.58, 126.48, 93.845, 102.91, 143.19, 128.03, 149.97, 0.433, 0.0, 95.4208, 95.288, 133.191, 132.559, 138.289, 138.305, 138.238, 137.447]
  out "error out (frontpanel screenshots)":errorcluster
  # "GLOBAL STATUS/CONTROL"
  # "Global Settings"
  # "USB6210 Analog inputs Settings"
  # "USB6218 Analog inputs Settings"
  # "USB6218 Digital Output Settings"
  # "USB6218 Analog Output Settings"
  # "LSI218 Settings"
  # "LSI336 Settings"
  # "Graph screenshots"
  # "Configuration"
  # "Activated only when *FIll state* = TRUE"
  # "Activated only when *FIll state* = TRUE"
  # "Vavle Status"
  # "OPEN"
  # "CLOSED"
  # "ADCMT6240A Control/Status"
  # "ADCMT6240A Initialization"
  # "Set Currents (mA)"
  # "KIKUSUI PWR400H CTRL via USB6218"
  # "Representative temperatures"
  # "Pressures / Flows"
  # "Labels"
  # "Helium Levels"
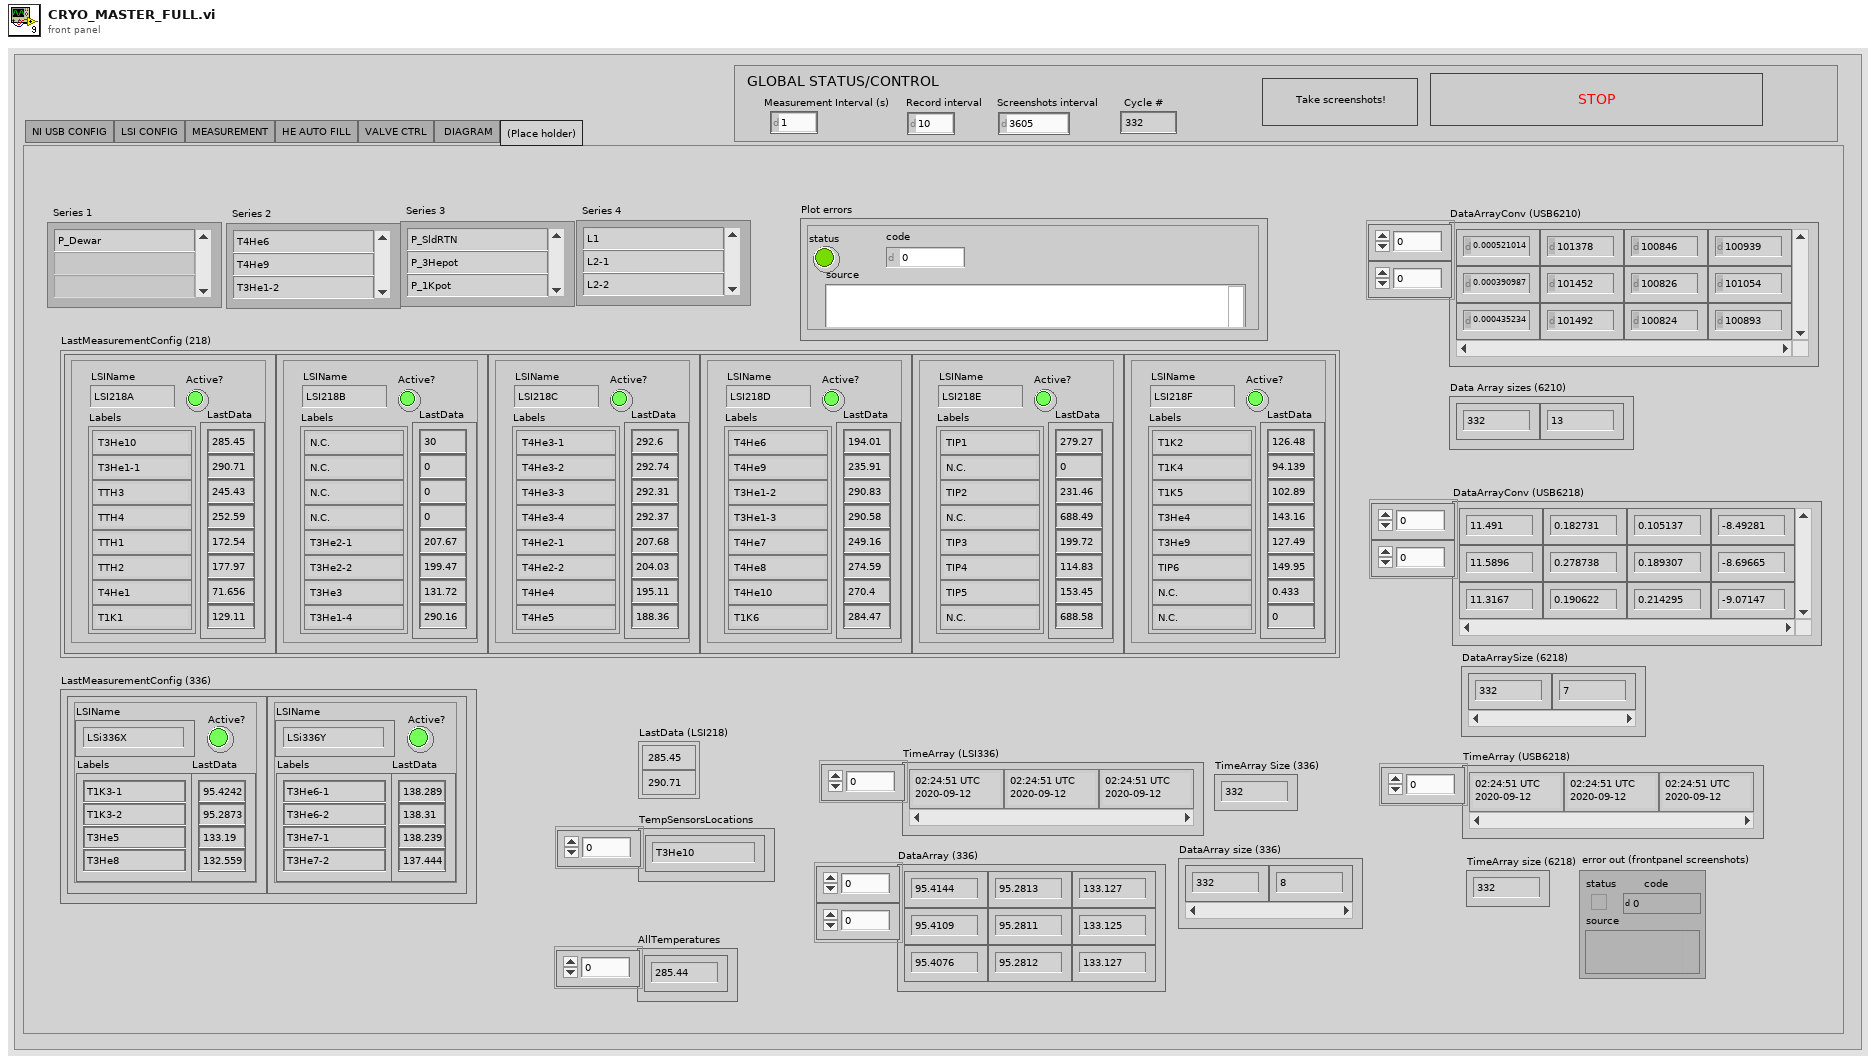
[diagram p1: front panel]
types:
  T1 = enum32{"NI USB CONFIG", "LSI CONFIG", "MEASUREMENT", "HE AUTO FILL", "VALVE CTRL", " DIAGRAM", "(Place holder)"}
  T2 = cluster{"Label":string, "FileFormat":string, "Active?":bool, "Physical CH":tag, " terminal\n type":i32, "ConversionType":cluster{"Type":enum16{"Raw", "SimpleProp", "CC-10_COMBINED", "CC-10_LOG", "LeakDet_EXP", "LeakDet_Mantissa", "Baratron"}, "ConversionParameters":dbl[]}, "VoltageLimits":dbl[]}[]
  T3 = cluster{"LSIName":string, "Labels":string[], "SensorLocations":enum16{"N.C.", "T3He1-1", "T3He1-2", "T3He1-3", "T3He1-4", "T3He2-1", "T3He2-2", "T3He3", "T3He4", "T3He5", "T3He6-1", "T3He6-2", "T3He7-1", "T3He7-2", "T3He8", "T3He9", "T3He10", "T4He1", "T4He2-1", "T4He2-2", "T4He3-1", "T4He3-2", "T4He3-3", "T4He3-4", "T4He4", "T4He5", "T4He6", "T4He7", "T4He8", "T4He9", "T4He10", "T1K1", "T1K2", "T1K3-1", "T1K3-2", "T1K4", "T1K5", "T1K6", "TIP1", "TIP2", "TIP3", "TIP4", "TIP5", "TIP6", "TIP7", "TTH1", "TTH2", "TTH3", "TTH4"}[], "Active?":bool, "VISA res. name":refnum<visa-resource-name>}[]
  T4 = cluster{"TimeArray":timestamp[], "DataArray":dbl[]}[]
  T5 = enum32{"USB6210", "USB6218", "Temeprature (1)", "Temperature (2)", "Temperature (3)"}
  T6 = enum16{"Intialized", "Ready", "Measuring", "Terminated"}
  T7 = enum16{"Initialized", "Ready", "Measuring", "Terminated"}
  T8 = cluster{"TimeArray":timestamp[], "Filtered X":dbl[]}[]
  T9 = cluster{"TimeArray (USB6218)":timestamp[], "DataArrayConv (USB6218)":dbl[]}[]
  T10 = enum16{"N.C.", "T3He1-1", "T3He1-2", "T3He1-3", "T3He1-4", "T3He2-1", "T3He2-2", "T3He3", "T3He4", "T3He5", "T3He6-1", "T3He6-2", "T3He7-1", "T3He7-2", "T3He8", "T3He9", "T3He10", "T4He1", "T4He2-1", "T4He2-2", "T4He3-1", "T4He3-2", "T4He3-3", "T4He3-4", "T4He4", "T4He5", "T4He6", "T4He7", "T4He8", "T4He9", "T4He10", "T1K1", "T1K2", "T1K3-1", "T1K3-2", "T1K4", "T1K5", "T1K6", "TIP1", "TIP2", "TIP3", "TIP4", "TIP5", "TIP6", "TIP7", "TTH1", "TTH2", "TTH3", "TTH4"}
  T11 = cluster{"LSIName":string, "Active?":bool, "LastData":dbl[], "Labels":string[]}[]
  T12 = enum16{"N.C.", "T3He1-1", "T3He1-2", "T3He1-3", "T3He1-4", "T3He2-1", "T3He2-2", "T3He3", "T3He4", "T3He5", "T3He6-1", "T3He6-2", "T3He7-1", "T3He7-2", "T3He8", "T3He9", "T3He10", "T4He1", "T4He2-1", "T4He2-2", "T4He3-1", "T4He3-2", "T4He3-3", "T4He3-4", "T4He4", "T4He5", "T4He6", "T4He7", "T4He8", "T4He9", "T4He10", "T1K1", "T1K2", "T1K3-1", "T1K3-2", "T1K4", "T1K5", "T1K6", "TIP1", "TIP2", "TIP3", "TIP4", "TIP5", "TIP6", "TIP7", "TTH1", "TTH2", "TTH3", "TTH4"}[]
  T13 = cluster{"appended array":timestamp[], "ActualCurrentArray":dbl[]}
  T14 = cluster{"appended array":timestamp[], "SetCurrentArray":dbl[]}
  T15 = cluster{"appended array":timestamp[], "SetCurrentArray":dbl[]}[]
  T16 = cluster{"TimeArray (USB6218)":timestamp[], "DataArrayConv (USB6218)":dbl[]}
  T17 = enum16{"open", "replace", "create", "open or create", "replace or create", "replace or create with confirmation"}
  T18 = cluster{"TimeArray":timestamp[], "DataArrayConv":dbl[]}[]
  T19 = cluster{"IndexArray":i64[], "TimeArray":timestamp[], "DataArrayRaw":dbl[][], "DataArrayConv":dbl[][], "LDArray":dbl[]}
  T20 = cluster{"InstName":string, "Active?":bool, "Status":enum16{"Intialized", "Ready", "Measuring", "Terminated"}, "Labels":string[], "LabelLD":string, "FileFormat":string[], "FileFormatLD":string, "ReadLeakDet?":bool}
  T21 = cluster{"TimeArray":timestamp[], "DataArrayConv":dbl[]}
  T22 = cluster{"TimeArray":timestamp[], "M.A. Array":dbl[]}
  T23 = cluster{"TimeArray":timestamp[], "M.A. Array":dbl[]}[]
  T24 = cluster{"TimeArray":timestamp[], "DataArray":dbl[]}
  T25 = typedef "imagedata.ctl" = cluster{"image type":i32, "image depth":i32, "image":u8[], "mask":u8[], "colors":u32[], "Rectangle":cluster{"left":i16, "top":i16, "right":i16, "bottom":i16}}
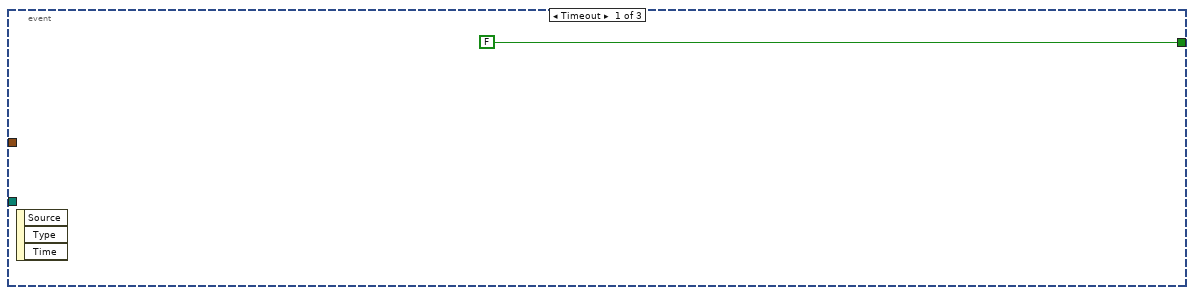
[diagram p2: hidden frame]
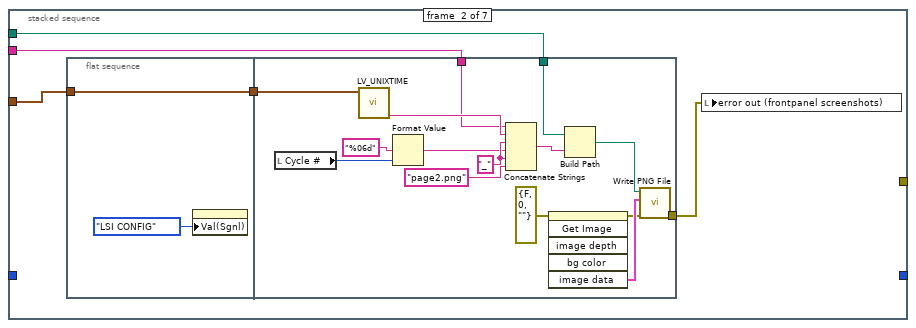
[diagram p3: hidden frame]
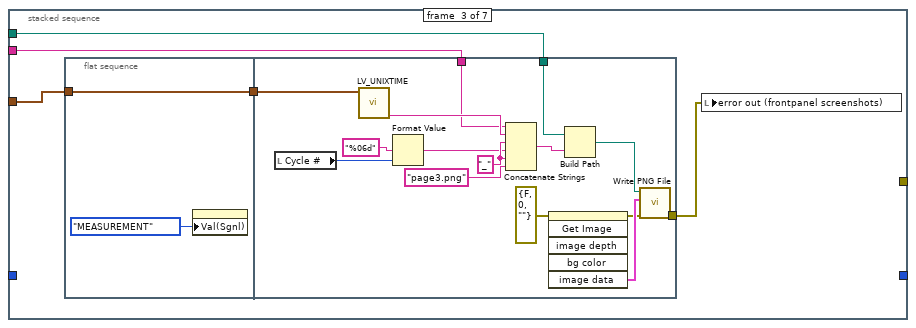
[diagram p4: hidden frame]
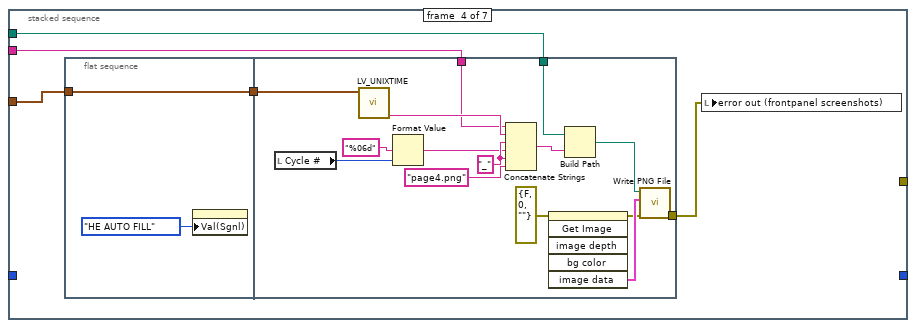
[diagram p5: hidden frame]
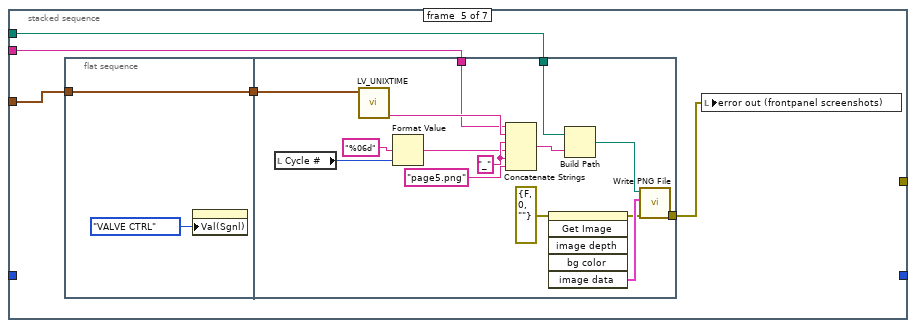
[diagram p6: hidden frame]
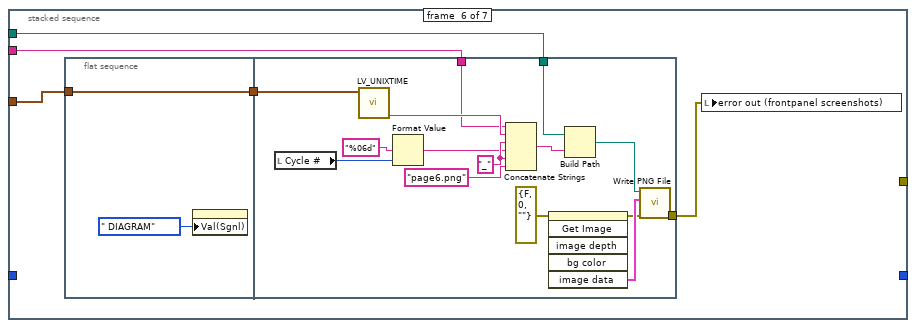
[diagram p7: hidden frame]
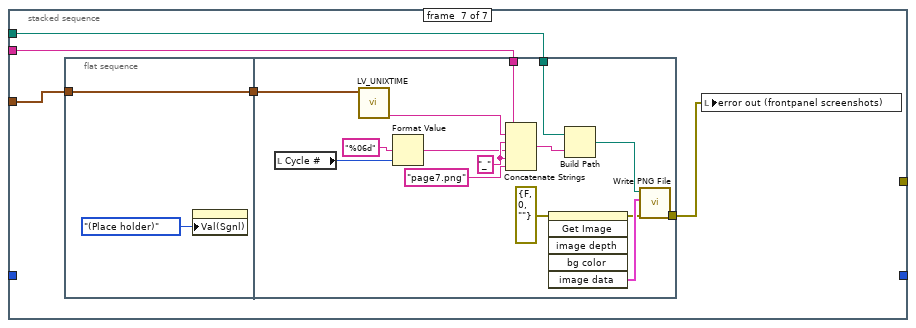
[diagram p8: hidden frame]
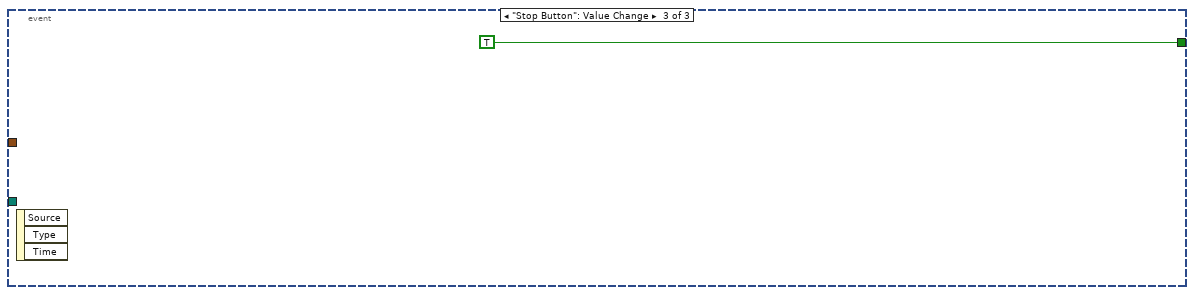
[diagram p9: hidden frame]
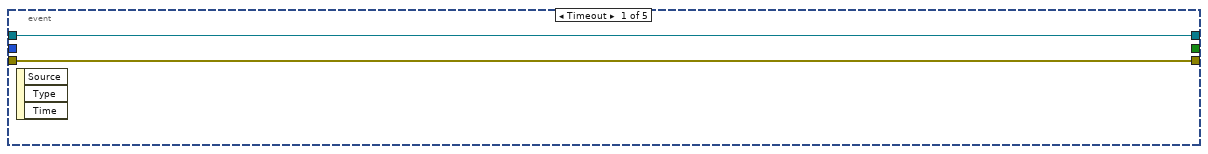
[diagram p11: hidden frame]
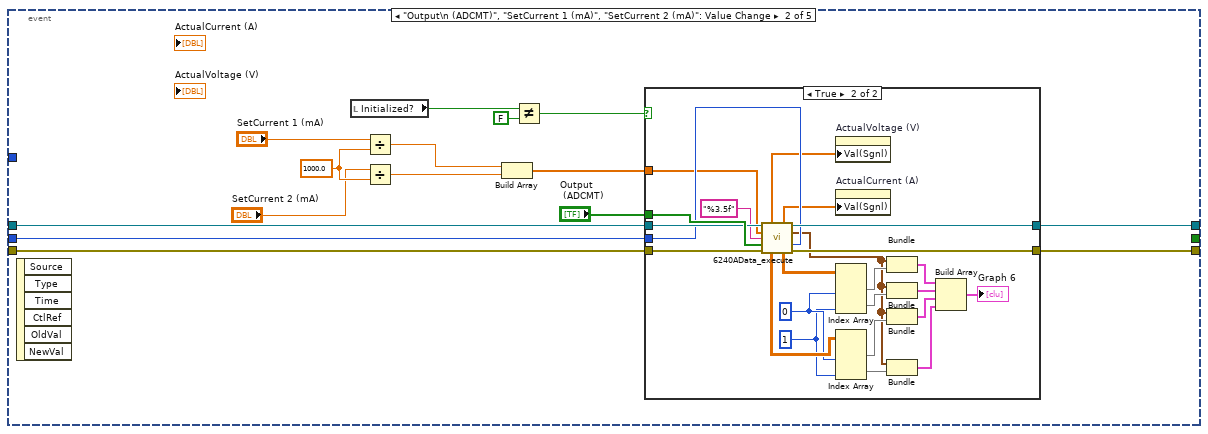
[diagram p12: hidden frame]
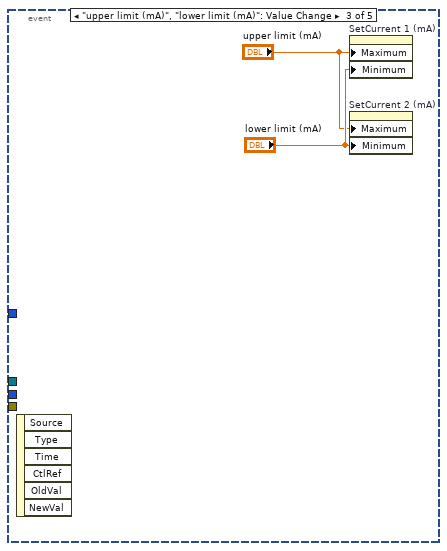
[diagram p14: hidden frame]
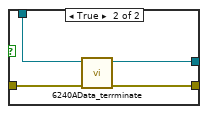
[diagram p15: hidden frame]
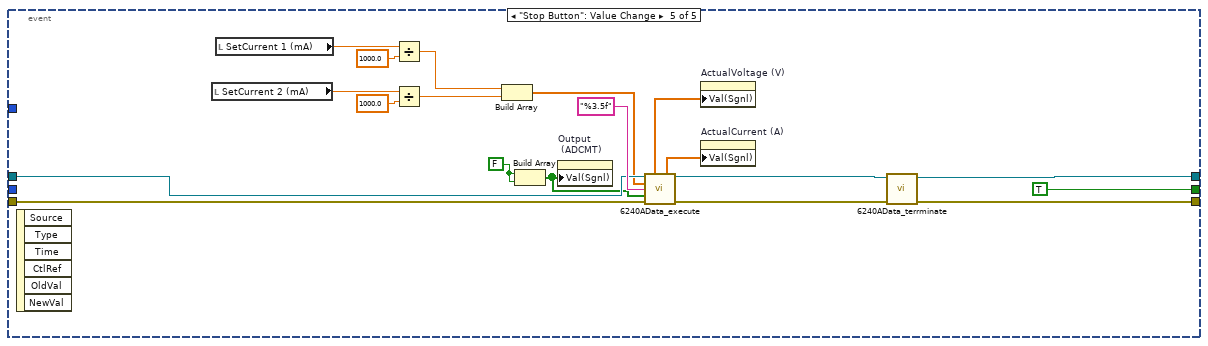
[diagram p16: hidden frame]
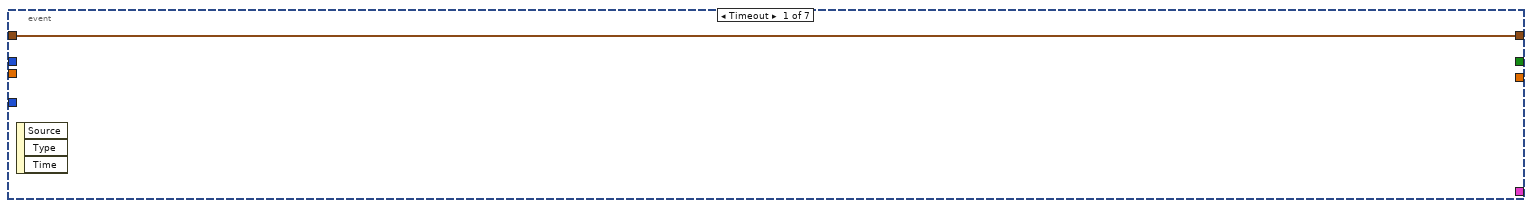
[diagram p17: hidden frame]
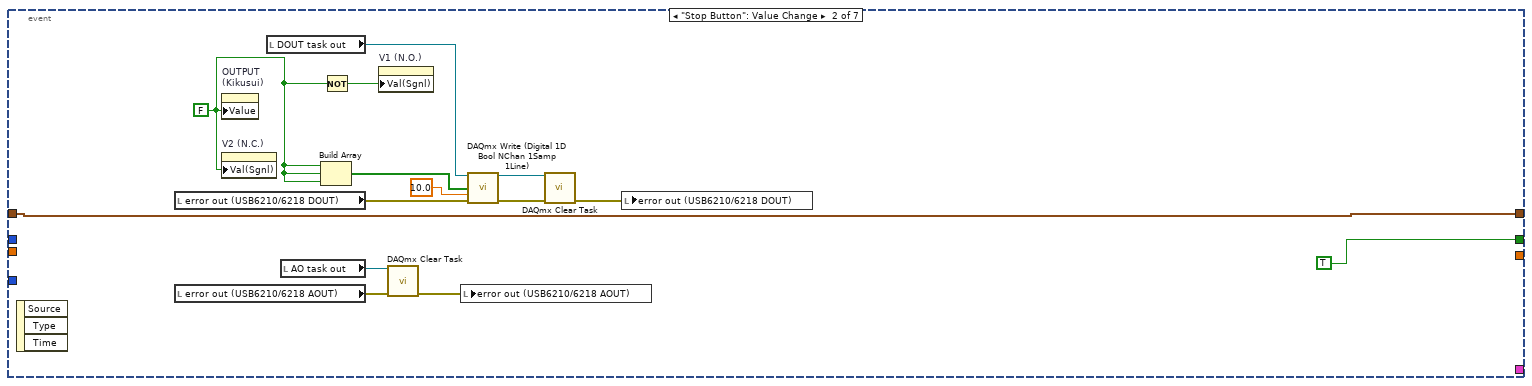
[diagram p18: hidden frame]
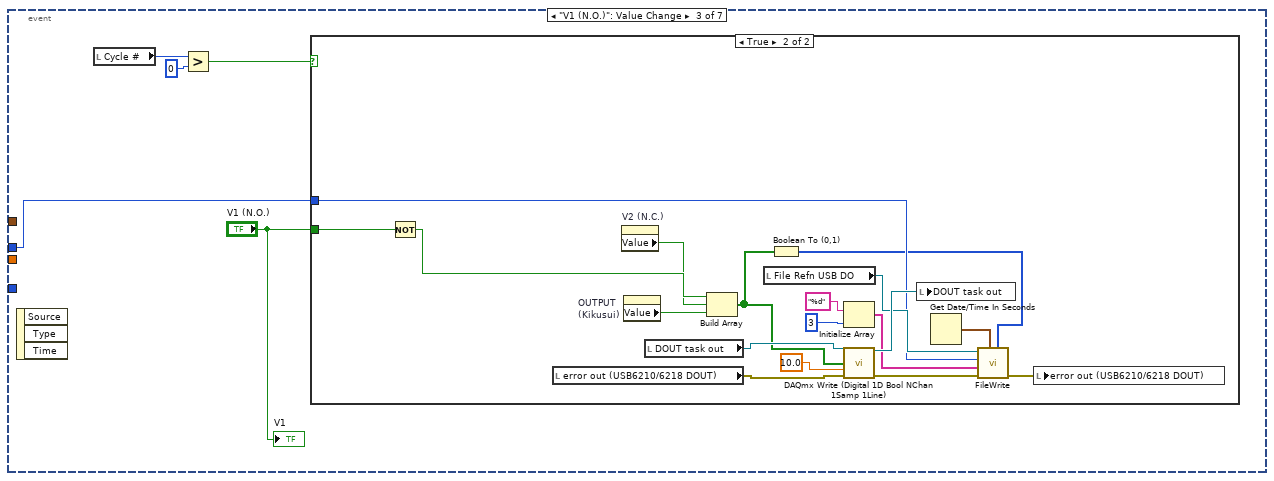
[diagram p19: hidden frame]
diagram:
  w3 = errorcluster {"status"=FALSE, "code"=0, "source"=""} ("error in (no error)")
  n1 = while {
    stop <- w31 stop-if-true
    n2 = event shown="[6] \"Take Screenshot! 1\": Value Change" {
      selector: _ -> [_ _ _ _ _ _ _ _ _ _ _]
      dyn-events: _ -> [_ _ _ _ _ _ _ _ _ _ _]
      timeout: _ -> [_ _ _ _ _ _ _ _ _ _ _]
      tunnel: [_ _ _ _ _ _ _ _ _ _ TRUE] -> w31
      event Timeout {
        n3 = event-data() -> ()  [unwired: 1 in, 3 out]
      }
      event "log/linear 1": Value Change {
        n4 = event-data() -> ()  [unwired: 1 in, 6 out]
        n5 = flat-sequence {
          frame #0 {
            n6 = control-ref of="Graph 1"() -> (w34:refnum<vi>)
            n7 = Boolean To (0,1)(Boolean="log/linear 1") -> (0, 1=w38:i16)
            n8 = property class="XYGraph (strict)"(reference=w34, error in=errorcluster {"status"=FALSE, "code"=0, "source"=""} ("error in (no error)"), "YScale.Mapping Mode"=w38) -> (error out=w36:errorcluster)  [unwired: 1 out]
            n9 = control-ref of="error out (USB6210)"() -> (w37:refnum<vi>)
            n10 = property class="Clust (strict)"(reference=w37, "Val(Sgnl)"=w36) -> ()  [unwired: 1 in, 2 out]
          }
        }
      }
      event "log/linear 2": Value Change {
        n11 = event-data() -> ()  [unwired: 1 in, 6 out]
        n12 = flat-sequence {
          frame #0 {
            n13 = control-ref of="Graph 2"() -> (w42:refnum<vi>)
            n14 = Boolean To (0,1)(Boolean="log/linear 2") -> (0, 1=w44:i16)
            n15 = property class="XYGraph (strict)"(reference=w42, error in=errorcluster {"status"=FALSE, "code"=0, "source"=""} ("error in (no error)"), "YScale.Mapping Mode"=w44) -> (error out=w43:errorcluster)  [unwired: 1 out]
            n16 = control-ref of="error out (USB6210)"() -> (w41:refnum<vi>)
            n17 = property class="Clust (strict)"(reference=w41, "Value"=w43) -> ()  [unwired: 1 in, 2 out]
          }
        }
      }
      event "log/linear 3": Value Change {
        n18 = event-data() -> ()  [unwired: 1 in, 6 out]
        n19 = flat-sequence {
          frame #0 {
            n20 = control-ref of="Graph 3"() -> (w46:refnum<vi>)
            n21 = Boolean To (0,1)(Boolean="log/linear 3") -> (0, 1=w50:i16)
            n22 = property class="XYGraph (strict)"(reference=w46, error in=errorcluster {"status"=FALSE, "code"=0, "source"=""} ("error in (no error)"), "YScale.Mapping Mode"=w50) -> (error out=w49:errorcluster)  [unwired: 1 out]
            n23 = control-ref of="error out (USB6210)"() -> (w48:refnum<vi>)
            n24 = property class="Clust (strict)"(reference=w48, "Value"=w49) -> ()  [unwired: 1 in, 2 out]
          }
        }
      }
      event "log/linear 4": Value Change {
        n25 = event-data() -> ()  [unwired: 1 in, 6 out]
        n26 = flat-sequence {
          frame #0 {
            n27 = control-ref of="Graph 4"() -> (w52:refnum<vi>)
            n28 = Boolean To (0,1)(Boolean="log/linear 4") -> (0, 1=w56:i16)
            n29 = property class="XYGraph (strict)"(reference=w52, error in=errorcluster {"status"=FALSE, "code"=0, "source"=""} ("error in (no error)"), "YScale.Mapping Mode"=w56) -> (error out=w55:errorcluster)  [unwired: 1 out]
            n30 = control-ref of="error out (USB6210)"() -> (w54:refnum<vi>)
            n31 = property class="Clust (strict)"(reference=w54, "Value"=w55) -> ()  [unwired: 1 in, 2 out]
          }
        }
      }
      event "Plot selecter LSI218(1)\n    1      2     3     4", "Plot selecter LSI218(2)\n    1      2     3     4", "Plot selecter (USB6210)\n    1      2     3     4", "Plot selecter LSI336 \n     1      2     3     4", "Plot selecter (USB6218)\n    1      2     3     4": Value Change {
        n32 = event-data() -> ()  [unwired: 1 in, 6 out]
        n33 = local read "All Labels (USB6210)"() -> (w74:string[])
        n34 = local read "All Labels (USB6218)"() -> (w63:string[])
        n35 = local read "Labels LSI218 (1)"() -> (w76:string[])
        n36 = local read "Labels LSI218 (2)"() -> (w77:string[])
        n37 = local read "Labels LSI336"() -> (w69:string[])
        n38 = call "BuildPlotLegends.vi"("Plot selecter \n    1      2     3     4"="Plot selecter (USB6210)\n    1      2     3     4", "AllLabels"=w74) -> ("Series 4"=w86:string[], "Series 3"=w84:string[], "Series 2"=w82:string[], "Series 1"=w80:string[])  [unwired: 6 in]
        n39 = call "BuildPlotLegends_LSI218.vi"("Plot selecter (2)\n    1      2     3     5"="Plot selecter LSI218(2)\n    1      2     3     4", "Plot selecter (1)\n    1      2     3     4"="Plot selecter LSI218(1)\n    1      2     3     4", "Labels (2)"=w77, "Labels (1)"=w76) -> ("Series 4"=w87:string[], "Series 3"=w85:string[], "Series 2"=w83:string[], "Series 1"=w81:string[])  [unwired: 4 in]
        n40 = call "BuildPlotLegends.vi"("Plot selecter \n    1      2     3     4"="Plot selecter LSI336 \n     1      2     3     4", "AllLabels"=w69) -> ("Series 4"=w64:string[], "Series 3"=w65:string[], "Series 2"=w66:string[], "Series 1"=w67:string[])  [unwired: 6 in]
        n41 = call "BuildPlotLegends.vi"("Plot selecter \n    1      2     3     4"="Plot selecter (USB6218)\n    1      2     3     4", "AllLabels"=w63) -> ("Series 4"=w59:string[], "Series 3"=w58:string[], "Series 2"=w60:string[], "Series 1"=w61:string[])  [unwired: 6 in]
        n42 = Build Array (concatenate)(w82, w83, w66, w60) -> (w71:string[])
        "Series 2" <- w71
        n43 = Build Array (concatenate)(w84, w85, w65, w58) -> (w72:string[])
        "Series 3" <- w72
        n44 = Build Array (concatenate)(w86, w87, w64, w59) -> (w73:string[])
        "Series 4" <- w73
        n45 = Build Array (concatenate)(w80, w81, w67, w61) -> (w70:string[])
        "Series 1" <- w70
        n46 = stacked-sequence {
          tunnel: [w97 _ _ _] -> w91
          tunnel: [_ w115 _ _] -> w92
          tunnel: [_ _ w132 _] -> w90
          tunnel: [_ _ _ w148] -> w89
          tunnel: w70 -> [w94 _ _ _]
          tunnel: w71 -> [_ w111 _ _]
          tunnel: w72 -> [_ _ w129 _]
          tunnel: w73 -> [_ _ _ w145]
          frame #0 {
            n47 = Array Size(array=w94) -> (size(s)=w99:i32)
            n48 = control-ref of="Graph 1"() -> (w93:refnum<vi>)
            n49 = for {
              N: 18 -> [_]
              tunnel: w93 -> [w108]
              shift-right: [w106] -> w98
              shift-left: errorcluster {"status"=FALSE, "code"=0, "source"=""} ("error in (no error)") -> [w107]
              i -> [w110]
              n50 = property class="XYGraph (strict)"(reference=w108, error in=w107, "Active Plot"=w110, "Plot.Plot Name"="") -> (error out=w106:errorcluster)  [unwired: 1 out]
            }
            n51 = for {
              N: w99 -> [_]
              tunnel: w93 -> [w104]
              shift-right: [w102] -> w97
              shift-left: w98 -> [w103]
              tunnel: w94 -> [w101] mode=indexing
              i -> [w105]
              n52 = property class="XYGraph (strict)"(reference=w104, error in=w103, "Active Plot"=w105, "Plot.Plot Name"=w101, "Plot.Visible?"=TRUE ("Plot.Visible")) -> (error out=w102:errorcluster)  [unwired: 1 out]
            }
          }
          frame #1 {
            n53 = Array Size(array=w111) -> (size(s)=w117:i32)
            n54 = control-ref of="Graph 2"() -> (w114:refnum<vi>)
            n55 = for {
              N: 18 -> [_]
              shift-right: [w124] -> w116
              shift-left: errorcluster {"status"=FALSE, "code"=0, "source"=""} ("error in (no error)") -> [w125]
              tunnel: w114 -> [w123]
              i -> [w127]
              n56 = property class="XYGraph (strict)"(reference=w123, error in=w125, "Active Plot"=w127, "Plot.Plot Name"="") -> (error out=w124:errorcluster)  [unwired: 1 out]
            }
            n57 = for {
              N: w117 -> [_]
              shift-right: [w120] -> w115
              shift-left: w116 -> [w121]
              tunnel: w111 -> [w119] mode=indexing
              tunnel: w114 -> [w118]
              i -> [w122]
              n58 = property class="XYGraph (strict)"(reference=w118, error in=w121, "Active Plot"=w122, "Plot.Plot Name"=w119) -> (error out=w120:errorcluster)  [unwired: 1 out]
            }
          }
          frame #2 {
            n59 = Array Size(array=w129) -> (size(s)=w134:i32)
            n60 = control-ref of="Graph 3"() -> (w128:refnum<vi>)
            n61 = for {
              N: 18 -> [_]
              tunnel: w128 -> [w142]
              shift-right: [w140] -> w133
              shift-left: errorcluster {"status"=FALSE, "code"=0, "source"=""} ("error in (no error)") -> [w141]
              i -> [w144]
              n62 = property class="XYGraph (strict)"(reference=w142, error in=w141, "Active Plot"=w144, "Plot.Plot Name"="") -> (error out=w140:errorcluster)  [unwired: 1 out]
            }
            n63 = for {
              N: w134 -> [_]
              tunnel: w128 -> [w138]
              shift-right: [w136] -> w132
              shift-left: w133 -> [w137]
              tunnel: w129 -> [w135] mode=indexing
              i -> [w139]
              n64 = property class="XYGraph (strict)"(reference=w138, error in=w137, "Active Plot"=w139, "Plot.Plot Name"=w135) -> (error out=w136:errorcluster)  [unwired: 1 out]
            }
          }
          frame #3 {
            n65 = Array Size(array=w145) -> (size(s)=w151:i32)
            n66 = control-ref of="Graph 4"() -> (w149:refnum<vi>)
            n67 = for {
              N: 18 -> [_]
              tunnel: w149 -> [w159]
              shift-right: [w157] -> w150
              shift-left: errorcluster {"status"=FALSE, "code"=0, "source"=""} ("error in (no error)") -> [w158]
              i -> [w161]
              n68 = property class="XYGraph (strict)"(reference=w159, error in=w158, "Active Plot"=w161, "Plot.Plot Name"="") -> (error out=w157:errorcluster)  [unwired: 1 out]
            }
            n69 = for {
              N: w151 -> [_]
              tunnel: w149 -> [w155]
              shift-right: [w153] -> w148
              shift-left: w150 -> [w154]
              tunnel: w145 -> [w152] mode=indexing
              i -> [w156]
              n70 = property class="XYGraph (strict)"(reference=w155, error in=w154, "Active Plot"=w156, "Plot.Plot Name"=w152) -> (error out=w153:errorcluster)  [unwired: 1 out]
            }
          }
        }
        n71 = Merge Errors(w91, w92, w90, w89) -> (→"Plot errors":errorcluster)
      }
      event "Take Screenshot! 1": Value Change {
        n72 = event-data() -> ()  [unwired: 1 in, 6 out]
        n73 = flat-sequence {
          frame #0 {
            n74 = flat-sequence {
              frame #0 {
                w166 = "_" ("string")
                n75 = Get Date/Time In Seconds() -> (seconds since 1Jan1904=w163:timestamp)
                n76 = local read "RUN identifier"() -> (w169:string)
                n77 = call "LV_UNIXTIME.vi"("current time"=w163) -> ("date/time string"=w167:string)  [unwired: 9 in, 1 out]
                n78 = local read "Base Path"() -> (w170:path)
                n79 = Concatenate Strings(w169, w166, w167, w166, "FIle suffix 1", ".bmp" ("string")) -> (w175:string)
                n80 = control-ref of="Graph 1"() -> (w162:refnum<vi>)
                n81 = Build Path(base path=w170, name or relative path=w175) -> (appended path=w174:path)
                n82 = invoke on="Invoke Node" class="XYGraph (strict)" method="Export Image"(reference=w162, "FileType"=enum32{"BMP", "EPS", "EMF", "PICT"}."BMP" ("File Type"), "Target"=enum32{"File", "Clipboard"}."File", "Path"=w174, "HideGrid"=FALSE ("Hide Grid"), "Overwrite"=TRUE ("Always Overwrite")) -> ()  [unwired: 2 in, 8 out]
              }
              frame #1 {
                n83 = local write "Take Screenshot! 1"(FALSE ("Take Screenshot! 1")) -> ()
              }
            }
          }
        }
      }
      event "Take Screenshot! 2": Value Change {
        n84 = event-data() -> ()  [unwired: 1 in, 6 out]
        n85 = flat-sequence {
          frame #0 {
            n86 = flat-sequence {
              frame #0 {
                w181 = "_" ("string")
                n87 = Get Date/Time In Seconds() -> (seconds since 1Jan1904=w177:timestamp)
                n88 = local read "RUN identifier"() -> (w184:string)
                n89 = call "LV_UNIXTIME.vi"("current time"=w177) -> ("date/time string"=w182:string)  [unwired: 9 in, 1 out]
                n90 = local read "Base Path"() -> (w185:path)
                n91 = Concatenate Strings(w184, w181, w182, w181, "FIle suffix 2", ".bmp" ("string")) -> (w190:string)
                n92 = control-ref of="Graph 2"() -> (w178:refnum<vi>)
                n93 = Build Path(base path=w185, name or relative path=w190) -> (appended path=w189:path)
                n94 = invoke on="Invoke Node" class="XYGraph (strict)" method="Export Image"(reference=w178, "FileType"=enum32{"BMP", "EPS", "EMF", "PICT"}."BMP" ("File Type"), "Target"=enum32{"File", "Clipboard"}."File", "Path"=w189, "HideGrid"=FALSE ("Hide Grid"), "Overwrite"=TRUE ("Always Overwrite")) -> ()  [unwired: 2 in, 8 out]
              }
              frame #1 {
                n95 = local write "Take Screenshot! 2"(FALSE ("Take Screenshot! 1")) -> ()
              }
            }
          }
        }
      }
      event "Take Screenshot! 3": Value Change {
        n96 = event-data() -> ()  [unwired: 1 in, 6 out]
        n97 = flat-sequence {
          frame #0 {
            n98 = flat-sequence {
              frame #0 {
                w196 = "_" ("string")
                n99 = Get Date/Time In Seconds() -> (seconds since 1Jan1904=w194:timestamp)
                n100 = local read "RUN identifier"() -> (w199:string)
                n101 = call "LV_UNIXTIME.vi"("current time"=w194) -> ("date/time string"=w197:string)  [unwired: 9 in, 1 out]
                n102 = local read "Base Path"() -> (w200:path)
                n103 = Concatenate Strings(w199, w196, w197, w196, "FIle suffix 3", ".bmp" ("string")) -> (w205:string)
                n104 = control-ref of="Graph 3"() -> (w192:refnum<vi>)
                n105 = Build Path(base path=w200, name or relative path=w205) -> (appended path=w204:path)
                n106 = invoke on="Invoke Node" class="XYGraph (strict)" method="Export Image"(reference=w192, "FileType"=enum32{"BMP", "EPS", "EMF", "PICT"}."BMP" ("File Type"), "Target"=enum32{"File", "Clipboard"}."File", "Path"=w204, "HideGrid"=FALSE ("Hide Grid"), "Overwrite"=TRUE ("Always Overwrite")) -> ()  [unwired: 2 in, 8 out]
              }
              frame #1 {
                n107 = local write "Take Screenshot! 3"(FALSE ("Take Screenshot! 1")) -> ()
              }
            }
          }
        }
      }
      event "Take Screenshot! 4": Value Change {
        n108 = event-data() -> ()  [unwired: 1 in, 6 out]
        n109 = flat-sequence {
          frame #0 {
            n110 = flat-sequence {
              frame #0 {
                w211 = "_" ("string")
                n111 = Get Date/Time In Seconds() -> (seconds since 1Jan1904=w209:timestamp)
                n112 = local read "RUN identifier"() -> (w214:string)
                n113 = call "LV_UNIXTIME.vi"("current time"=w209) -> ("date/time string"=w212:string)  [unwired: 9 in, 1 out]
                n114 = local read "Base Path"() -> (w215:path)
                n115 = Concatenate Strings(w214, w211, w212, w211, "FIle suffix 4", ".bmp" ("string")) -> (w220:string)
                n116 = control-ref of="Graph 4"() -> (w207:refnum<vi>)
                n117 = Build Path(base path=w215, name or relative path=w220) -> (appended path=w219:path)
                n118 = invoke on="Invoke Node" class="XYGraph (strict)" method="Export Image"(reference=w207, "FileType"=enum32{"BMP", "EPS", "EMF", "PICT"}."BMP" ("File Type"), "Target"=enum32{"File", "Clipboard"}."File", "Path"=w219, "HideGrid"=FALSE ("Hide Grid"), "Overwrite"=TRUE ("Always Overwrite")) -> ()  [unwired: 2 in, 8 out]
              }
              frame #1 {
                n119 = local write "Take Screenshot! 4"(FALSE ("Take Screenshot! 1")) -> ()
              }
            }
          }
        }
      }
      event "Stop Button": Value Change {
        n120 = event-data() -> ()  [unwired: 1 in, 6 out]
      }
    }
    n121 = local write "Take Screenshot! 4"(FALSE ("Take Screenshot! 1")) -> ()
    n122 = local write "Take Screenshot! 1"(FALSE ("Take Screenshot! 1")) -> ()
    n123 = local write "Take Screenshot! 2"(FALSE ("Take Screenshot! 1")) -> ()
    n124 = local write "Take Screenshot! 3"(FALSE ("Take Screenshot! 1")) -> ()
    n125 = Wait (ms)(milliseconds to wait=u32 1000) -> ()  [unwired: 1 out]
  }
  n126 = while {
    shift-right: [w231] -> _
    shift-left: refnum<class "6240AData.lvclass"> refnum ("6240AData.lvclass") -> [w229]
    shift-right: [w227] -> _
    shift-left: errorcluster {"status"=FALSE, "code"=0, "source"=""} ("error in (no error)") -> [w228]
    i -> [w223]
    stop <- w230 stop-if-true
    n127 = Wait (ms)(milliseconds to wait=u32 231) -> ()  [unwired: 1 out]
    n128 = Equal?(x=w223, y=0) -> (x = y?=w225:bool)
    n129 = case shown="True" w225 {
      frame False {
      }
      frame True {
        n130 = property on="Initialized?" class="Bool (strict)"("Val(Sgnl)"=FALSE ("Value (Signaling)")) -> ()  [unwired: 2 in, 2 out]
      }
    }
    n131 = event shown="[3] \"Initialize\": Value Change" {
      selector: _ -> [_ _ _ _ _]
      dyn-events: _ -> [_ _ _ _ _]
      timeout: _ -> [_ _ _ _ _]
      tunnel: [w234 w249 _ w298 w331] -> w231
      tunnel: [_ _ _ _ TRUE ("Value (Signaling)")] -> w230
      tunnel: w229 -> [w234 w248 _ w282 w325]
      tunnel: w228 -> [w233 w247 _ w281 w323]
      tunnel: [w233 w246 _ w296 w330] -> w227
      tunnel: w223 -> [_ w245 _ _ _]
      tunnel: w223 -> [_ _ _ w290 _]
      event Timeout {
        n132 = event-data() -> ()  [unwired: 1 in, 3 out]
      }
      event "Output\n (ADCMT)", "SetCurrent 1 (mA)", "SetCurrent 2 (mA)": Value Change {
        w238 = 1000.0 ("y")
        n133 = event-data() -> ()  [unwired: 1 in, 6 out]
        n134 = local read "Initialized?"() -> (w244:bool)
        n135 = Divide(x="SetCurrent 1 (mA)", y=w238) -> (x/y=w239:dbl)
        n136 = Divide(x="SetCurrent 2 (mA)", y=w238) -> (x/y=w240:dbl)
        n137 = Build Array(w239, w240) -> (w237:dbl[])
        n138 = Not Equal?(x=w244, y=FALSE) -> (x != y?=w242:bool)
        n139 = case shown="True" w242 {
          tunnel: [w251 w275] -> w249
          tunnel: "Output\n (ADCMT)" -> [_ w274]
          tunnel: w248 -> [w251 w273]
          tunnel: w247 -> [w250 w272]
          tunnel: [w250 w271] -> w246
          tunnel: w245 -> [_ w267]
          tunnel: w237 -> [_ w253]
          frame False {
          }
          frame True {
            w260 = 1 ("index (col)")
            w261 = 0 ("disabled index (col)")
            n140 = call-dynamic "6240AData_execute.vi"("6240AData in"=w273, "SetCurrent (A)"=w253, "FileFormat"="%3.5f", "Output status"=w274, "ExecutionIndex"=w267, "error in (no error)"=w272) -> ("ActualVoltage (V)"=w252:dbl[], "ActualCurrent (A)"=w266:dbl[], "6240AData out"=w275:refnum<class "6240AData.lvclass">, "appended array"=w256:timestamp[], "SetCurrentArray"=w262:dbl[][], "ActualCurrentArray"=w269:dbl[][], "error out"=w271:errorcluster)  [unwired: 3 in]
            n141 = property on="ActualVoltage (V)" class="Arr (strict)"("Val(Sgnl)"=w252) -> ()  [unwired: 2 in, 2 out]
            n142 = property on="ActualCurrent (A)" class="Arr (strict)"("Val(Sgnl)"=w266) -> ()  [unwired: 2 in, 2 out]
            n143 = Index Array(array=w269, index (col) #1=w261, index (col) #2=w260) -> (element #1=w270:dbl[], element #2=w264:dbl[])  [unwired: 2 in]
            n144 = Index Array(array=w262, index (col) #1=w261, index (col) #2=w260) -> (element #1=w258:dbl[], element #2=w255:dbl[])  [unwired: 2 in]
            n145 = Bundle("appended array"=w256, "ActualCurrentArray"=w270) -> (w265:T13)  [unwired: 1 in]
            n146 = Bundle("appended array"=w256, "ActualCurrentArray"=w264) -> (w259:T13)  [unwired: 1 in]
            n147 = Bundle("appended array"=w256, "SetCurrentArray"=w258) -> (w257:T14)  [unwired: 1 in]
            n148 = Bundle("appended array"=w256, "SetCurrentArray"=w255) -> (w254:T14)  [unwired: 1 in]
            n149 = Build Array(w265, w259, w257, w254) -> (→"Graph 6":T15)
          }
        }
      }
      event "upper limit (mA)", "lower limit (mA)": Value Change {
        n150 = event-data() -> ()  [unwired: 1 in, 6 out]
        n151 = property on="SetCurrent 1 (mA)" class="DigNum (strict)"("Maximum"="upper limit (mA)", "Minimum"="lower limit (mA)") -> ()  [unwired: 2 in, 2 out]
        n152 = property on="SetCurrent 2 (mA)" class="DigNum (strict)"("Maximum"="upper limit (mA)", "Minimum"="lower limit (mA)") -> ()  [unwired: 2 in, 2 out]
      }
      event "Initialize": Value Change {
        w292 = FALSE
        n153 = event-data() -> ()  [unwired: 1 in, 6 out]
        n154 = local read "Initialized?"() -> (w280:bool)
        n155 = case shown="False" w280 {
          tunnel: w282 -> [w309 w313]
          tunnel: w281 -> [w308 w312]
          tunnel: [w309 w311] -> w279
          tunnel: [w308 w310] -> w278
          frame False {
          }
          frame True {
            n156 = call-dynamic "6240AData_terrminate.vi"("error in (no error)"=w312, "6240AData in"=w313) -> ("error out"=w310:errorcluster, "6240AData out"=w311:refnum<class "6240AData.lvclass">)  [unwired: 8 in]
          }
        }
        n157 = local read "SetCurrent 2 (mA)"() -> (w285:dbl)
        n158 = property on="Initialized?" class="Bool (strict)"("Val(Sgnl)"=TRUE ("Value (Signaling)")) -> ()  [unwired: 2 in, 2 out]
        n159 = local read "SetCurrent 1 (mA)"() -> (w288:dbl)
        n160 = local read "RUN identifier"() -> (w300:string)
        n161 = local read "Base Path"() -> (w301:path)
        n162 = Divide(x=w288, y=1000.0) -> (x/y=w287:dbl)
        n163 = Divide(x=w285, y=1000.0) -> (x/y=w284:dbl)
        n164 = Get Date/Time In Seconds() -> (seconds since 1Jan1904=w307:timestamp)
        n165 = call-dynamic "6240AData_initialize.vi"("6240AData in"=w279, "RunName"=w300, "InstName"="InstName", "start time"=w307, "base path"=w301, "VISA"="VISA", "error in (no error)"=w278, "CtrlLabels"="CtrlLabels", "Voltage limits (V)"="Voltage limits (V)") -> ("6240AData out"=w299:refnum<class "6240AData.lvclass">, "error out"=w297:errorcluster)  [unwired: 5 in]
        n166 = Build Array(w287, w284) -> (w283:dbl[])
        n167 = Build Array(w292, w292) -> (w291:bool[])
        n168 = call-dynamic "6240AData_execute.vi"("6240AData in"=w299, "SetCurrent (A)"=w283, "FileFormat"="%3.5f", "Output status"=w291, "ExecutionIndex"=w290, "error in (no error)"=w297) -> ("ActualVoltage (V)"=w294:dbl[], "ActualCurrent (A)"=w293:dbl[], "6240AData out"=w298:refnum<class "6240AData.lvclass">, "error out"=w296:errorcluster)  [unwired: 3 in, 3 out]
        n169 = property on="ActualVoltage (V)" class="Arr (strict)"("Val(Sgnl)"=w294) -> ()  [unwired: 2 in, 2 out]
        n170 = property on="ActualCurrent (A)" class="Arr (strict)"("Val(Sgnl)"=w293) -> ()  [unwired: 2 in, 2 out]
      }
      event "Stop Button": Value Change {
        w329 = FALSE
        n171 = event-data() -> ()  [unwired: 1 in, 6 out]
        n172 = local read "SetCurrent 2 (mA)"() -> (w315:dbl)
        n173 = local read "SetCurrent 1 (mA)"() -> (w319:dbl)
        n174 = Divide(x=w319, y=1000.0) -> (x/y=w317:dbl)
        n175 = Divide(x=w315, y=1000.0) -> (x/y=w314:dbl)
        n176 = Build Array(w317, w314) -> (w321:dbl[])
        n177 = Build Array(w329, w329) -> (w320:bool[])
        n178 = property on="Output\n (ADCMT)" class="Arr (strict)"("Val(Sgnl)"=w320) -> ()  [unwired: 2 in, 2 out]
        n179 = call-dynamic "6240AData_execute.vi"("6240AData in"=w325, "SetCurrent (A)"=w321, "FileFormat"="%3.5f", "Output status"=w320, "error in (no error)"=w323) -> ("ActualVoltage (V)"=w326:dbl[], "ActualCurrent (A)"=w327:dbl[], "6240AData out"=w324:refnum<class "6240AData.lvclass">, "error out"=w322:errorcluster)  [unwired: 4 in, 3 out]
        n180 = property on="ActualVoltage (V)" class="Arr (strict)"("Val(Sgnl)"=w326) -> ()  [unwired: 2 in, 2 out]
        n181 = property on="ActualCurrent (A)" class="Arr (strict)"("Val(Sgnl)"=w327) -> ()  [unwired: 2 in, 2 out]
        n182 = call-dynamic "6240AData_terrminate.vi"("error in (no error)"=w322, "6240AData in"=w324) -> ("error out"=w330:errorcluster, "6240AData out"=w331:refnum<class "6240AData.lvclass">)  [unwired: 8 in]
      }
    }
    "error out (ADCMT6420A)" <- w227
  }
  n183 = while {
    shift-right: [w334] -> _
    shift-left: dbl[] [] -> [w340]
    shift-right: [w337] -> _
    shift-left: timestamp[] [] -> [w339]
    i -> [w338]
    stop <- w341 stop-if-true
    n184 = Wait (ms)(milliseconds to wait=u32 225) -> ()  [unwired: 1 out]
    n185 = event shown="[3] \"V2 (N.C.)\": Value Change" {
      selector: _ -> [_ _ _ _ _ _ _]
      dyn-events: _ -> [_ _ _ _ _ _ _]
      timeout: _ -> [_ _ _ _ _ _ _]
      tunnel: [_ TRUE _ _ _ _ _] -> w341
      tunnel: w338 -> [_ _ _ _ w419 _ _]
      tunnel: [_ _ _ _ w418 w477 _] -> w334
      tunnel: w340 -> [_ _ _ _ w415 w477 _]
      tunnel: [w343 w353 _ _ w417 w476 w482] -> w337
      tunnel: w339 -> [w343 w353 _ _ w416 w476 w482]
      tunnel: w338 -> [_ _ w359 w382 _ _ w483]
      tunnel: [_ _ _ _ w404 _ _] -> w333
      event Timeout {
        n186 = event-data() -> ()  [unwired: 1 in, 3 out]
      }
      event "Stop Button": Value Change {
        w344 = FALSE
        n187 = event-data() -> ()  [unwired: 1 in, 3 out]
        n188 = local read "error out (USB6210/6218 DOUT)"() -> (w352:errorcluster)
        n189 = local read "error out (USB6210/6218 AOUT)"() -> (w349:errorcluster)
        n190 = property on="OUTPUT\n(Kikusui)" class="Bool (strict)"("Value"=w344) -> ()  [unwired: 2 in, 2 out]
        n191 = property on="V2 (N.C.)" class="Bool (strict)"("Val(Sgnl)"=w344) -> ()  [unwired: 2 in, 2 out]
        n192 = local read "DOUT task out"() -> (w348:refnum<k21>)
        n193 = local read "AO task out"() -> (w355:refnum<k21>)
        n194 = Build Array(w344, w344, w344) -> (w351:bool[])
        n195 = Not(x=w344) -> (.not. x?=w345:bool)
        n196 = property on="V1 (N.O.)" class="Bool (strict)"("Val(Sgnl)"=w345) -> ()  [unwired: 2 in, 2 out]
        n197 = call <vilib>:"DAQmx Clear Task.vi"("task in"=w355, "error in"=w349) -> ("error out"=w354:errorcluster)  [unwired: 13 in]
        n198 = local write "error out (USB6210/6218 AOUT)"(w354) -> ()
        n199 = call <vilib>:"DAQmx Write (Digital 1D Bool NChan 1Samp 1Line).vi"("task/channels in"=w348, "data"=w351, "timeout"=10.0, "error in"=w352) -> ("task out"=w347:refnum<k21>, "error out"=w346:errorcluster)  [unwired: 9 in, 1 out]
        n200 = call <vilib>:"DAQmx Clear Task.vi"("task in"=w347, "error in"=w346) -> ("error out"=w356:errorcluster)  [unwired: 13 in]
        n201 = local write "error out (USB6210/6218 DOUT)"(w356) -> ()
      }
      event "V1 (N.O.)": Value Change {
        n202 = event-data() -> ()  [unwired: 1 in, 3 out]
        n203 = local read "Cycle #"() -> (w362:u32)
        n204 = Greater?(x=w362, y=u32 0) -> (0:w360:bool)
        n205 = case shown="True" w360 {
          tunnel: "V1 (N.O.)" -> [_ w375]
          tunnel: w359 -> [_ w370]
          frame False {
          }
          frame True {
            n206 = Not(x=w375) -> (.not. x?=w377:bool)
            n207 = local read "error out (USB6210/6218 DOUT)"() -> (w376:errorcluster)
            n208 = property on="V2 (N.C.)" class="Bool (strict)"() -> ("Value"=w374:bool)  [unwired: 2 in, 2 out]
            n209 = property on="OUTPUT\n(Kikusui)" class="Bool (strict)"() -> ("Value"=w373:bool)  [unwired: 2 in, 2 out]
            n210 = local read "DOUT task out"() -> (w380:refnum<k21>)
            n211 = Build Array(w377, w374, w373) -> (w366:bool[])
            n212 = local read "File Refn USB DO"() -> (w371:refnum<file>)
            n213 = Boolean To (0,1)(Boolean=w366) -> (0, 1=w365:i16[])
            n214 = Initialize Array("%d" ("element"), 3 ("dimension size")) -> (w369:string[])
            n215 = call <vilib>:"DAQmx Write (Digital 1D Bool NChan 1Samp 1Line).vi"("task/channels in"=w380, "data"=w366, "timeout"=10.0, "error in"=w376) -> ("task out"=w378:refnum<k21>, "error out"=w364:errorcluster)  [unwired: 9 in, 1 out]
            n216 = local write "DOUT task out"(w378) -> ()
            n217 = Get Date/Time In Seconds() -> (seconds since 1Jan1904=w372:timestamp)
            n218 = call "FileWrite.vi"("DataArray"=w365, "Time Stamp"=w372, "Error In"=w364, "FileFormat"=w369, "Index"=w370, "refnum in"=w371) -> ("Error Out"=w363:errorcluster)  [unwired: 4 in, 1 out]
            n219 = local write "error out (USB6210/6218 DOUT)"(w363) -> ()
          }
        }
        "V1" <- "V1 (N.O.)"
      }
      event "V2 (N.C.)": Value Change {
        n220 = event-data() -> ()  [unwired: 1 in, 3 out]
        n221 = local read "Cycle #"() -> (w385:u32)
        n222 = Greater?(x=w385, y=u32 0) -> (0:w383:bool)
        n223 = case shown="True" w383 {
          tunnel: "V2 (N.C.)" -> [_ w399]
          tunnel: w382 -> [_ w391]
          frame False {
          }
          frame True {
            n224 = property on="V1 (N.O.)" class="Bool (strict)"() -> ("Value"=w398:bool)  [unwired: 2 in, 2 out]
            n225 = Not(x=w398) -> (.not. x?=w397:bool)
            n226 = local read "error out (USB6210/6218 DOUT)"() -> (w402:errorcluster)
            n227 = property on="OUTPUT\n(Kikusui)" class="Bool (strict)"() -> ("Value"=w396:bool)  [unwired: 2 in, 2 out]
            n228 = local read "DOUT task out"() -> (w403:refnum<k21>)
            n229 = Build Array(w397, w399, w396) -> (w394:bool[])
            n230 = local read "File Refn USB DO"() -> (w395:refnum<file>)
            n231 = Boolean To (0,1)(Boolean=w394) -> (0, 1=w393:i16[])
            n232 = Initialize Array("%d" ("element"), 3 ("dimension size")) -> (w388:string[])
            n233 = call <vilib>:"DAQmx Write (Digital 1D Bool NChan 1Samp 1Line).vi"("task/channels in"=w403, "data"=w394, "timeout"=10.0, "error in"=w402) -> ("task out"=w400:refnum<k21>, "error out"=w387:errorcluster)  [unwired: 9 in, 1 out]
            n234 = local write "DOUT task out"(w400) -> ()
            n235 = Get Date/Time In Seconds() -> (seconds since 1Jan1904=w392:timestamp)
            n236 = call "FileWrite.vi"("DataArray"=w393, "Time Stamp"=w392, "Error In"=w387, "FileFormat"=w388, "Index"=w391, "refnum in"=w395) -> ("Error Out"=w386:errorcluster)  [unwired: 4 in, 1 out]
            n237 = local write "error out (USB6210/6218 DOUT)"(w386) -> ()
          }
        }
        "V2" <- "V2 (N.C.)"
      }
      event "update current", "Set Voltage (V)\n (Kikusui)", "Set Current (mA)\n (Kikusui)": Value Change {
        n238 = event-data() -> ()  [unwired: 1 in, 3 out]
        n239 = case shown="False" "CONTROL KIKUSUI?" {
          tunnel: w419 -> [_ w450]
          tunnel: [w421 w443] -> w418
          tunnel: [w424 w442] -> w417
          tunnel: w416 -> [w426 w445]
          tunnel: w415 -> [w422 w444]
          tunnel: "Set Voltage (V)\n (Kikusui)" -> [_ w435]
          tunnel: "Set Current (mA)\n (Kikusui)" -> [_ w433]
          frame False {
            w423 = 0.0 ("element")
            n240 = Get Date/Time In Seconds() -> (seconds since 1Jan1904=w425:timestamp)
            n241 = local read "AO task out"() -> (w431:refnum<k21>)
            n242 = Build Array (concatenate)(w422, w423) -> (w421:dbl[])
            n243 = Build Array (concatenate)(w426, w425) -> (w424:timestamp[])
            n244 = Build Array(w423, w423) -> (w429:dbl[])
            n245 = call <vilib>:"DAQmx Write (Analog 1D DBL NChan 1Samp).vi"("task/channels in"=w431, "data"=w429, "timeout"=100.0, "error in"=errorcluster {"status"=FALSE, "code"=0, "source"=""}) -> ("task out"=w432:refnum<k21>, "error out"=w427:errorcluster)  [unwired: 9 in, 1 out]
            n246 = local write "AO task out"(w432) -> ()
            n247 = local write "error out (KIKUSI CTRL)"(w427) -> ()
          }
          frame True {
            (unwired) 2.0 ("y")
            n248 = xnode "Formula"("X1"=w433) -> ("Result"=w439:dbl)  [unwired: 1 in, 1 out]
            n249 = Divide(x=w435, y=650.0) -> (x/y=w457:dbl)
            n250 = Multiply(x=10.0 ("y"), y=w457) -> (x*y=w437:dbl)
            n251 = In Range and Coerce(upper limit=0.4, x=w439, lower limit=0.0 ("y")) -> (coerced(x)=w436:dbl, In Range?=w438:bool)
            n252 = case shown="True" w438 {
              tunnel: w437 -> [w464 w467]
              tunnel: w436 -> [_ w466]
              tunnel: [w462 w465] -> w434
              frame False {
                n253 = Build Array(w464, 0.0 ("element")) -> (w462:dbl[])
              }
              frame True {
                n254 = Build Array(w467, w466) -> (w465:dbl[])
              }
            }
            "USB AOUT" <- w434
            n255 = local read "File Refn USB AO"() -> (w451:refnum<file>)
            n256 = Get Date/Time In Seconds() -> (seconds since 1Jan1904=w446:timestamp)
            n257 = Initialize Array("%.3f", 2 ("dimension size")) -> (w452:string[])
            n258 = local read "AO task out"() -> (w459:refnum<k21>)
            n259 = call "FileWrite.vi"("DataArray"=w434, "Time Stamp"=w446, "Error In"=errorcluster {"status"=FALSE, "code"=0, "source"=""} ("error in"), "FileFormat"=w452, "Index"=w450, "refnum in"=w451) -> ("Error Out"=w448:errorcluster, "Byte Stream File Refnum"=w447:refnum<file>)  [unwired: 4 in]
            n260 = Build Array (concatenate)(w445, w446) -> (w442:timestamp[])
            n261 = local write "File Refn USB AO"(w447) -> ()
            n262 = call <vilib>:"DAQmx Write (Analog 1D DBL NChan 1Samp).vi"("task/channels in"=w459, "data"=w434, "timeout"=100.0, "error in"=w448) -> ("task out"=w460:refnum<k21>, "error out"=→"error out (KIKUSI CTRL)":errorcluster)  [unwired: 9 in, 1 out]
            n263 = local write "AO task out"(w460) -> ()
            n264 = Build Array (concatenate)(w444, w433) -> (w443:dbl[])
          }
        }
        n265 = local read "All Labels (USB6218)"() -> (w411:string[])
        n266 = local read "DataArrayConv (USB6218)"() -> (w410:dbl[][])
        n267 = local read "Last Data \n(USB6218)"() -> (w406:dbl[])
        n268 = local read "TimeArray (USB6218)"() -> (w408:timestamp[])
        n269 = Search 1D Array(1D array=w411, element="I_CV") -> (index of element=w412:i32)  [unwired: 1 in]
        n270 = Index Array(array=w410, index (row)=w412) -> (element=w409:dbl[])  [unwired: 1 in]
        n271 = Index Array(array=w406, index=w412) -> (element=→"Monitor Current (mA)":dbl)
        n272 = Bundle("TimeArray (USB6218)"=w408, "DataArrayConv (USB6218)"=w409) -> (w404:T16)  [unwired: 1 in]
      }
      event "upper limit (mA)\n (Kikusui)", "upper limit (V)\n (Kikusui)", "lower limit (mA) \n(Kikusui)", "lower limit (V) \n(Kikusui)": Value Change {
        n273 = event-data() -> ()  [unwired: 1 in, 6 out]
        n274 = property on="Set Current (mA)\n (Kikusui)" class="DigNum (strict)"("Maximum"="upper limit (mA)\n (Kikusui)", "Minimum"="lower limit (mA) \n(Kikusui)") -> ()  [unwired: 2 in, 2 out]
        n275 = property on="Set Voltage (V)\n (Kikusui)" class="DigNum (strict)"("Maximum"="upper limit (V)\n (Kikusui)", "Minimum"="lower limit (V) \n(Kikusui)") -> ()  [unwired: 2 in, 2 out]
      }
      event "OUTPUT\n(Kikusui)": Value Change {
        n276 = event-data() -> ()  [unwired: 1 in, 6 out]
        n277 = local read "Cycle #"() -> (w486:u32)
        n278 = Greater?(x=w486, y=u32 0) -> (0:w484:bool)
        n279 = case shown="True" w484 {
          tunnel: w483 -> [_ w490]
          frame False {
          }
          frame True {
            n280 = property on="V1 (N.O.)" class="Bool (strict)"() -> ("Value"=w501:bool)  [unwired: 2 in, 2 out]
            n281 = Not(x=w501) -> (.not. x?=w500:bool)
            n282 = local read "error out (USB6210/6218 DOUT)"() -> (w504:errorcluster)
            n283 = property on="V2 (N.C.)" class="Bool (strict)"() -> ("Value"=w499:bool)  [unwired: 2 in, 2 out]
            n284 = local read "DOUT task out"() -> (w505:refnum<k21>)
            n285 = Build Array(w500, w499, "OUTPUT\n(Kikusui)") -> (w488:bool[])
            n286 = local read "File Refn USB DO"() -> (w491:refnum<file>)
            n287 = Boolean To (0,1)(Boolean=w488) -> (0, 1=w487:i16[])
            n288 = Initialize Array("%d" ("element"), 3 ("dimension size")) -> (w493:string[])
            n289 = call <vilib>:"DAQmx Write (Digital 1D Bool NChan 1Samp 1Line).vi"("task/channels in"=w505, "data"=w488, "timeout"=10.0, "error in"=w504) -> ("task out"=w502:refnum<k21>, "error out"=w495:errorcluster)  [unwired: 9 in, 1 out]
            n290 = local write "DOUT task out"(w502) -> ()
            n291 = Get Date/Time In Seconds() -> (seconds since 1Jan1904=w492:timestamp)
            n292 = call "FileWrite.vi"("DataArray"=w487, "Time Stamp"=w492, "Error In"=w495, "FileFormat"=w493, "Index"=w490, "refnum in"=w491) -> ("Error Out"=w494:errorcluster, "Byte Stream File Refnum"=w489:refnum<file>)  [unwired: 4 in]
            n293 = local write "File Refn USB DO"(w489) -> ()
            n294 = local write "error out (USB6210/6218 DOUT)"(w494) -> ()
          }
        }
      }
    }
    n295 = Bundle(w337, w334) -> (w336:cluster{timestamp[], dbl[]})  [unwired: 1 in]
    n296 = Build Array(w336, w333) -> (→"Graph 7":T9)
  }
  n297 = while {
    shift-right: [w597] -> w24
    shift-left: refnum<class "USBData.lvclass"> refnum ("USBData.lvclass") -> [w601]
    shift-right: [w593] -> w23
    shift-left: errorcluster {"status"=FALSE, "code"=0, "source"=""} ("error in (no error)") -> [w600]
    tunnel: "RUN identifier" -> [w536]
    tunnel: "Base Path" -> [w535]
    shift-right: [w575] -> w17
    shift-left: errorcluster {"status"=FALSE, "code"=0, "source"=""} ("error in (no error)") -> [w591]
    shift-right: [w576] -> w18
    shift-left: refnum<class "LSI218Data.lvclass"> refnum ("LSI218Data.lvclass") -> [w590]
    shift-right: [w563] -> w14
    shift-left: refnum<class "LSI336Data.lvclass"> refnum ("LSI336Data.lvclass") -> [w572]
    shift-right: [w562] -> w13
    shift-left: w3 -> [w571]
    shift-right: [w551] -> _
    shift-left: errorcluster {"status"=FALSE, "code"=0, "source"=""} ("error in") -> [w552]
    shift-right: [w541] -> w7
    shift-left: refnum<class "USBData.lvclass"> refnum ("USBData.lvclass") -> [w549]
    shift-right: [w540] -> w6
    shift-left: errorcluster {"status"=FALSE, "code"=0, "source"=""} ("error in (no error)") -> [w548]
    shift-right: [w534] -> _
    shift-left: w3 -> [w533]
    i -> [w510]
    stop <- "Stop Button" stop-if-true
    w558 = u32 24 ("Number of Rows")
    w568 = T18 [] ("appended array")
    w585 = T18 [] ("appended array")
    n298 = control-ref of="Plot selecter LSI218(2)\n    1      2     3     4"() -> (w556:refnum<vi>)
    n299 = control-ref of="Plot selecter LSI218(1)\n    1      2     3     4"() -> (w557:refnum<vi>)
    n300 = control-ref of="Plot selecter LSI336 \n     1      2     3     4"() -> (w555:refnum<vi>)
    n301 = local read "Last Data \nLSI336"() -> (w518:dbl[])
    n302 = local read "LSI336Settings(X,Y)"() -> (w523:T3)
    n303 = Equal?(x=w510, y=0) -> (x = y?=w537:bool)
    n304 = local read "LastData (LSI218)"() -> (w519:dbl[])
    n305 = local read "LSI218Settings(A-F)"() -> (w525:T3)
    n306 = And(x="Analog Out ON?", y=w537) -> (x .and. y?=w538:bool)
    n307 = property on="Property Node" class="Arr (strict)"(reference=w557, "Number of Rows"=w558) -> ()  [unwired: 1 in, 2 out]
    n308 = property on="Property Node" class="Arr (strict)"(reference=w556, "Number of Rows"=w558) -> ()  [unwired: 1 in, 2 out]
    n309 = case shown="True" w537 {
      tunnel: [w1492 w1504] -> w562
      tunnel: [w1482 w1503] -> w570
      tunnel: [w1491 w1502] -> w563
      tunnel: [w1490 timestamp[] [] ("TimeArray")] -> w529
      tunnel: [w1489 dbl[][] [] ("DataArray")] -> w527
      tunnel: w572 -> [w1488 w1499]
      tunnel: w571 -> [w1487 w1498]
      tunnel: w536 -> [_ w1496]
      tunnel: w510 -> [w1483 _]
      tunnel: w535 -> [_ w1493]
      frame False {
        n310 = local read "Record interval"() -> (w1480:i64)
        n311 = call-dynamic "LSI336Data_measure.vi"("LSI336Data in"=w1488, "MeasurementIndex"=w1483, "error in (no error)"=w1487, "save every ... measurements"=w1480) -> ("Active?"=→"Active?\n(LSI336)":bool[], "TimeMeasuremeent"=→"Time of Last Measurement (LSI336)":timestamp, "LSI336Data out"=w1491:refnum<class "LSI336Data.lvclass">, "LastData"=→"Last Data \nLSI336":dbl[], "LastMeasurementConfig"=→"LastMeasurementConfig (336)":T11, "DataArray"=w1489:dbl[][], "Status"=w1482:u16, "TimeArray"=w1490:timestamp[], "error out"=w1492:errorcluster)  [unwired: 3 in]
      }
      frame True {
        n312 = Get Date/Time In Seconds() -> (seconds since 1Jan1904=w1505:timestamp)
        n313 = call-dynamic "LSI336Data_initialize.vi"("LSI336Data in"=w1499, "RunName"=w1496, "InstName"="InstName (LSI336)", "FileFormat"="FileFormat (336)", "LSI336Settings(X, Y)"="LSI336Settings(X,Y)", "RUN start time"=w1505, "error in (no error)"=w1498, "base path"=w1493) -> ("LSI336Data out"=w1502:refnum<class "LSI336Data.lvclass">, "Status"=w1503:T7, "AllLabels"=→"Labels LSI336":string[], "error out"=w1504:errorcluster)  [unwired: 4 in]
      }
    }
    "LSI336 Status" <- w570
    "error out (LSI336)" <- w562
    "TimeArray (LSI336)" <- w529
    "DataArray (336)" <- w527
    n314 = case shown="False" w537 {
      tunnel: w601 -> [w1639 w1663]
      tunnel: w600 -> [w1633 w1661]
      tunnel: w510 -> [w1624 _]
      tunnel: [w1631 w1658] -> w593
      tunnel: [w1628 w1657] -> w550
      tunnel: [w1629 w1656] -> w597
      tunnel: [w1619 w1651] -> w598
      tunnel: w536 -> [_ w1649]
      tunnel: w535 -> [_ w1648]
      tunnel: [w1618 w1645] -> w530
      frame False {
        n315 = call-dynamic "USBData_measure.vi"("USBData in"=w1639, "DAQ sample #"=i64 5, "DAQ timeout"=100.0 ("DAQ timeout (def: 100)"), "MeasurementIndex"=w1624, "error in (no error)"=w1633, "save every ... measurements"="Record interval") -> ("USBData out"=w1638:refnum<class "USBData.lvclass">, "TimeMeasuremeent"=w1635:timestamp, "Status"=→"USB6210 Status":T6, "LastDataAcquired"=w1620:dbl[], "error out"=w1634:errorcluster)  [unwired: 3 in, 2 out]
        "Time of Last Measurement (USB6210)" <- w1635
        "Last Vol\n(USB6210)" <- w1620
        n316 = call-dynamic "USBData_convert.vi"("Save every ... measurements"="Record interval", "MeasurementIndex"=w1624, "error in (no error)"=w1634, "LastDataAcquired"=w1620, "TimeMeasuremeent"=w1635, "USBData in"=w1638) -> ("error out"=w1632:errorcluster, "LeakDet_FULL"=w1627:dbl, "LastDataConverted"=w1621:dbl[], "USBData out"=w1630:refnum<class "USBData.lvclass">)  [unwired: 2 in]
        n317 = call "USBData_read.vi"("USBData in"=w1630, "error in (no error)"=w1632) -> ("Status"=w1622:T6, "USBData out"=w1629:refnum<class "USBData.lvclass">, "Data"=w1628:T19, "Basic"=w1619:T20, "error out"=w1631:errorcluster)  [unwired: 2 in, 2 out]
        n318 = local write "USB6210 Status"(w1622) -> ()
        n319 = Unbundle By Name(w1619) -> ("ReadLeakDet?"=w1626:bool)
        n320 = Unbundle By Name(w1619) -> ("Labels"=w1618:string[])
        n321 = case shown="False" w1626 {
          tunnel: w1621 -> [w1640 w1643]
          tunnel: w1627 -> [_ w1642]
          tunnel: [w1640 w1641] -> w1625
          frame False {
          }
          frame True {
            n322 = Build Array (concatenate)(w1643, w1642) -> (w1641:dbl[])
          }
        }
        "Last Data \n(USB6210)" <- w1625
      }
      frame True {
        n323 = Get Date/Time In Seconds() -> (seconds since 1Jan1904=w1650:timestamp)
        n324 = call-dynamic "USBData_initialize.vi"("USBData in"=w1663, "SeriesSetting"="USB6210 Config", "BasePath"=w1648, "RunName"=w1649, "FileName"="InstName (USB6210)", "error in (no error)"=w1661, "RUN start time"=w1650) -> ("Status"=w1644:T6, "USBData out"=w1659:refnum<class "USBData.lvclass">, "error out"=w1660:errorcluster)  [unwired: 4 in, 2 out]
        n325 = local write "USB6210 Status"(w1644) -> ()
        n326 = call "USBData_read.vi"("USBData in"=w1659, "error in (no error)"=w1660) -> ("Status"=w1647:T6, "USBData out"=w1656:refnum<class "USBData.lvclass">, "Data"=w1657:T19, "Basic"=w1651:T20, "error out"=w1658:errorcluster)  [unwired: 2 in, 2 out]
        n327 = local write "USB6210 Status"(w1647) -> ()
        n328 = Unbundle By Name(w1651) -> ("ReadLeakDet?"=w1655:bool, "Labels"=w1645:string[])
        n329 = Array Size(array=w1645) -> (size(s)=w1654:i32)
        n330 = case shown="True" w1655 {
          tunnel: w1654 -> [w1664 w1666]
          tunnel: [w1664 w1665] -> w1652
          frame False {
          }
          frame True {
            n331 = Add(x=w1666, y=1) -> (x+y=w1665:i32)
          }
        }
        n332 = Initialize Array(TRUE ("Activate 2"), w1652) -> ()  [unwired: 1 out]
      }
    }
    "error out (USB6210)" <- w593
    n333 = case shown="False" w537 {
      tunnel: [w1169 w1197] -> w540
      tunnel: [w1166 w1196] -> w547
      tunnel: [w1167 w1195] -> w541
      tunnel: [w1158 w1190] -> w546
      tunnel: [w1157 w1187] -> _
      tunnel: w549 -> [w1156 w1185]
      tunnel: w535 -> [_ w1184]
      tunnel: w536 -> [_ w1183]
      tunnel: w548 -> [w1155 w1182]
      tunnel: w510 -> [w1154 _]
      frame False {
        n334 = local read "Record interval"() -> (w1153:i64)
        n335 = call-dynamic "USBData_measure.vi"("USBData in"=w1156, "DAQ sample #"=i64 5, "DAQ timeout"=100.0 ("DAQ timeout (def: 100)"), "MeasurementIndex"=w1154, "error in (no error)"=w1155, "save every ... measurements"=w1153) -> ("USBData out"=w1175:refnum<class "USBData.lvclass">, "TimeMeasuremeent"=w1172:timestamp, "Status"=→"USB6218 Status":T6, "LastDataAcquired"=w1159:dbl[], "error out"=w1171:errorcluster)  [unwired: 3 in, 2 out]
        "Time of Last Measurement (USB6218)" <- w1172
        "Last Vol \n(USB6218)" <- w1159
        n336 = call-dynamic "USBData_convert.vi"("Save every ... measurements"=w1153, "MeasurementIndex"=w1154, "error in (no error)"=w1171, "LastDataAcquired"=w1159, "TimeMeasuremeent"=w1172, "USBData in"=w1175) -> ("error out"=w1170:errorcluster, "LeakDet_FULL"=w1165:dbl, "LastDataConverted"=w1160:dbl[], "USBData out"=w1168:refnum<class "USBData.lvclass">)  [unwired: 2 in]
        n337 = call "USBData_read.vi"("USBData in"=w1168, "error in (no error)"=w1170) -> ("Status"=w1161:T6, "USBData out"=w1167:refnum<class "USBData.lvclass">, "Data"=w1166:T19, "Basic"=w1158:T20, "error out"=w1169:errorcluster)  [unwired: 2 in, 2 out]
        n338 = local write "USB6218 Status"(w1161) -> ()
        n339 = Unbundle By Name(w1158) -> ("ReadLeakDet?"=w1164:bool)
        n340 = Unbundle By Name(w1158) -> ("Labels"=w1157:string[])
        n341 = case shown="True" w1164 {
          tunnel: w1160 -> [w1176 w1179]
          tunnel: w1165 -> [_ w1178]
          tunnel: [w1176 w1177] -> w1163
          frame False {
          }
          frame True {
            n342 = Build Array (concatenate)(w1179, w1178) -> (w1177:dbl[])
          }
        }
        "Last Data \n(USB6218)" <- w1163
      }
      frame True {
        n343 = Get Date/Time In Seconds() -> (seconds since 1Jan1904=w1189:timestamp)
        n344 = call-dynamic "USBData_initialize.vi"("USBData in"=w1185, "SeriesSetting"="USB6218 Config", "BasePath"=w1184, "RunName"=w1183, "FileName"="InstName (USB6218)", "error in (no error)"=w1182, "RUN start time"=w1189) -> ("Status"=w1180:T6, "USBData out"=w1198:refnum<class "USBData.lvclass">, "error out"=w1199:errorcluster)  [unwired: 4 in, 2 out]
        n345 = local write "USB6218 Status"(w1180) -> ()
        n346 = call "USBData_read.vi"("USBData in"=w1198, "error in (no error)"=w1199) -> ("Status"=w1188:T6, "USBData out"=w1195:refnum<class "USBData.lvclass">, "Data"=w1196:T19, "Basic"=w1190:T20, "error out"=w1197:errorcluster)  [unwired: 2 in, 2 out]
        n347 = local write "USB6218 Status"(w1188) -> ()
        n348 = Unbundle By Name(w1190) -> ("ReadLeakDet?"=w1194:bool, "Labels"=w1187:string[])
        n349 = Array Size(array=w1187) -> (size(s)=w1193:i32)
        n350 = case shown="True" w1194 {
          tunnel: w1193 -> [w1200 w1202]
          tunnel: [w1200 w1201] -> w1191
          frame False {
          }
          frame True {
            n351 = Add(x=w1202, y=1) -> (x+y=w1201:i32)
          }
        }
        n352 = Initialize Array(TRUE ("Activate 2"), w1191) -> ()  [unwired: 1 out]
      }
    }
    "error out (USB6218)" <- w540
    n353 = case shown="False" w537 {
      tunnel: [w1598 w1613] -> w575
      tunnel: [w1593 w1612] -> w592
      tunnel: [w1596 w1611] -> w576
      tunnel: w510 -> [w1597 _]
      tunnel: w591 -> [w1587 w1606]
      tunnel: w590 -> [w1588 w1605]
      tunnel: w536 -> [_ w1604]
      tunnel: w535 -> [_ w1603]
      tunnel: [w1585 timestamp[] [] ("TimeArray")] -> w589
      tunnel: [w1584 dbl[][] [] ("DataArray")] -> w588
      frame False {
        w1591 = 24 ("index")
        n354 = local read "Record interval"() -> (w1582:i64)
        n355 = call-dynamic "LSI218Data_measure.vi"("LSI218Data in"=w1588, "MeasurementIndex"=w1597, "error in (no error)"=w1587, "save every ... measurements"=w1582) -> ("TimeMeasuremeent"=→"Time of Last Measurement (LSI218)":timestamp, "Active?"=w1592:bool[], "LSI218Data out"=w1596:refnum<class "LSI218Data.lvclass">, "LastMeasurementConfig"=→"LastMeasurementConfig (218)":T11, "LastData"=w1586:dbl[], "Status"=w1593:u16, "TimeArray"=w1585:timestamp[], "DataArray"=w1584:dbl[][], "error out"=w1598:errorcluster)  [unwired: 3 in]
        "LastData (LSI218)" <- w1586
        n356 = Split 1D Array(array=w1592, index=w1591) -> (first subarray=→"Active?\n (1)":bool[], second subarray=→"Active?\n(2)":bool[])
        n357 = Split 1D Array(array=w1586, index=w1591) -> (first subarray=→"Last Data \nLSI218 (1)":dbl[], second subarray=→"Last Data \nLSI218 (2)":dbl[])
      }
      frame True {
        n358 = Get Date/Time In Seconds() -> (seconds since 1Jan1904=w1614:timestamp)
        n359 = call-dynamic "LSI218Data_initialize.vi"("LSI218Settings(A-F)"="LSI218Settings(A-F)", "FileFormat"="FileFormat (218)", "RUN start time"=w1614, "base path"=w1603, "error in (no error)"=w1606, "InstName"="InstName (LSI218)", "RunName"=w1604, "LSI218Data in"=w1605) -> ("error out"=w1613:errorcluster, "Status"=w1612:T7, "AllLabels"=w1602:string[], "LSI218Data out"=w1611:refnum<class "LSI218Data.lvclass">)
        n360 = Split 1D Array(array=w1602, index=24) -> (first subarray=→"Labels LSI218 (1)":string[], second subarray=→"Labels LSI218 (2)":string[])
      }
    }
    "LSI218 Status" <- w592
    "error out (LSI218)" <- w575
    n361 = property on="Property Node" class="Arr (strict)"(reference=w555, "Number of Rows"=u32 8) -> ()  [unwired: 1 in, 2 out]
    n362 = Array Size(array=w525) -> (size(s)=w524:i32)
    n363 = Multiply(x="Measurement Interval (s)", y=u32 1000) -> (x*y=w594:dbl)
    n364 = for {
      tunnel: w523 -> [w607] mode=indexing
      tunnel: [w606] -> w522 mode=concatenating
      n365 = Unbundle By Name(w607) -> ("SensorLocations"=w606:T12)
    }
    n366 = for {
      N: w524 -> [_]
      tunnel: w525 -> [w609] mode=indexing
      tunnel: [w608] -> w521 mode=concatenating
      n367 = Unbundle By Name(w609) -> ("SensorLocations"=w608:T12)
    }
    n368 = Wait (ms)(milliseconds to wait=w594) -> ()  [unwired: 1 out]
    n369 = Quotient & Remainder(x=w510, y="Screenshots interval") -> (x-y*floor(x/y)=w508:i64)  [unwired: 1 out]
    n370 = Equal?(x=w508, y=i64 0) -> (x = y?=w506:bool)
    n371 = case shown="True" w506 {
      frame False {
      }
      frame True {
        n372 = flat-sequence {
          frame #0 {
            n373 = property on="Frontpanel screenshots" class="Bool (strict)"("Val(Sgnl)"=TRUE ("Value (Signaling)")) -> ()  [unwired: 2 in, 2 out]
          }
          frame #1 {
            n374 = Wait (ms)(milliseconds to wait=u32 500) -> ()  [unwired: 1 out]
          }
          frame #2 {
            n375 = property on="Frontpanel screenshots" class="Bool (strict)"("Val(Sgnl)"=FALSE ("Value (Signaling)")) -> ()  [unwired: 2 in, 2 out]
          }
        }
      }
    }
    n376 = Build Array (concatenate)(w519, w518) -> (w517:dbl[])
    "AllTemperatures" <- w517
    n377 = Build Array (concatenate)(w521, w522) -> (w520:T12)
    "TempSensorsLocations" <- w520
    n378 = case shown="True" w538 {
      tunnel: w535 -> [_ w969]
      tunnel: w536 -> [_ w968]
      tunnel: [w954 w956] -> w534
      tunnel: w533 -> [w954 w955]
      frame False {
      }
      frame True {
        w967 = "_"
        w977 = 10.0 ("V_lim_max")
        w976 = 0.0 ("V_lim_min")
        w975 = -1 items=["Default"=-1, "RSE"=10083, "Differential"=10106, "Pseudodifferential"=12529] ("output terminal configuration")
        w974 = 10348 items=["Volts"=10348, "From Custom Scale"=10065] ("units")
        n379 = Get Date/Time In Seconds() -> (seconds since 1Jan1904=w972:timestamp)
        n380 = call "LV_UNIXTIME.vi"("current time"=w972) -> ("date/time string"=w965:string)  [unwired: 9 in, 1 out]
        n381 = Concatenate Strings(w965, "_AO" ("string")) -> (w979:string)
        n382 = Concatenate Strings(w968, w967, w965, w967, "USB_AOUT.csv" ("string")) -> (w970:string)
        n383 = Build Path(base path=w969, name or relative path=w970) -> (appended path=w964:path)
        n384 = Open/Create/Replace File(file path (use dialog)=w964, operation (0:open)=T17."open or create") -> (refnum out=w962:refnum<file>)  [unwired: 4 in, 2 out]
        n385 = Build Array("AOUT 0 Label", "AOUT 1 Label") -> (w958:string[])
        n386 = call "FileIntialize.vi"("Error In"=w955, "Labels"=w958, "refnum in"=w962) -> ("Error Out"=w957:errorcluster, "File Refnum"=→"File Refn USB AO":refnum<file>)  [unwired: 7 in]
        n387 = call <vilib>:"DAQmx Create Task.vi"("new task name"=w979, "auto cleanup"=FALSE, "error in"=w957) -> ("task out"=w978:refnum<k21>, "error out"=w980:errorcluster)  [unwired: 11 in]
        n388 = call-poly <vilib>:"DAQmx Create Virtual Channel.vi"("task in"=w978, "maximum value"=w977, "minimum value"=w976, "output terminal configuration"=w975, "physical channels"="AOUT For Voltage CTRL", "units"=w974, "error in"=w980) -> ("task out"=w982:refnum<k21>, "error out"=w983:errorcluster)  [unwired: 7 in]
        n389 = call-poly <vilib>:"DAQmx Create Virtual Channel.vi"("task in"=w982, "maximum value"=w977, "minimum value"=w976, "physical channels"="AOUT for Current CTRL", "error in"=w983) -> ("task out"=w985:refnum<k21>, "error out"=w984:errorcluster)  [unwired: 9 in]
        n390 = call <vilib>:"DAQmx Start Task.vi"("task/channels in"=w985, "error in"=w984) -> ("task out"=→"AO task out":refnum<k21>, "error out"=w956:errorcluster)  [unwired: 12 in]
      }
    }
    "error out (USB6210/6218 AOUT)" <- w534
    n391 = local read "All Labels (USB6218)"() -> (w515:string[])
    n392 = local read "Last Data \n(USB6218)"() -> (w514:dbl[])
    n393 = local read "All Labels (USB6210)"() -> (w516:string[])
    n394 = local read "Last Data \n(USB6210)"() -> (w513:dbl[])
    n395 = flat-sequence {
      tunnel: w517 -> [w610]
      tunnel: w520 -> [w611]
      tunnel: w512 -> [w863]
      tunnel: w511 -> [w862]
      frame #0 {
        n396 = stacked-sequence {
          tunnel: w611 -> [w616 w621 w626 w631 w636 w641 w646 w651 w656 w661 w666 w671 w676 w681 w686 w691 w696 w701 w706 w711 w716 w721 w726 w731 w736 w741 w746 w751 w756 w761 w766 w771 w776 w781 w786 w791 w796 w801 w806 w811 w816 w821 w826 w831 w836 w841 w846 w851 w856 w861]
          tunnel: w610 -> [w614 w619 w624 w629 w634 w639 w644 w649 w654 w659 w664 w669 w674 w679 w684 w689 w694 w699 w704 w709 w714 w719 w724 w729 w734 w739 w744 w749 w754 w759 w764 w769 w774 w779 w784 w789 w794 w799 w804 w809 w814 w819 w824 w829 w834 w839 w844 w849 w854 w859]
          frame #0 {
            n397 = Search 1D Array(1D array=w616, element=T10."T3He1-1" ("SensorLocations")) -> (index of element=w613:i32)  [unwired: 1 in]
            n398 = Index Array(array=w614, index=w613) -> (element=→"T3He1-1":dbl)
          }
          frame #1 {
            n399 = Search 1D Array(1D array=w621, element=T10."T3He1-2" ("SensorLocations")) -> (index of element=w618:i32)  [unwired: 1 in]
            n400 = Index Array(array=w619, index=w618) -> (element=→"T3He1-2":dbl)
          }
          frame #2 {
            n401 = Search 1D Array(1D array=w626, element=T10."T3He1-3" ("SensorLocations")) -> (index of element=w623:i32)  [unwired: 1 in]
            n402 = Index Array(array=w624, index=w623) -> (element=→"T3He1-3":dbl)
          }
          frame #3 {
            n403 = Search 1D Array(1D array=w631, element=T10."T3He1-4" ("SensorLocations")) -> (index of element=w628:i32)  [unwired: 1 in]
            n404 = Index Array(array=w629, index=w628) -> (element=→"T3He1-4":dbl)
          }
          frame #4 {
            n405 = Search 1D Array(1D array=w636, element=T10."T3He2-1" ("SensorLocations")) -> (index of element=w633:i32)  [unwired: 1 in]
            n406 = Index Array(array=w634, index=w633) -> (element=→"T3He2-1":dbl)
          }
          frame #5 {
            n407 = Search 1D Array(1D array=w641, element=T10."T3He2-2" ("SensorLocations")) -> (index of element=w638:i32)  [unwired: 1 in]
            n408 = Index Array(array=w639, index=w638) -> (element=→"T3He2-2":dbl)
          }
          frame #6 {
            n409 = Search 1D Array(1D array=w646, element=T10."T3He3" ("SensorLocations")) -> (index of element=w643:i32)  [unwired: 1 in]
            n410 = Index Array(array=w644, index=w643) -> (element=→"T3He3":dbl)
          }
          frame #7 {
            n411 = Search 1D Array(1D array=w651, element=T10."T3He4" ("SensorLocations")) -> (index of element=w648:i32)  [unwired: 1 in]
            n412 = Index Array(array=w649, index=w648) -> (element=→"T3He4":dbl)
          }
          frame #8 {
            n413 = Search 1D Array(1D array=w656, element=T10."T3He5" ("SensorLocations")) -> (index of element=w653:i32)  [unwired: 1 in]
            n414 = Index Array(array=w654, index=w653) -> (element=→"T3He5":dbl)
          }
          frame #9 {
            n415 = Search 1D Array(1D array=w661, element=T10."T3He6-1" ("SensorLocations")) -> (index of element=w658:i32)  [unwired: 1 in]
            n416 = Index Array(array=w659, index=w658) -> (element=→"T3He6-1" →"T3He6-1/6-2 (HEX1)":dbl)
          }
          frame #10 {
            n417 = Search 1D Array(1D array=w666, element=T10."T3He6-2" ("SensorLocations")) -> (index of element=w663:i32)  [unwired: 1 in]
            n418 = Index Array(array=w664, index=w663) -> (element=→"T3He6-2" →"T3He6-1/6-2 (3He pot) 2":dbl)
          }
          frame #11 {
            n419 = Search 1D Array(1D array=w671, element=T10."T3He7-1" ("SensorLocations")) -> (index of element=w668:i32)  [unwired: 1 in]
            n420 = Index Array(array=w669, index=w668) -> (element=→"T3He7-1" →"T3He7-1/7-2 (HEX1)":dbl)
          }
          frame #12 {
            n421 = Search 1D Array(1D array=w676, element=T10."T3He7-2" ("SensorLocations")) -> (index of element=w673:i32)  [unwired: 1 in]
            n422 = Index Array(array=w674, index=w673) -> (element=→"T3He7-2" →"T3He7-1/6-2 (3He pot) 2":dbl)
          }
          frame #13 {
            n423 = Search 1D Array(1D array=w681, element=T10."T3He8" ("SensorLocations")) -> (index of element=w678:i32)  [unwired: 1 in]
            n424 = Index Array(array=w679, index=w678) -> (element=→"T3He8":dbl)
          }
          frame #14 {
            n425 = Search 1D Array(1D array=w686, element=T10."T3He9" ("SensorLocations")) -> (index of element=w683:i32)  [unwired: 1 in]
            n426 = Index Array(array=w684, index=w683) -> (element=→"T3He9":dbl)
          }
          frame #15 {
            n427 = Search 1D Array(1D array=w691, element=T10."T3He10" ("SensorLocations")) -> (index of element=w688:i32)  [unwired: 1 in]
            n428 = Index Array(array=w689, index=w688) -> (element=→"T3He10":dbl)
          }
          frame #16 {
            n429 = Search 1D Array(1D array=w696, element=T10."T4He1" ("SensorLocations")) -> (index of element=w693:i32)  [unwired: 1 in]
            n430 = Index Array(array=w694, index=w693) -> (element=→"T4He1" →"T4He1 (4K reservoir )":dbl)
          }
          frame #17 {
            n431 = Search 1D Array(1D array=w701, element=T10."T4He2-1" ("SensorLocations")) -> (index of element=w698:i32)  [unwired: 1 in]
            n432 = Index Array(array=w699, index=w698) -> (element=→"T4He2-1":dbl)
          }
          frame #18 {
            n433 = Search 1D Array(1D array=w706, element=T10."T4He2-2" ("SensorLocations")) -> (index of element=w703:i32)  [unwired: 1 in]
            n434 = Index Array(array=w704, index=w703) -> (element=→"T4He2-2":dbl)
          }
          frame #19 {
            n435 = Search 1D Array(1D array=w711, element=T10."T4He3-1" ("SensorLocations")) -> (index of element=w708:i32)  [unwired: 1 in]
            n436 = Index Array(array=w709, index=w708) -> (element=→"T4He3-1":dbl)
          }
          frame #20 {
            n437 = Search 1D Array(1D array=w716, element=T10."T4He3-2" ("SensorLocations")) -> (index of element=w713:i32)  [unwired: 1 in]
            n438 = Index Array(array=w714, index=w713) -> (element=→"T4He3-2":dbl)
          }
          frame #21 {
            n439 = Search 1D Array(1D array=w721, element=T10."T4He3-3" ("SensorLocations")) -> (index of element=w718:i32)  [unwired: 1 in]
            n440 = Index Array(array=w719, index=w718) -> (element=→"T4He3-3":dbl)
          }
          frame #22 {
            n441 = Search 1D Array(1D array=w726, element=T10."T4He3-4" ("SensorLocations")) -> (index of element=w723:i32)  [unwired: 1 in]
            n442 = Index Array(array=w724, index=w723) -> (element=→"T4He3-4":dbl)
          }
          frame #23 {
            n443 = Search 1D Array(1D array=w731, element=T10."T4He4" ("SensorLocations")) -> (index of element=w728:i32)  [unwired: 1 in]
            n444 = Index Array(array=w729, index=w728) -> (element=→"T4He4":dbl)
          }
          frame #24 {
            n445 = Search 1D Array(1D array=w736, element=T10."T4He5" ("SensorLocations")) -> (index of element=w733:i32)  [unwired: 1 in]
            n446 = Index Array(array=w734, index=w733) -> (element=→"T4He5":dbl)
          }
          frame #25 {
            n447 = Search 1D Array(1D array=w741, element=T10."T4He6" ("SensorLocations")) -> (index of element=w738:i32)  [unwired: 1 in]
            n448 = Index Array(array=w739, index=w738) -> (element=→"T4He6":dbl)
          }
          frame #26 {
            n449 = Search 1D Array(1D array=w746, element=T10."T4He7" ("SensorLocations")) -> (index of element=w743:i32)  [unwired: 1 in]
            n450 = Index Array(array=w744, index=w743) -> (element=→"T4He7":dbl)
          }
          frame #27 {
            n451 = Search 1D Array(1D array=w751, element=T10."T4He8" ("SensorLocations")) -> (index of element=w748:i32)  [unwired: 1 in]
            n452 = Index Array(array=w749, index=w748) -> (element=→"T4He8":dbl)
          }
          frame #28 {
            n453 = Search 1D Array(1D array=w756, element=T10."T4He9" ("SensorLocations")) -> (index of element=w753:i32)  [unwired: 1 in]
            n454 = Index Array(array=w754, index=w753) -> (element=→"T4He9":dbl)
          }
          frame #29 {
            n455 = Search 1D Array(1D array=w761, element=T10."T4He10" ("SensorLocations")) -> (index of element=w758:i32)  [unwired: 1 in]
            n456 = Index Array(array=w759, index=w758) -> (element=→"T4He10":dbl)
          }
          frame #30 {
            n457 = Search 1D Array(1D array=w766, element=T10."T1K1" ("SensorLocations")) -> (index of element=w763:i32)  [unwired: 1 in]
            n458 = Index Array(array=w764, index=w763) -> (element=→"T1K1":dbl)
          }
          frame #31 {
            n459 = Search 1D Array(1D array=w771, element=T10."T1K2" ("SensorLocations")) -> (index of element=w768:i32)  [unwired: 1 in]
            n460 = Index Array(array=w769, index=w768) -> (element=→"T1K2":dbl)
          }
          frame #32 {
            n461 = Search 1D Array(1D array=w776, element=T10."T1K3-1" ("SensorLocations")) -> (index of element=w773:i32)  [unwired: 1 in]
            n462 = Index Array(array=w774, index=w773) -> (element=→"T1K3-1" →"T1K3-1/3-2 (1K pot)":dbl)
          }
          frame #33 {
            n463 = Search 1D Array(1D array=w781, element=T10."T1K3-2" ("SensorLocations")) -> (index of element=w778:i32)  [unwired: 1 in]
            n464 = Index Array(array=w779, index=w778) -> (element=→"T1K3-2" →"T1K3-1/3-2 (1K pot) 2":dbl)
          }
          frame #34 {
            n465 = Search 1D Array(1D array=w786, element=T10."T1K4" ("SensorLocations")) -> (index of element=w783:i32)  [unwired: 1 in]
            n466 = Index Array(array=w784, index=w783) -> (element=→"T1K4":dbl)
          }
          frame #35 {
            n467 = Search 1D Array(1D array=w791, element=T10."T1K5" ("SensorLocations")) -> (index of element=w788:i32)  [unwired: 1 in]
            n468 = Index Array(array=w789, index=w788) -> (element=→"T1K5":dbl)
          }
          frame #36 {
            n469 = Search 1D Array(1D array=w796, element=T10."T1K6" ("SensorLocations")) -> (index of element=w793:i32)  [unwired: 1 in]
            n470 = Index Array(array=w794, index=w793) -> (element=→"T1K6":dbl)
          }
          frame #37 {
            n471 = Search 1D Array(1D array=w801, element=T10."TIP1" ("SensorLocations")) -> (index of element=w798:i32)  [unwired: 1 in]
            n472 = Index Array(array=w799, index=w798) -> (element=→"TIP1":dbl)
          }
          frame #38 {
            n473 = Search 1D Array(1D array=w806, element=T10."TIP2" ("SensorLocations")) -> (index of element=w803:i32)  [unwired: 1 in]
            n474 = Index Array(array=w804, index=w803) -> (element=→"TIP2":dbl)
          }
          frame #39 {
            n475 = Search 1D Array(1D array=w811, element=T10."TIP3" ("SensorLocations")) -> (index of element=w808:i32)  [unwired: 1 in]
            n476 = Index Array(array=w809, index=w808) -> (element=→"TIP3":dbl)
          }
          frame #40 {
            n477 = Search 1D Array(1D array=w816, element=T10."TIP4" ("SensorLocations")) -> (index of element=w813:i32)  [unwired: 1 in]
            n478 = Index Array(array=w814, index=w813) -> (element=→"TIP4":dbl)
          }
          frame #41 {
            n479 = Search 1D Array(1D array=w821, element=T10."TIP5" ("SensorLocations")) -> (index of element=w818:i32)  [unwired: 1 in]
            n480 = Index Array(array=w819, index=w818) -> (element=→"TIP5":dbl)
          }
          frame #42 {
            n481 = Search 1D Array(1D array=w826, element=T10."TIP6" ("SensorLocations")) -> (index of element=w823:i32)  [unwired: 1 in]
            n482 = Index Array(array=w824, index=w823) -> (element=→"TIP6":dbl)
          }
          frame #43 {
            n483 = Search 1D Array(1D array=w831, element=T10."TIP7" ("SensorLocations")) -> (index of element=w828:i32)  [unwired: 1 in]
            n484 = Index Array(array=w829, index=w828) -> (element=→"TIP7":dbl)
          }
          frame #44 {
            n485 = Search 1D Array(1D array=w836, element=T10."TTH1" ("SensorLocations")) -> (index of element=w833:i32)  [unwired: 1 in]
            n486 = Index Array(array=w834, index=w833) -> (element=→"TTH1":dbl)
          }
          frame #45 {
            n487 = Search 1D Array(1D array=w841, element=T10."TTH2" ("SensorLocations")) -> (index of element=w838:i32)  [unwired: 1 in]
            n488 = Index Array(array=w839, index=w838) -> (element=→"TTH2":dbl)
          }
          frame #46 {
            n489 = Search 1D Array(1D array=w846, element=T10."TTH3" ("SensorLocations")) -> (index of element=w843:i32)  [unwired: 1 in]
            n490 = Index Array(array=w844, index=w843) -> (element=→"TTH3":dbl)
          }
          frame #47 {
            n491 = Search 1D Array(1D array=w851, element=T10."TTH4" ("SensorLocations")) -> (index of element=w848:i32)  [unwired: 1 in]
            n492 = Index Array(array=w849, index=w848) -> (element=→"TTH4":dbl)
          }
          frame #48 {
            n493 = Search 1D Array(1D array=w856, element="SensorLocation 1") -> (index of element=w853:i32)  [unwired: 1 in]
            n494 = Index Array(array=w854, index=w853) -> (element=→"Temperature 1":dbl)
          }
          frame #49 {
            n495 = Search 1D Array(1D array=w861, element="SensorLocation 2") -> (index of element=w858:i32)  [unwired: 1 in]
            n496 = Index Array(array=w859, index=w858) -> (element=→"Temperature 2":dbl)
          }
        }
      }
      frame #1 {
        n497 = stacked-sequence {
          tunnel: w863 -> [w868 w873 w878 w883 w888 w893 w898 w903 w908 w913 w918 w923 w928 w933 w938 w943 w948 w953]
          tunnel: w862 -> [w865 w871 w877 w882 w887 w891 w896 w901 w906 w911 w916 w920 w925 w930 w935 w940 w945 w950]
          frame #0 {
            n498 = Search 1D Array(1D array=w868, element="Insulation vacuum") -> (index of element=w866:i32)  [unwired: 1 in]
            n499 = Index Array(array=w865, index=w866) -> (element=→"P_ins" →"P (insulation)":dbl)
          }
          frame #1 {
            n500 = Search 1D Array(1D array=w873, element="4K reservoir pressure") -> (index of element=w870:i32)  [unwired: 1 in]
            n501 = Index Array(array=w871, index=w870) -> (element=→"P_4Kres" →"P (4K reservoir)":dbl)
          }
          frame #2 {
            n502 = Search 1D Array(1D array=w878, element="3He inlet pressure") -> (index of element=w876:i32)  [unwired: 1 in]
            n503 = Index Array(array=w877, index=w876) -> (element=→"P_3HeIN" →"P (3He IN)":dbl)
          }
          frame #3 {
            n504 = Search 1D Array(1D array=w883, element="Shield return press.") -> (index of element=w881:i32)  [unwired: 1 in]
            n505 = Index Array(array=w882, index=w881) -> (element=→"P_SldRTN" →"P (shield return)":dbl)
          }
          frame #4 {
            n506 = Search 1D Array(1D array=w888, element="3He pot pressure") -> (index of element=w886:i32)  [unwired: 1 in]
            n507 = Index Array(array=w887, index=w886) -> (element=→"P_3Hepot" →"P (3He pot)":dbl)
          }
          frame #5 {
            n508 = Search 1D Array(1D array=w893, element="1Kpot pressure") -> (index of element=w890:i32)  [unwired: 1 in]
            n509 = Index Array(array=w891, index=w890) -> (element=→"P_1Kpot" →"P (1K pot)":dbl)
          }
          frame #6 {
            n510 = Search 1D Array(1D array=w898, element="Dewar pressure") -> (index of element=w895:i32)  [unwired: 1 in]
            n511 = Index Array(array=w896, index=w895) -> (element=→"P_Dewar" →"P (Dewar)":dbl)
          }
          frame #7 {
            n512 = Search 1D Array(1D array=w903, element="Diff pressure HEX4") -> (index of element=w900:i32)  [unwired: 1 in]
            n513 = Index Array(array=w901, index=w900) -> (element=→"DP_HEX4" →"DP HEX4":dbl)
          }
          frame #8 {
            n514 = Search 1D Array(1D array=w908, element="Diff pressure HEX5") -> (index of element=w905:i32)  [unwired: 1 in]
            n515 = Index Array(array=w906, index=w905) -> (element=→"DP_HEX5" →"DP HEX5":dbl)
          }
          frame #9 {
            n516 = Search 1D Array(1D array=w913, element="1K pump exhaust flow") -> (index of element=w910:i32)  [unwired: 1 in]
            n517 = Index Array(array=w911, index=w910) -> (element=→"F_1" →"F1 (1K pump exhaust) flow":dbl)
          }
          frame #10 {
            n518 = Search 1D Array(1D array=w918, element="Shield flow") -> (index of element=w915:i32)  [unwired: 1 in]
            n519 = Index Array(array=w916, index=w915) -> (element=→"F_2" →"F2 (shield flow)":dbl)
          }
          frame #11 {
            n520 = Search 1D Array(1D array=w923, element="4He return flow from HEX7") -> (index of element=w921:i32)  [unwired: 1 in]
            n521 = Index Array(array=w920, index=w921) -> (element=→"F_3" →"F3 (4He rtn flw via HEX7)":dbl)
          }
          frame #12 {
            n522 = Search 1D Array(1D array=w928, element="3He incoming flow into HEX7") -> (index of element=w926:i32)  [unwired: 1 in]
            n523 = Index Array(array=w925, index=w926) -> (element=→"F_4" →"F4 (3He in flow to HEX7)":dbl)
          }
          frame #13 {
            n524 = Search 1D Array(1D array=w933, element="3He pump exhaust flow") -> (index of element=w931:i32)  [unwired: 1 in]
            n525 = Index Array(array=w930, index=w931) -> (element=→"F_5" →"F5 (3He pump ex.)":dbl)
          }
          frame #14 {
            n526 = Search 1D Array(1D array=w938, element="4K reservoir level") -> (index of element=w936:i32)  [unwired: 1 in]
            n527 = Index Array(array=w935, index=w936) -> (element=→"L3" →"He level (4K)":dbl)
          }
          frame #15 {
            n528 = Search 1D Array(1D array=w943, element="1K pot level") -> (index of element=w941:i32)  [unwired: 1 in]
            n529 = Index Array(array=w940, index=w941) -> (element=→"L(1K) (a1)" →"He level (1K)":dbl)
          }
          frame #16 {
            n530 = Search 1D Array(1D array=w948, element="1K pot (b)") -> (index of element=w946:i32)  [unwired: 1 in]
            n531 = Index Array(array=w945, index=w946) -> (element=→"1K pot(b1)" →"He level (1K) b":dbl)
          }
          frame #17 {
            n532 = Search 1D Array(1D array=w953, element="3He pot") -> (index of element=w951:i32)  [unwired: 1 in]
            n533 = Index Array(array=w950, index=w951) -> (element=→"3He pot level" →"He level (3He)":dbl)
          }
        }
      }
    }
    n534 = Build Array (concatenate)(w516, w515) -> (w512:string[])
    n535 = Build Array (concatenate)(w513, w514) -> (w511:dbl[])
    n536 = case shown="True" "Digital Out ON?" {
      tunnel: w537 -> [_ w1211]
      tunnel: w552 -> [w1204 w1210]
      tunnel: [w1204 w1209] -> w551
      tunnel: w550 -> [_ w1208]
      tunnel: w536 -> [_ w1207]
      tunnel: w535 -> [_ w1206]
      tunnel: w530 -> [_ w1205]
      frame False {
      }
      frame True {
        n537 = case shown="True" w1211 {
          tunnel: w1210 -> [w1226 w1386]
          tunnel: [w1226 w1407] -> w1209
          tunnel: w1208 -> [w1227 _]
          tunnel: w1207 -> [_ w1395]
          tunnel: w1206 -> [_ w1378]
          tunnel: w1205 -> [_ _]
          frame False {
            n538 = flat-sequence {
              frame #0 {
              }
            }
            n539 = local read "All Labels (USB6210)"() -> (w1215:string[])
            n540 = Multiply(x="N for sampling", y=i64 2) -> (x*y=w1221:i64)
            n541 = local read "Cycle #"() -> (w1225:u32)
            n542 = Add(x=w1221, y="Mov. Avg Interval") -> (x+y=w1223:i64)
            n543 = Search 1D Array(1D array=w1215, element="Auto Fll\nDewar P. label") -> (index of element=→"Target Index (P)":i32)  [unwired: 1 in]
            n544 = Search 1D Array(1D array=w1215, element="Auto Fll\nHe level label") -> (index of element=→"Target Index (L)":i32)  [unwired: 1 in]
            n545 = Greater?(x=w1225, y=w1223) -> (0:w1219:bool)
            n546 = And(x=w1219, y="Auto Fill ON?") -> (x .and. y?=w1217:bool)
            n547 = case shown="False" w1217 {
              tunnel: w1227 -> [_ w1258]
              tunnel: "Mov. Avg Interval" -> [_ w1242]
              tunnel: w1221 -> [_ w1238]
              tunnel: "N for sampling" -> [_ w1240]
              frame False {
              }
              frame True {
                n548 = local read "Pstd"() -> (→"Pstd history":dbl)
                n549 = local read "Lstd"() -> (→"Lstd history":dbl)
                n550 = local read "Pav (Pa)"() -> (→"Pav history":dbl)
                n551 = local read "Lav (%)"() -> (→"Lav history":dbl)
                n552 = local read "Target Index (P)"() -> (w1259:i32)
                n553 = local read "Target Index (L)"() -> (w1245:i32)
                n554 = Unbundle By Name(w1258) -> ("TimeArray"=w1256:timestamp[], "DataArrayConv"=w1257:dbl[][])
                n555 = Index Array(array=w1257, index (col) #1=w1259, index (col) #2=w1245) -> (element #1=w1244:dbl[], element #2=w1239:dbl[])  [unwired: 2 in]
                n556 = Delete From Array(array=w1244, length=w1238) -> (deleted portion=w1253:dbl[])  [unwired: 1 in, 1 out]
                n557 = Delete From Array(array=w1239, length=w1238) -> (deleted portion=w1237:dbl[])  [unwired: 1 in, 1 out]
                n558 = call "MovingAverage.vi"("Moving Average interval"=w1242, "Input Array"=w1239) -> ("M.A. Array"=w1241:dbl[])  [unwired: 9 in]
                n559 = call "MovingAverage.vi"("Moving Average interval"=w1242, "Input Array"=w1244) -> ("M.A. Array"=w1243:dbl[])  [unwired: 9 in]
                n560 = Delete From Array(array=w1243, length=w1238) -> (deleted portion=w1254:dbl[])  [unwired: 1 in, 1 out]
                n561 = Delete From Array(array=w1243, length=w1240) -> (deleted portion=w1250:dbl[])  [unwired: 1 in, 1 out]
                "Last N M.A. Pressures" <- w1250
                n562 = Delete From Array(array=w1241, length=w1240) -> (deleted portion=w1232:dbl[])  [unwired: 1 in, 1 out]
                "Last N M.A. Levels" <- w1232
                n563 = Delete From Array(array=w1256, length=w1238) -> (deleted portion=w1234:timestamp[])  [unwired: 1 in, 1 out]
                n564 = Bundle("TimeArray"=w1234, "DataArrayConv"=w1253) -> (w1252:T21)  [unwired: 1 in]
                n565 = Bundle("TimeArray"=w1234, "M.A. Array"=w1254) -> (w1255:T22)  [unwired: 1 in]
                n566 = Bundle("TimeArray"=w1234, "DataArrayConv"=w1237) -> (w1236:T21)  [unwired: 1 in]
                n567 = Bundle("TimeArray"=w1234, "M.A. Array"=w1232) -> (w1233:T22)  [unwired: 1 in]
                n568 = Array Size(array=w1250) -> (size(s)=w1249:i32)
                n569 = Equal?(x=w1249, y=w1240) -> (x = y?=w1248:bool)
                n570 = Build Array(w1252, w1255) -> (→"Dewar Pressure":T23)
                n571 = Build Array(w1236, w1233) -> (→"He Level":T23)
                n572 = case shown="True" w1248 {
                  tunnel: [w1363 w1368] -> w1231
                  tunnel: w1250 -> [_ w1369]
                  tunnel: w1232 -> [_ w1366]
                  tunnel: [w1363 w1364] -> w1230
                  frame False {
                    w1363 = nan ("mean")
                  }
                  frame True {
                    n573 = call <vilib>:"Std Deviation and Variance.vi"("X"=w1369) -> ("mean"=w1368:dbl, "standard deviation"=w1367:dbl)  [unwired: 1 in, 1 out]
                    n574 = call <vilib>:"Std Deviation and Variance.vi"("X"=w1366) -> ("mean"=w1364:dbl, "standard deviation"=w1365:dbl)  [unwired: 1 in, 1 out]
                    n575 = local write "Pstd"(w1367) -> ()
                    n576 = local write "Lstd"(w1365) -> ()
                    n577 = local write "Pav (Pa)"(w1368) -> ()
                    n578 = local write "Lav (%)"(w1364) -> ()
                  }
                }
                n579 = flat-sequence {
                  tunnel: w1231 -> [w1260]
                  tunnel: w1230 -> [w1261]
                  frame #0 {
                    n580 = flat-sequence {
                      tunnel: w1261 -> [w1263]
                      tunnel: w1260 -> [w1262]
                      tunnel: w1260 -> [w1331]
                      frame #0 {
                        n581 = stacked-sequence {
                          tunnel: w1263 -> [w1270 w1274 _ _ _ _]
                          tunnel: w1262 -> [_ _ w1288 w1297 w1306 w1315]
                          frame #0 {
                            n582 = local read "L_low (%)"() -> (w1269:dbl)
                            n583 = local read "Fill state"() -> (w1267:bool)
                            n584 = Less?(x=w1270, y=w1269) -> (x < y?=w1266:bool)
                            n585 = Equal?(x=w1267, y=FALSE) -> (x = y?=w1265:bool)
                            n586 = And(x=w1266, y=w1265) -> (x .and. y?=w1264:bool)
                            n587 = case shown="False" w1264 {
                              frame False {
                              }
                              frame True {
                                w1272 = TRUE ("Value (Signaling)")
                                n588 = property on="Fill state" class="Bool (strict)"("Val(Sgnl)"=w1272) -> ()  [unwired: 2 in, 2 out]
                                n589 = Not(x=w1272) -> (.not. x?=w1271:bool)
                                n590 = property on="Fill (false)" class="Bool (strict)"("Val(Sgnl)"=w1271) -> ()  [unwired: 2 in, 2 out]
                              }
                            }
                          }
                          frame #1 {
                            n591 = local read "L_high (%)"() -> (w1275:dbl)
                            n592 = local read "Fill state"() -> (w1278:bool)
                            n593 = Greater?(x=w1274, y=w1275) -> (0:w1273:bool)
                            n594 = Equal?(x=w1278, y=TRUE) -> (x = y?=w1277:bool)
                            n595 = And(x=w1273, y=w1277) -> (x .and. y?=w1276:bool)
                            n596 = case shown="True" w1276 {
                              frame False {
                              }
                              frame True {
                                w1280 = FALSE ("Value (Signaling)")
                                n597 = property on="Fill state" class="Bool (strict)"("Val(Sgnl)"=w1280) -> ()  [unwired: 2 in, 2 out]
                                n598 = Not(x=w1280) -> (.not. x?=w1281:bool)
                                n599 = property on="Fill (false)" class="Bool (strict)"("Val(Sgnl)"=w1281) -> ()  [unwired: 2 in, 2 out]
                              }
                            }
                          }
                          frame #2 {
                            n600 = local read "P_1_low (Pa)"() -> (w1287:dbl)
                            n601 = property on="state 1" class="Bool (strict)"() -> ("Value"=w1285:bool)  [unwired: 2 in, 2 out]
                            n602 = Less?(x=w1288, y=w1287) -> (x < y?=w1284:bool)
                            n603 = Equal?(x=w1285, y=FALSE) -> (x = y?=w1283:bool)
                            n604 = And(x=w1283, y=w1284) -> (x .and. y?=w1282:bool)
                            n605 = case shown="True" w1282 {
                              frame False {
                              }
                              frame True {
                                w1290 = TRUE ("Value (Signaling)")
                                n606 = property on="state 1" class="Bool (strict)"("Val(Sgnl)"=w1290) -> ()  [unwired: 2 in, 2 out]
                                n607 = Not(x=w1290) -> (.not. x?=w1289:bool)
                                n608 = property on="state 1 (false)" class="Bool (strict)"("Val(Sgnl)"=w1289) -> ()  [unwired: 2 in, 2 out]
                              }
                            }
                          }
                          frame #3 {
                            n609 = local read "P_1_high (Pa)"() -> (w1296:dbl)
                            n610 = property on="state 1" class="Bool (strict)"() -> ("Value"=w1294:bool)  [unwired: 2 in, 2 out]
                            n611 = Greater?(x=w1297, y=w1296) -> (0:w1293:bool)
                            n612 = Equal?(x=w1294, y=TRUE) -> (x = y?=w1292:bool)
                            n613 = And(x=w1292, y=w1293) -> (x .and. y?=w1291:bool)
                            n614 = case shown="True" w1291 {
                              frame False {
                              }
                              frame True {
                                w1299 = FALSE ("Value (Signaling)")
                                n615 = property on="state 1" class="Bool (strict)"("Val(Sgnl)"=w1299) -> ()  [unwired: 2 in, 2 out]
                                n616 = Not(x=w1299) -> (.not. x?=w1298:bool)
                                n617 = property on="state 1 (false)" class="Bool (strict)"("Val(Sgnl)"=w1298) -> ()  [unwired: 2 in, 2 out]
                              }
                            }
                          }
                          frame #4 {
                            n618 = local read "P_2_low (Pa)"() -> (w1305:dbl)
                            n619 = property on="state 2" class="Bool (strict)"() -> ("Value"=w1300:bool)  [unwired: 2 in, 2 out]
                            n620 = Less?(x=w1306, y=w1305) -> (x < y?=w1303:bool)
                            n621 = Equal?(x=w1300, y=FALSE) -> (x = y?=w1302:bool)
                            n622 = And(x=w1302, y=w1303) -> (x .and. y?=w1301:bool)
                            n623 = case shown="True" w1301 {
                              frame False {
                              }
                              frame True {
                                w1307 = TRUE ("Value (Signaling)")
                                n624 = property on="state 2" class="Bool (strict)"("Val(Sgnl)"=w1307) -> ()  [unwired: 2 in, 2 out]
                                n625 = Not(x=w1307) -> (.not. x?=w1308:bool)
                                n626 = property on="state 2 (false)" class="Bool (strict)"("Val(Sgnl)"=w1308) -> ()  [unwired: 2 in, 2 out]
                              }
                            }
                          }
                          frame #5 {
                            n627 = local read "P_2_high (Pa)"() -> (w1314:dbl)
                            n628 = property on="state 2" class="Bool (strict)"() -> ("Value"=w1309:bool)  [unwired: 2 in, 2 out]
                            n629 = Greater?(x=w1315, y=w1314) -> (0:w1312:bool)
                            n630 = Equal?(x=w1309, y=TRUE) -> (x = y?=w1311:bool)
                            n631 = And(x=w1311, y=w1312) -> (x .and. y?=w1310:bool)
                            n632 = case shown="True" w1310 {
                              frame False {
                              }
                              frame True {
                                w1316 = FALSE ("Value (Signaling)")
                                n633 = property on="state 2" class="Bool (strict)"("Val(Sgnl)"=w1316) -> ()  [unwired: 2 in, 2 out]
                                n634 = Not(x=w1316) -> (.not. x?=w1317:bool)
                                n635 = property on="state 2 (false)" class="Bool (strict)"("Val(Sgnl)"=w1317) -> ()  [unwired: 2 in, 2 out]
                              }
                            }
                          }
                        }
                      }
                      frame #1 {
                        n636 = property on="Fill state" class="Bool (strict)"() -> ("Value"=w1318:bool)  [unwired: 2 in, 2 out]
                        n637 = case shown="True" w1318 {
                          frame False {
                            n638 = property on="V1 (N.O.)" class="Bool (strict)"("Val(Sgnl)"=TRUE ("V1 (N.O.)")) -> ()  [unwired: 2 in, 2 out]
                            n639 = property on="V2 (N.C.)" class="Bool (strict)"("Val(Sgnl)"=FALSE ("Value (Signaling)")) -> ()  [unwired: 2 in, 2 out]
                          }
                          frame True {
                            n640 = property on="state 1" class="Bool (strict)"() -> ("Value"=w1322:bool)  [unwired: 2 in, 2 out]
                            n641 = property on="state 2" class="Bool (strict)"() -> ("Value"=w1321:bool)  [unwired: 2 in, 2 out]
                            n642 = case shown="True" w1322 {
                              frame False {
                                n643 = property on="V1 (N.O.)" class="Bool (strict)"("Val(Sgnl)"=TRUE ("Value (Signaling)")) -> ()  [unwired: 2 in, 2 out]
                                n644 = local write "Status V1 CTRL"(enum16{"Pressurize", "Release"}."Release" ("Status V1 CTRL")) -> ()
                              }
                              frame True {
                                n645 = property on="V1 (N.O.)" class="Bool (strict)"("Val(Sgnl)"=FALSE ("V1 (N.O.)")) -> ()  [unwired: 2 in, 2 out]
                                n646 = local write "Status V1 CTRL"(enum16{"Pressurize", "Release"}."Pressurize" ("Status V1 CTRL")) -> ()
                              }
                            }
                            n647 = case shown="True" w1321 {
                              frame False {
                                n648 = property on="V2 (N.C.)" class="Bool (strict)"("Val(Sgnl)"=FALSE ("Value (Signaling)")) -> ()  [unwired: 2 in, 2 out]
                                n649 = local write "Status V2 CTRL"(enum16{"Pressurize", "Release"}."Release" ("Status V2 CTRL")) -> ()
                              }
                              frame True {
                                n650 = property on="V2 (N.C.)" class="Bool (strict)"("Val(Sgnl)"=TRUE ("Value (Signaling)")) -> ()  [unwired: 2 in, 2 out]
                                n651 = local write "Status V2 CTRL"(enum16{"Pressurize", "Release"}."Pressurize" ("Status V2 CTRL")) -> ()
                              }
                            }
                          }
                        }
                      }
                      frame #2 {
                        n652 = Greater?(x=w1331, y="P_safelimit_high (Pa)") -> (0:w1333:bool)
                        n653 = Less?(x=w1331, y="P_safelimit_low (Pa)") -> (x < y?=w1335:bool)
                        n654 = Or(x=w1333, y=w1335) -> (x .or. y?=w1336:bool)
                        n655 = case shown="False" w1336 {
                          frame False {
                          }
                          frame True {
                            w1337 = FALSE ("Value (Signaling)")
                            w1339 = FALSE ("Value (Signaling)")
                            n656 = property on="V2 (N.C.)" class="Bool (strict)"("Val(Sgnl)"=FALSE ("V1 (N.O.)")) -> ()  [unwired: 2 in, 2 out]
                            n657 = property on="V1 (N.O.)" class="Bool (strict)"("Val(Sgnl)"=TRUE ("V1 (N.O.)")) -> ()  [unwired: 2 in, 2 out]
                            n658 = property on="state 1" class="Bool (strict)"("Val(Sgnl)"=w1337) -> ()  [unwired: 2 in, 2 out]
                            n659 = property on="state 2" class="Bool (strict)"("Val(Sgnl)"=w1339) -> ()  [unwired: 2 in, 2 out]
                            n660 = Not(x=w1337) -> (.not. x?=w1338:bool)
                            n661 = Not(x=w1339) -> (.not. x?=w1340:bool)
                            n662 = property on="state 1 (false)" class="Bool (strict)"("Val(Sgnl)"=w1338) -> ()  [unwired: 2 in, 2 out]
                            n663 = property on="state 2 (false)" class="Bool (strict)"("Val(Sgnl)"=w1340) -> ()  [unwired: 2 in, 2 out]
                          }
                        }
                      }
                    }
                  }
                  frame #1 {
                    n664 = property on="V1 (N.O.)" class="Bool (strict)"() -> ("Value"=w1361:bool)  [unwired: 2 in, 2 out]
                    n665 = local read "L_high (%)"() -> (w1351:dbl)
                    n666 = property on="V2 (N.C.)" class="Bool (strict)"() -> ("Value"=w1350:bool)  [unwired: 2 in, 2 out]
                    n667 = local read "P_1_high (Pa)"() -> (w1355:dbl)
                    n668 = local read "P_2_high (Pa)"() -> (w1353:dbl)
                    n669 = local read "P_1_low (Pa)"() -> (w1356:dbl)
                    n670 = local read "P_2_low (Pa)"() -> (w1354:dbl)
                    n671 = local read "L_low (%)"() -> (w1352:dbl)
                    n672 = local read "Pav (Pa)"() -> (w1344:dbl)
                    n673 = Boolean To (0,1)(Boolean=w1361) -> (0, 1=w1362:i16)
                    n674 = local read "Lav (%)"() -> (w1343:dbl)
                    n675 = Boolean To (0,1)(Boolean=w1350) -> (0, 1=w1349:i16)
                    n676 = local read "File Refn DewarCTRL"() -> (w1357:refnum<file>)
                    n677 = local read "Cycle #"() -> (w1360:u32)
                    n678 = Build Array(w1344, w1343, w1356, w1355, w1354, w1353, w1352, w1351, w1362, w1349) -> (w1348:dbl[])
                    n679 = Get Date/Time In Seconds() -> (seconds since 1Jan1904=w1358:timestamp)
                    n680 = call "FileWrite.vi"("DataArray"=w1348, "Time Stamp"=w1358, "Error In"=errorcluster {"status"=FALSE, "code"=0, "source"=""}, "FileFormat"=string[] ["%4.5e", "%4.2f", "%4.4e", "%4.4e", "%4.4e", "%4.4e", "%4.4e", "%d", "%d"] ("Array"), "Index"=w1360, "refnum in"=w1357) -> ("Error Out"=→"Error Out (Dewar CTRL":errorcluster, "Byte Stream File Refnum"=w1347:refnum<file>)  [unwired: 4 in]
                    n681 = local write "File Refn DewarCTRL"(w1347) -> ()
                  }
                }
              }
            }
          }
          frame True {
            w1401 = "_"
            w1370 = FALSE ("auto cleanup")
            w1406 = 1 items=["one channel for each line", "one channel for all lines"] ("line grouping")
            n682 = flat-sequence {
              frame #0 {
                w1421 = FALSE ("V1 (N.O.)")
                n683 = local write "V1 (N.O.)"(TRUE ("V1 (N.O.)")) -> ()
                n684 = local write "V2 (N.C.)"(FALSE ("V1 (N.O.)")) -> ()
                n685 = local write "state 1"(w1421) -> ()
                n686 = local write "state 2"(w1421) -> ()
                n687 = local write "Fill state"(w1421) -> ()
                n688 = Not(x=w1421) -> (.not. x?=w1423:bool)
                n689 = Not(x=w1421) -> (.not. x?=w1422:bool)
                n690 = local write "state 1 (false)"(w1422) -> ()
                n691 = local write "state 2 (false)"(w1422) -> ()
                n692 = local write "Fill (false)"(w1423) -> ()
              }
            }
            n693 = Get Date/Time In Seconds() -> (seconds since 1Jan1904=w1418:timestamp)
            n694 = call "LV_UNIXTIME.vi"("current time"=w1418) -> ("date/time string"=w1396:string)  [unwired: 9 in, 1 out]
            n695 = Concatenate Strings(w1396, "_DO" ("new task name")) -> (w1415:string)
            n696 = Concatenate Strings(w1395, w1401, w1396, w1401) -> (w1377:string)
            n697 = Concatenate Strings(w1377, "DEWAR.csv" ("string")) -> (w1376:string)
            n698 = Concatenate Strings(w1377, "USB_DOUT.csv" ("string")) -> (w1380:string)
            n699 = Build Path(base path=w1378, name or relative path=w1376) -> (appended path=w1375:path)
            n700 = Build Path(base path=w1378, name or relative path=w1380) -> (appended path=w1400:path)
            n701 = Open/Create/Replace File(file path (use dialog)=w1400, error in=w1386, operation (0:open)=T17."open or create") -> (refnum out=w1398:refnum<file>, error out=w1385:errorcluster)  [unwired: 3 in, 1 out]
            n702 = call "FileIntialize.vi"("Error In"=w1385, "Labels"="DOUT Labels", "refnum in"=w1398) -> ("Error Out"=w1372:errorcluster, "File Refnum"=→"File Refn USB DO":refnum<file>)  [unwired: 7 in]
            n703 = Open/Create/Replace File(file path (use dialog)=w1375, error in=w1372, operation (0:open)=T17."open or create") -> (refnum out=w1383:refnum<file>, error out=w1384:errorcluster)  [unwired: 3 in, 1 out]
            n704 = call "FileIntialize.vi"("Error In"=w1384, "Labels"=string[] ["P_av", "L_av", "P_1_low", "P_1_high", "P_2_low", "P_2_high", "L_low", "L_high", "V1(NO)", "V2(NC)"], "refnum in"=w1383) -> ("Error Out"=w1371:errorcluster, "File Refnum"=→"File Refn DewarCTRL":refnum<file>)  [unwired: 7 in]
            n705 = Index Array(array="DOUT Physical CH", index=2) -> (element=w1388:tag)
            n706 = Index Array(array="DOUT Physical CH", index=1) -> (element=w1391:tag)
            n707 = Index Array(array="DOUT Physical CH", index=0) -> (element=w1393:tag)
            n708 = call <vilib>:"DAQmx Create Task.vi"("new task name"=w1415, "auto cleanup"=FALSE, "error in"=w1371) -> ("task out"=w1416:refnum<k21>, "error out"=w1417:errorcluster)  [unwired: 11 in]
            n709 = call-poly <vilib>:"DAQmx Create Virtual Channel.vi"("task in"=w1416, "lines"=w1393, "line grouping"=w1406, "error in"=w1417) -> ("task out"=w1419:refnum<k21>, "error out"=w1420:errorcluster)  [unwired: 10 in]
            n710 = call-poly <vilib>:"DAQmx Create Virtual Channel.vi"("task in"=w1419, "lines"=w1391, "line grouping"=w1406, "error in"=w1420) -> ("task out"=w1405:refnum<k21>, "error out"=w1403:errorcluster)  [unwired: 10 in]
            n711 = call-poly <vilib>:"DAQmx Create Virtual Channel.vi"("task in"=w1405, "lines"=w1388, "line grouping"=w1406, "error in"=w1403) -> ("task out"=w1404:refnum<k21>, "error out"=w1402:errorcluster)  [unwired: 10 in]
            n712 = call <vilib>:"DAQmx Start Task.vi"("task/channels in"=w1404, "error in"=w1402) -> ("task out"=w1410:refnum<k21>, "error out"=w1408:errorcluster)  [unwired: 12 in]
            n713 = Build Array(w1370, w1370, w1370) -> (w1411:bool[])
            n714 = call <vilib>:"DAQmx Write (Digital 1D Bool NChan 1Samp 1Line).vi"("task/channels in"=w1410, "data"=w1411, "timeout"=10.0, "error in"=w1408) -> ("task out"=→"DOUT task out":refnum<k21>, "error out"=w1407:errorcluster)  [unwired: 9 in, 1 out]
          }
        }
      }
    }
    "error out (USB6210/6218 DOUT)" <- w551
    n715 = flat-sequence {
      tunnel: w598 -> [w1087]
      tunnel: [w1082] -> w586
      tunnel: [w1080] -> w584
      tunnel: [w1079] -> w581
      tunnel: [w1078] -> w579
      tunnel: w550 -> [w1073]
      frame #0 {
        w1081 = T18 [] ("appended array")
        n716 = Unbundle By Name(w1073) -> ("TimeArray"=w1090:timestamp[], "DataArrayConv"=w1085:dbl[][], "LDArray"=w1084:dbl[])
        n717 = Unbundle By Name(w1087) -> ("ReadLeakDet?"=w1086:bool, "LabelLD"=w1089:string, "Labels"=w1083:string[])  [unwired: 1 out]
        n718 = case shown="True" w1086 {
          tunnel: w1089 -> [_ w1098]
          tunnel: w1085 -> [w1092 w1097]
          tunnel: w1084 -> [_ w1096]
          tunnel: [w1092 w1095] -> w1072
          tunnel: w1083 -> [w1091 w1094]
          tunnel: [w1091 w1093] -> w1075
          frame False {
          }
          frame True {
            n719 = Build Array (concatenate)(w1097, w1096) -> (w1095:dbl[][])
            n720 = Build Array (concatenate)(w1094, w1098) -> (w1093:string[])
          }
        }
        "All Labels (USB6210)" <- w1075
        "DataArrayConv (USB6210)" <- w1072
        n721 = local read "Plot selecter (USB6210)\n    1      2     3     4"() -> (w1077:bool[][])
        n722 = control-ref of="Plot selecter (USB6210)\n    1      2     3     4"() -> (w1074:refnum<vi>)
        n723 = Array Size(array=w1075) -> (size(s)=w1088:i32)
        n724 = Array Size(array=w1075) -> (size(s)=w1076:i32)
        n725 = Array Size(array=w1072) -> (size(s)=→"Data Array sizes (6210)":i32[])
        n726 = property on="Property Node" class="Arr (strict)"(reference=w1074, "Number of Rows"=w1076) -> ()  [unwired: 1 in, 2 out]
        n727 = for {
          N: w1088 -> [_]
          tunnel: w1072 -> [w1119]
          tunnel: w1090 -> [w1120]
          shift-right: [w1115] -> w1080
          shift-left: w1081 -> [w1118]
          shift-right: [w1113] -> w1078
          shift-left: w1081 -> [w1116]
          shift-right: [w1114] -> w1082
          shift-left: w1081 -> [w1112]
          shift-right: [w1111] -> w1079
          shift-left: w1081 -> [w1110]
          tunnel: w1077 -> [w1109]
          i -> [w1104]
          n728 = Index Array(array=w1119, index (col)=w1104) -> (element=w1099:dbl[])  [unwired: 1 in]
          n729 = Index Array(array=w1109, index (row) #1=w1104, index (col) #1=0 ("index (row)"), index (row) #2=w1104, index (col) #2=1 ("index (row)"), index (row) #3=w1104, index (col) #3=2 ("index (row)"), index (row) #4=w1104, index (col) #4=3 ("index (row)")) -> (element #1=w1103:bool, element #2=w1102:bool, element #3=w1101:bool, element #4=w1100:bool)
          n730 = Bundle("TimeArray"=w1120, "DataArrayConv"=w1099) -> (w1117:T21)  [unwired: 1 in]
          n731 = stacked-sequence {
            tunnel: w1103 -> [w1124 _ _ _]
            tunnel: w1118 -> [_ w1132 _ _]
            tunnel: w1101 -> [_ _ w1140 _]
            tunnel: w1117 -> [w1121 w1130 w1139 w1145]
            tunnel: w1100 -> [_ _ _ w1148]
            tunnel: w1116 -> [_ _ _ w1147]
            tunnel: [_ _ _ w1146] -> w1113
            tunnel: [_ w1131 _ _] -> w1115
            tunnel: [w1123 _ _ _] -> w1114
            tunnel: w1112 -> [w1122 _ _ _]
            tunnel: [_ _ w1138 _] -> w1111
            tunnel: w1110 -> [_ _ w1137 _]
            tunnel: w1102 -> [_ w1129 _ _]
            frame #0 {
              n732 = case shown="True" w1124 {
                tunnel: [w1125 w1128] -> w1123
                tunnel: w1121 -> [_ w1127]
                tunnel: w1122 -> [w1125 w1126]
                frame False {
                }
                frame True {
                  n733 = Build Array (concatenate)(w1126, w1127) -> (w1128:T18)
                }
              }
            }
            frame #1 {
              n734 = case shown="True" w1129 {
                tunnel: w1132 -> [w1133 w1136]
                tunnel: [w1133 w1135] -> w1131
                tunnel: w1130 -> [_ w1134]
                frame False {
                }
                frame True {
                  n735 = Build Array (concatenate)(w1136, w1134) -> (w1135:T18)
                }
              }
            }
            frame #2 {
              n736 = case shown="True" w1140 {
                tunnel: [w1141 w1144] -> w1138
                tunnel: w1139 -> [_ w1143]
                tunnel: w1137 -> [w1141 w1142]
                frame False {
                }
                frame True {
                  n737 = Build Array (concatenate)(w1142, w1143) -> (w1144:T18)
                }
              }
            }
            frame #3 {
              n738 = case shown="True" w1148 {
                tunnel: [w1149 w1152] -> w1146
                tunnel: w1145 -> [_ w1151]
                tunnel: w1147 -> [w1149 w1150]
                frame False {
                }
                frame True {
                  n739 = Build Array (concatenate)(w1150, w1151) -> (w1152:T18)
                }
              }
            }
          }
        }
      }
    }
    n740 = flat-sequence {
      tunnel: w546 -> [w1006]
      tunnel: [w1001] -> w545
      tunnel: [w999] -> w544
      tunnel: [w998] -> w543
      tunnel: [w997] -> w542
      tunnel: w547 -> [w993]
      frame #0 {
        w1000 = T18 [] ("appended array")
        n741 = Unbundle By Name(w993) -> ("TimeArray"=w989:timestamp[], "DataArrayConv"=w1004:dbl[][], "LDArray"=w1003:dbl[])
        "TimeArray (USB6218)" <- w989
        n742 = Unbundle By Name(w1006) -> ("ReadLeakDet?"=w1005:bool, "LabelLD"=w1008:string, "Labels"=w1002:string[])  [unwired: 1 out]
        n743 = case shown="True" w1005 {
          tunnel: w1008 -> [_ w1016]
          tunnel: w1004 -> [w1010 w1015]
          tunnel: w1003 -> [_ w1014]
          tunnel: [w1010 w1013] -> w991
          tunnel: w1002 -> [w1009 w1012]
          tunnel: [w1009 w1011] -> w994
          frame False {
          }
          frame True {
            n744 = Build Array (concatenate)(w1015, w1014) -> (w1013:dbl[][])
            n745 = Build Array (concatenate)(w1012, w1016) -> (w1011:string[])
          }
        }
        "All Labels (USB6218)" <- w994
        "DataArrayConv (USB6218)" <- w991
        n746 = Array Size(array=w989) -> (size(s)=→"TimeArray size (6218)":i32)
        n747 = local read "Plot selecter (USB6218)\n    1      2     3     4"() -> (w996:bool[][])
        n748 = control-ref of="Plot selecter (USB6218)\n    1      2     3     4"() -> (w992:refnum<vi>)
        n749 = Array Size(array=w994) -> (size(s)=w1007:i32)
        n750 = Array Size(array=w994) -> (size(s)=w995:i32)
        n751 = property on="Property Node" class="Arr (strict)"(reference=w992, "Number of Rows"=w995) -> ()  [unwired: 1 in, 2 out]
        n752 = for {
          N: w1007 -> [_]
          tunnel: w991 -> [w1037]
          tunnel: w989 -> [w1038]
          shift-right: [w1032] -> w999
          shift-left: w1000 -> [w1035]
          shift-right: [w1030] -> w997
          shift-left: w1000 -> [w1033]
          shift-right: [w1031] -> w1001
          shift-left: w1000 -> [w1029]
          shift-right: [w1028] -> w998
          shift-left: w1000 -> [w1027]
          tunnel: w996 -> [w1026]
          i -> [w1021]
          n753 = Index Array(array=w1037, index (col)=w1021) -> (element=w1036:dbl[])  [unwired: 1 in]
          n754 = Index Array(array=w1026, index (row) #1=w1021, index (col) #1=0 ("index (row)"), index (row) #2=w1021, index (col) #2=1 ("index (row)"), index (row) #3=w1021, index (col) #3=2 ("index (row)"), index (row) #4=w1021, index (col) #4=3 ("index (row)")) -> (element #1=w1020:bool, element #2=w1019:bool, element #3=w1018:bool, element #4=w1017:bool)
          n755 = Bundle("TimeArray"=w1038, "DataArrayConv"=w1036) -> (w1034:T21)  [unwired: 1 in]
          n756 = stacked-sequence {
            tunnel: w1020 -> [w1042 _ _ _]
            tunnel: w1035 -> [_ w1050 _ _]
            tunnel: w1018 -> [_ _ w1058 _]
            tunnel: w1034 -> [w1039 w1048 w1057 w1063]
            tunnel: w1017 -> [_ _ _ w1066]
            tunnel: w1033 -> [_ _ _ w1065]
            tunnel: [_ _ _ w1064] -> w1030
            tunnel: [_ w1049 _ _] -> w1032
            tunnel: [w1041 _ _ _] -> w1031
            tunnel: w1029 -> [w1040 _ _ _]
            tunnel: [_ _ w1056 _] -> w1028
            tunnel: w1027 -> [_ _ w1055 _]
            tunnel: w1019 -> [_ w1047 _ _]
            frame #0 {
              n757 = case shown="True" w1042 {
                tunnel: [w1043 w1046] -> w1041
                tunnel: w1039 -> [_ w1045]
                tunnel: w1040 -> [w1043 w1044]
                frame False {
                }
                frame True {
                  n758 = Build Array (concatenate)(w1044, w1045) -> (w1046:T18)
                }
              }
            }
            frame #1 {
              n759 = case shown="True" w1047 {
                tunnel: w1050 -> [w1051 w1054]
                tunnel: [w1051 w1053] -> w1049
                tunnel: w1048 -> [_ w1052]
                frame False {
                }
                frame True {
                  n760 = Build Array (concatenate)(w1054, w1052) -> (w1053:T18)
                }
              }
            }
            frame #2 {
              n761 = case shown="True" w1058 {
                tunnel: [w1059 w1062] -> w1056
                tunnel: w1057 -> [_ w1061]
                tunnel: w1055 -> [w1059 w1060]
                frame False {
                }
                frame True {
                  n762 = Build Array (concatenate)(w1060, w1061) -> (w1062:T18)
                }
              }
            }
            frame #3 {
              n763 = case shown="True" w1066 {
                tunnel: [w1067 w1070] -> w1064
                tunnel: w1063 -> [_ w1069]
                tunnel: w1065 -> [w1067 w1068]
                frame False {
                }
                frame True {
                  n764 = Build Array (concatenate)(w1068, w1069) -> (w1070:T18)
                }
              }
            }
          }
        }
        n765 = Array Size(array=w991) -> (size(s)=→"DataArraySize (6218)":i32[])
      }
    }
    n766 = local read "Plot selecter LSI218(1)\n    1      2     3     4"() -> (w574:bool[][])
    n767 = local read "Plot selecter LSI218(2)\n    1      2     3     4"() -> (w573:bool[][])
    n768 = Array Size(array=w529) -> (size(s)=→"TimeArray Size (336)":i32)
    n769 = Array Size(array=w527) -> (size(s)=→"DataArray size (336)":i32[])
    n770 = for {
      N: 48 -> [_]
      tunnel: w589 -> [w1526]
      tunnel: w588 -> [w1523]
      tunnel: w574 -> [w1507]
      tunnel: w573 -> [w1508]
      shift-right: [w1524] -> w587
      shift-left: w585 -> [w1525]
      shift-right: [w1519] -> w582
      shift-left: w585 -> [w1520]
      shift-right: [w1518] -> w580
      shift-left: w585 -> [w1517]
      shift-right: [w1516] -> w578
      shift-left: w585 -> [w1515]
      i -> [w1513]
      n771 = Index Array(array=w1523, index (col)=w1513) -> (element=w1522:dbl[])  [unwired: 1 in]
      n772 = Less?(x=w1513, y=24) -> (x < y?=w1514:bool)
      n773 = case shown="True" w1514 {
        tunnel: [w1531 w1549] -> w1512
        tunnel: [w1530 w1548] -> w1511
        tunnel: [w1529 w1546] -> w1510
        tunnel: [w1528 w1545] -> w1509
        tunnel: w1507 -> [_ w1544]
        tunnel: w1508 -> [w1538 _]
        tunnel: w1513 -> [w1533 w1541]
        frame False {
          n774 = Subtract(x=w1533, y=24) -> (x-y=w1537:i32)
          n775 = Index Array(array=w1538, index (row) #1=w1537, index (col) #1=0 ("index (row)"), index (row) #2=w1537, index (col) #2=1 ("index (row)"), index (row) #3=w1537, index (col) #3=2 ("index (row)"), index (row) #4=w1537, index (col) #4=3 ("index (row)")) -> (element #1=w1531:bool, element #2=w1530:bool, element #3=w1529:bool, element #4=w1528:bool)
        }
        frame True {
          n776 = Index Array(array=w1544, index (row) #1=w1541, index (col) #1=0 ("index (row)"), index (row) #2=w1541, index (col) #2=1 ("index (row)"), index (row) #3=w1541, index (col) #3=2 ("index (row)"), index (row) #4=w1541, index (col) #4=3 ("index (row)")) -> (element #1=w1549:bool, element #2=w1548:bool, element #3=w1546:bool, element #4=w1545:bool)
        }
      }
      n777 = Bundle("TimeArray"=w1526, "DataArray"=w1522) -> (w1521:T24)  [unwired: 1 in]
      n778 = stacked-sequence {
        tunnel: w1525 -> [w1553 _ _ _]
        tunnel: [w1552 _ _ _] -> w1524
        tunnel: w1521 -> [w1551 w1561 w1569 w1577]
        tunnel: w1520 -> [_ w1560 _ _]
        tunnel: [_ w1559 _ _] -> w1519
        tunnel: [_ _ w1568 _] -> w1518
        tunnel: w1517 -> [_ _ w1567 _]
        tunnel: [_ _ _ w1576] -> w1516
        tunnel: w1515 -> [_ _ _ w1575]
        tunnel: w1512 -> [w1550 _ _ _]
        tunnel: w1511 -> [_ w1558 _ _]
        tunnel: w1510 -> [_ _ w1566 _]
        tunnel: w1509 -> [_ _ _ w1574]
        frame #0 {
          n779 = case shown="False" w1550 {
            tunnel: w1551 -> [_ w1555]
            tunnel: w1553 -> [w1554 w1557]
            tunnel: [w1554 w1556] -> w1552
            frame False {
            }
            frame True {
              n780 = Build Array (concatenate)(w1557, w1555) -> (w1556:T4)
            }
          }
        }
        frame #1 {
          n781 = case shown="True" w1558 {
            tunnel: [w1562 w1565] -> w1559
            tunnel: w1561 -> [_ w1564]
            tunnel: w1560 -> [w1562 w1563]
            frame False {
            }
            frame True {
              n782 = Build Array (concatenate)(w1563, w1564) -> (w1565:T4)
            }
          }
        }
        frame #2 {
          n783 = case shown="True" w1566 {
            tunnel: [w1570 w1573] -> w1568
            tunnel: w1569 -> [_ w1572]
            tunnel: w1567 -> [w1570 w1571]
            frame False {
            }
            frame True {
              n784 = Build Array (concatenate)(w1571, w1572) -> (w1573:T4)
            }
          }
        }
        frame #3 {
          n785 = case shown="True" w1574 {
            tunnel: [w1578 w1581] -> w1576
            tunnel: w1577 -> [_ w1580]
            tunnel: w1575 -> [w1578 w1579]
            frame False {
            }
            frame True {
              n786 = Build Array (concatenate)(w1579, w1580) -> (w1581:T4)
            }
          }
        }
      }
    }
    n787 = local read "Plot selecter LSI336 \n     1      2     3     4"() -> (w569:bool[][])
    n788 = local read "Labels LSI336"() -> (w561:string[])
    n789 = Array Size(array=w561) -> (size(s)=w560:i32)
    n790 = for {
      N: w560 -> [_]
      tunnel: w569 -> [w1438]
      shift-right: [w1432] -> w567
      shift-left: w568 -> [w1447]
      shift-right: [w1428] -> w566
      shift-left: w568 -> [w1445]
      shift-right: [w1429] -> w565
      shift-left: w568 -> [w1444]
      shift-right: [w1427] -> w564
      shift-left: w568 -> [w1443]
      tunnel: w527 -> [w1435]
      tunnel: w529 -> [w1433]
      i -> [w1436]
      n791 = Index Array(array=w1435, index (col)=w1436) -> (element=w1434:dbl[])  [unwired: 1 in]
      n792 = Index Array(array=w1438, index (row) #1=w1436, index (col) #1=0 ("index (row)"), index (row) #2=w1436, index (col) #2=1 ("index (row)"), index (row) #3=w1436, index (col) #3=2 ("index (row)"), index (row) #4=w1436, index (col) #4=3 ("index (row)")) -> (element #1=w1437:bool, element #2=w1431:bool, element #3=w1430:bool, element #4=w1426:bool)
      n793 = Bundle("TimeArray"=w1433, "DataArray"=w1434) -> (w1446:T24)  [unwired: 1 in]
      n794 = stacked-sequence {
        tunnel: w1447 -> [w1451 _ _ _]
        tunnel: [w1450 _ _ _] -> w1432
        tunnel: w1446 -> [w1449 w1459 w1467 w1475]
        tunnel: w1445 -> [_ w1458 _ _]
        tunnel: [_ w1457 _ _] -> w1428
        tunnel: [_ _ w1466 _] -> w1429
        tunnel: w1444 -> [_ _ w1465 _]
        tunnel: [_ _ _ w1474] -> w1427
        tunnel: w1443 -> [_ _ _ w1473]
        tunnel: w1437 -> [w1448 _ _ _]
        tunnel: w1431 -> [_ w1456 _ _]
        tunnel: w1430 -> [_ _ w1464 _]
        tunnel: w1426 -> [_ _ _ w1472]
        frame #0 {
          n795 = case shown="False" w1448 {
            tunnel: w1449 -> [_ w1453]
            tunnel: w1451 -> [w1452 w1455]
            tunnel: [w1452 w1454] -> w1450
            frame False {
            }
            frame True {
              n796 = Build Array (concatenate)(w1455, w1453) -> (w1454:T4)
            }
          }
        }
        frame #1 {
          n797 = case shown="True" w1456 {
            tunnel: [w1460 w1463] -> w1457
            tunnel: w1459 -> [_ w1461]
            tunnel: w1458 -> [w1460 w1462]
            frame False {
            }
            frame True {
              n798 = Build Array (concatenate)(w1462, w1461) -> (w1463:T4)
            }
          }
        }
        frame #2 {
          n799 = case shown="True" w1464 {
            tunnel: [w1468 w1471] -> w1466
            tunnel: w1467 -> [_ w1469]
            tunnel: w1465 -> [w1468 w1470]
            frame False {
            }
            frame True {
              n800 = Build Array (concatenate)(w1470, w1469) -> (w1471:T4)
            }
          }
        }
        frame #3 {
          n801 = case shown="True" w1472 {
            tunnel: [w1476 w1479] -> w1474
            tunnel: w1475 -> [_ w1477]
            tunnel: w1473 -> [w1476 w1478]
            frame False {
            }
            frame True {
              n802 = Build Array (concatenate)(w1478, w1477) -> (w1479:T4)
            }
          }
        }
      }
    }
    n803 = Build Array (concatenate)(w586, w587, w567, w545) -> (→"Graph 1":T18)
    n804 = Build Array (concatenate)(w584, w582, w566, w544) -> (→"Graph 2":T18)
    n805 = Build Array (concatenate)(w579, w578, w564, w542) -> (→"Graph 4":T18)
    n806 = Build Array (concatenate)(w581, w580, w565, w543) -> (→"Graph 3":T18)
    "Cycle #" <- w510
  }
  n807 = while {
    stop <- w1670 stop-if-true
    n808 = Get Date/Time In Seconds() -> (seconds since 1Jan1904=w1668:timestamp)
    n809 = Wait (ms)(milliseconds to wait=u32 123) -> ()  [unwired: 1 out]
    n810 = event shown="[1] \"Frontpanel screenshots\": Value Change" {
      selector: _ -> [_ _ _]
      dyn-events: _ -> [_ _ _]
      timeout: _ -> [_ _ _]
      tunnel: [FALSE _ TRUE] -> w1670
      tunnel: "Base Path (screenshots)" -> [_ w1678 _]
      tunnel: w1668 -> [_ w1677 _]
      event Timeout {
        n811 = event-data() -> ()  [unwired: 1 in, 3 out]
      }
      event "Frontpanel screenshots": Value Change {
        n812 = event-data() -> ()  [unwired: 1 in, 3 out]
        n813 = property class="TabCtl (strict)"() -> ("Value"=w1675:T1)  [unwired: 2 in, 2 out]
        n814 = stacked-sequence {
          tunnel: w1678 -> [w1684 w1706 w1728 w1750 w1772 w1794 w1816]
          tunnel: w1677 -> [w1683 w1705 w1727 w1749 w1771 w1793 w1815]
          tunnel: [w1681 _ _ _ _ _ _] -> w1676
          tunnel: w1675 -> [w1680 _ _ _ _ _ _]
          tunnel: [w1680 _ _ _ _ _ _] -> w1674
          tunnel: "cryostatus_" ("string") -> [w1679 w1702 w1724 w1746 w1768 w1790 w1812]
          frame #0 {
            n815 = flat-sequence {
              tunnel: w1683 -> [w1686]
              tunnel: [w1686] -> w1682
              tunnel: w1684 -> [w1701]
              tunnel: w1682 -> [w1689]
              tunnel: [w1688] -> w1681
              tunnel: w1679 -> [w1687]
              frame #0 {
                n816 = property class="TabCtl (strict)"("Val(Sgnl)"=T1."NI USB CONFIG" ("Value (Signaling)")) -> ()  [unwired: 2 in, 2 out]
              }
              frame #1 {
                w1699 = "_" ("string")
                n817 = local read "Cycle #"() -> (w1697:u32)
                n818 = call "LV_UNIXTIME.vi"("current time"=w1689) -> ("date/time string"=w1700:string)  [unwired: 9 in, 1 out]
                n819 = Format Value(format string="%06d", value (0)=w1697) -> (output string=w1696:string)  [unwired: 1 in]
                n820 = Concatenate Strings(w1687, w1700, w1699, w1696, w1699, "page1.png" ("string")) -> (w1694:string)
                n821 = invoke class="TabCtl (strict)" method="Get Image"(error in=errorcluster {"status"=FALSE, "code"=0, "source"=""} ("error in (no error)")) -> (error out=w1690:errorcluster, "image data"=w1692:T25)  [unwired: 5 in, 4 out]
                n822 = Build Path(base path=w1701, name or relative path=w1694) -> (appended path=w1693:path)
                n823 = call <vilib>:"Write PNG File.vi"("error in (no error)"=w1690, "image data"=w1692, "path to PNG file"=w1693) -> ("error out"=w1688:errorcluster)  [unwired: 7 in, 1 out]
              }
            }
          }
          frame #1 {
            n824 = flat-sequence {
              tunnel: w1705 -> [w1708]
              tunnel: [w1708] -> w1704
              tunnel: w1706 -> [w1723]
              tunnel: w1704 -> [w1711]
              tunnel: [w1710] -> w1703
              tunnel: w1702 -> [w1709]
              frame #0 {
                n825 = property class="TabCtl (strict)"("Val(Sgnl)"=T1."LSI CONFIG" ("Value (Signaling)")) -> ()  [unwired: 2 in, 2 out]
              }
              frame #1 {
                w1721 = "_" ("string")
                n826 = local read "Cycle #"() -> (w1719:u32)
                n827 = call "LV_UNIXTIME.vi"("current time"=w1711) -> ("date/time string"=w1722:string)  [unwired: 9 in, 1 out]
                n828 = Format Value(format string="%06d", value (0)=w1719) -> (output string=w1718:string)  [unwired: 1 in]
                n829 = Concatenate Strings(w1709, w1722, w1721, w1718, w1721, "page2.png" ("string")) -> (w1716:string)
                n830 = invoke class="TabCtl (strict)" method="Get Image"(error in=errorcluster {"status"=FALSE, "code"=0, "source"=""} ("error in (no error)")) -> (error out=w1712:errorcluster, "image data"=w1714:T25)  [unwired: 5 in, 4 out]
                n831 = Build Path(base path=w1723, name or relative path=w1716) -> (appended path=w1715:path)
                n832 = call <vilib>:"Write PNG File.vi"("error in (no error)"=w1712, "image data"=w1714, "path to PNG file"=w1715) -> ("error out"=w1710:errorcluster)  [unwired: 7 in, 1 out]
              }
            }
            n833 = local write "error out (frontpanel screenshots)"(w1703) -> ()
          }
          frame #2 {
            n834 = flat-sequence {
              tunnel: w1727 -> [w1730]
              tunnel: [w1730] -> w1726
              tunnel: w1728 -> [w1745]
              tunnel: w1726 -> [w1733]
              tunnel: [w1732] -> w1725
              tunnel: w1724 -> [w1731]
              frame #0 {
                n835 = property class="TabCtl (strict)"("Val(Sgnl)"=T1."MEASUREMENT" ("Value (Signaling)")) -> ()  [unwired: 2 in, 2 out]
              }
              frame #1 {
                w1743 = "_" ("string")
                n836 = local read "Cycle #"() -> (w1741:u32)
                n837 = call "LV_UNIXTIME.vi"("current time"=w1733) -> ("date/time string"=w1744:string)  [unwired: 9 in, 1 out]
                n838 = Format Value(format string="%06d", value (0)=w1741) -> (output string=w1740:string)  [unwired: 1 in]
                n839 = Concatenate Strings(w1731, w1744, w1743, w1740, w1743, "page3.png" ("string")) -> (w1738:string)
                n840 = invoke class="TabCtl (strict)" method="Get Image"(error in=errorcluster {"status"=FALSE, "code"=0, "source"=""} ("error in (no error)")) -> (error out=w1734:errorcluster, "image data"=w1736:T25)  [unwired: 5 in, 4 out]
                n841 = Build Path(base path=w1745, name or relative path=w1738) -> (appended path=w1737:path)
                n842 = call <vilib>:"Write PNG File.vi"("error in (no error)"=w1734, "image data"=w1736, "path to PNG file"=w1737) -> ("error out"=w1732:errorcluster)  [unwired: 7 in, 1 out]
              }
            }
            n843 = local write "error out (frontpanel screenshots)"(w1725) -> ()
          }
          frame #3 {
            n844 = flat-sequence {
              tunnel: w1749 -> [w1752]
              tunnel: [w1752] -> w1748
              tunnel: w1750 -> [w1767]
              tunnel: w1748 -> [w1755]
              tunnel: [w1754] -> w1747
              tunnel: w1746 -> [w1753]
              frame #0 {
                n845 = property class="TabCtl (strict)"("Val(Sgnl)"=T1."HE AUTO FILL" ("Value (Signaling)")) -> ()  [unwired: 2 in, 2 out]
              }
              frame #1 {
                w1765 = "_" ("string")
                n846 = local read "Cycle #"() -> (w1763:u32)
                n847 = call "LV_UNIXTIME.vi"("current time"=w1755) -> ("date/time string"=w1766:string)  [unwired: 9 in, 1 out]
                n848 = Format Value(format string="%06d", value (0)=w1763) -> (output string=w1762:string)  [unwired: 1 in]
                n849 = Concatenate Strings(w1753, w1766, w1765, w1762, w1765, "page4.png" ("string")) -> (w1760:string)
                n850 = invoke class="TabCtl (strict)" method="Get Image"(error in=errorcluster {"status"=FALSE, "code"=0, "source"=""} ("error in (no error)")) -> (error out=w1756:errorcluster, "image data"=w1758:T25)  [unwired: 5 in, 4 out]
                n851 = Build Path(base path=w1767, name or relative path=w1760) -> (appended path=w1759:path)
                n852 = call <vilib>:"Write PNG File.vi"("error in (no error)"=w1756, "image data"=w1758, "path to PNG file"=w1759) -> ("error out"=w1754:errorcluster)  [unwired: 7 in, 1 out]
              }
            }
            n853 = local write "error out (frontpanel screenshots)"(w1747) -> ()
          }
          frame #4 {
            n854 = flat-sequence {
              tunnel: w1771 -> [w1774]
              tunnel: [w1774] -> w1770
              tunnel: w1772 -> [w1789]
              tunnel: w1770 -> [w1777]
              tunnel: [w1776] -> w1769
              tunnel: w1768 -> [w1775]
              frame #0 {
                n855 = property class="TabCtl (strict)"("Val(Sgnl)"=T1."VALVE CTRL" ("Value (Signaling)")) -> ()  [unwired: 2 in, 2 out]
              }
              frame #1 {
                w1787 = "_" ("string")
                n856 = local read "Cycle #"() -> (w1785:u32)
                n857 = call "LV_UNIXTIME.vi"("current time"=w1777) -> ("date/time string"=w1788:string)  [unwired: 9 in, 1 out]
                n858 = Format Value(format string="%06d", value (0)=w1785) -> (output string=w1784:string)  [unwired: 1 in]
                n859 = Concatenate Strings(w1775, w1788, w1787, w1784, w1787, "page5.png" ("string")) -> (w1782:string)
                n860 = invoke class="TabCtl (strict)" method="Get Image"(error in=errorcluster {"status"=FALSE, "code"=0, "source"=""} ("error in (no error)")) -> (error out=w1778:errorcluster, "image data"=w1780:T25)  [unwired: 5 in, 4 out]
                n861 = Build Path(base path=w1789, name or relative path=w1782) -> (appended path=w1781:path)
                n862 = call <vilib>:"Write PNG File.vi"("error in (no error)"=w1778, "image data"=w1780, "path to PNG file"=w1781) -> ("error out"=w1776:errorcluster)  [unwired: 7 in, 1 out]
              }
            }
            n863 = local write "error out (frontpanel screenshots)"(w1769) -> ()
          }
          frame #5 {
            n864 = flat-sequence {
              tunnel: w1793 -> [w1796]
              tunnel: [w1796] -> w1792
              tunnel: w1794 -> [w1811]
              tunnel: w1792 -> [w1799]
              tunnel: [w1798] -> w1791
              tunnel: w1790 -> [w1797]
              frame #0 {
                n865 = property class="TabCtl (strict)"("Val(Sgnl)"=T1." DIAGRAM" ("Value (Signaling)")) -> ()  [unwired: 2 in, 2 out]
              }
              frame #1 {
                w1809 = "_" ("string")
                n866 = local read "Cycle #"() -> (w1807:u32)
                n867 = call "LV_UNIXTIME.vi"("current time"=w1799) -> ("date/time string"=w1810:string)  [unwired: 9 in, 1 out]
                n868 = Format Value(format string="%06d", value (0)=w1807) -> (output string=w1806:string)  [unwired: 1 in]
                n869 = Concatenate Strings(w1797, w1810, w1809, w1806, w1809, "page6.png" ("string")) -> (w1804:string)
                n870 = invoke class="TabCtl (strict)" method="Get Image"(error in=errorcluster {"status"=FALSE, "code"=0, "source"=""} ("error in (no error)")) -> (error out=w1800:errorcluster, "image data"=w1802:T25)  [unwired: 5 in, 4 out]
                n871 = Build Path(base path=w1811, name or relative path=w1804) -> (appended path=w1803:path)
                n872 = call <vilib>:"Write PNG File.vi"("error in (no error)"=w1800, "image data"=w1802, "path to PNG file"=w1803) -> ("error out"=w1798:errorcluster)  [unwired: 7 in, 1 out]
              }
            }
            n873 = local write "error out (frontpanel screenshots)"(w1791) -> ()
          }
          frame #6 {
            n874 = flat-sequence {
              tunnel: w1815 -> [w1818]
              tunnel: [w1818] -> w1814
              tunnel: w1816 -> [w1833]
              tunnel: w1814 -> [w1821]
              tunnel: [w1820] -> w1813
              tunnel: w1812 -> [w1819]
              frame #0 {
                n875 = property class="TabCtl (strict)"("Val(Sgnl)"=T1."(Place holder)" ("Value (Signaling)")) -> ()  [unwired: 2 in, 2 out]
              }
              frame #1 {
                w1831 = "_" ("string")
                n876 = local read "Cycle #"() -> (w1829:u32)
                n877 = call "LV_UNIXTIME.vi"("current time"=w1821) -> ("date/time string"=w1832:string)  [unwired: 9 in, 1 out]
                n878 = Format Value(format string="%06d", value (0)=w1829) -> (output string=w1828:string)  [unwired: 1 in]
                n879 = Concatenate Strings(w1819, w1832, w1831, w1828, w1831, "page7.png" ("string")) -> (w1826:string)
                n880 = invoke class="TabCtl (strict)" method="Get Image"(error in=errorcluster {"status"=FALSE, "code"=0, "source"=""} ("error in (no error)")) -> (error out=w1822:errorcluster, "image data"=w1824:T25)  [unwired: 5 in, 4 out]
                n881 = Build Path(base path=w1833, name or relative path=w1826) -> (appended path=w1825:path)
                n882 = call <vilib>:"Write PNG File.vi"("error in (no error)"=w1822, "image data"=w1824, "path to PNG file"=w1825) -> ("error out"=w1820:errorcluster)  [unwired: 7 in, 1 out]
              }
            }
            n883 = local write "error out (frontpanel screenshots)"(w1813) -> ()
          }
        }
        "error out (frontpanel screenshots)" <- w1676
        n884 = property class="TabCtl (strict)"("Val(Sgnl)"=w1674) -> ()  [unwired: 2 in, 2 out]
      }
      event "Stop Button": Value Change {
        n885 = event-data() -> ()  [unwired: 1 in, 3 out]
      }
    }
  }
  n886 = call-dynamic "USBData_terminate.vi"("error in (no error)"=w23, "USBData in"=w24) -> ("error out"=w25:errorcluster)  [unwired: 8 in, 1 out]
  n887 = call-dynamic "LSI336Data_terminate.vi"("error in (no error)"=w13, "LSI336Data in"=w14) -> ("error out"=w12:errorcluster)  [unwired: 8 in, 1 out]
  n888 = call-dynamic "USBData_terminate.vi"("error in (no error)"=w6, "USBData in"=w7) -> ("error out"=w8:errorcluster)  [unwired: 8 in, 1 out]
  n889 = call "LSI218Data_terminate.vi"("error in (no error)"=w17, "LSI218Data in"=w18) -> ("error out"=w16:errorcluster)  [unwired: 8 in, 1 out]
  n890 = local write "error out (USB6210)"(w25) -> ()
  n891 = local write "error out (LSI336)"(w12) -> ()
  n892 = local write "error out (USB6210)"(w8) -> ()
  n893 = local write "error out (LSI218)"(w16) -> ()
